vi "Main.vi"() -> ()   [LabVIEW 2018]
doc: "The myRIO Project template acquires acceleration data from the onboard accelerometer and displays the changes of acceleration values in a waveform chart."
uses:
  <vilib>/myRIO/Instrument Drivers/Utilities/Utilities.lvlib
  <vilib>/Platform/TimedLoop/XDataNode/XDataNode.xnode
  <vilib>/Platform/TimedLoop/XDataNode/nitl_modes.ctl
  <vilib>/Platform/TimedLoop/XDataNode/XDNodeRunTimeDep.lvlib
  <vilib>/Platform/TimedLoop/XDataNode/wakeup.ctl
  <vilib>/Platform/TimedLoop/XDataNode/timing_clust.ctl
  <vilib>/robotics/Steering/Steering Frame/NI_Robotics_Steering Frame.lvclass
  <vilib>/robotics/Steering/Wheel/NI_Robotics_Wheel.lvclass
  <vilib>/robotics/Steering/Wheel/Rotation Direction.ctl
  <vilib>/robotics/Steering/Wheel/Wheel Parameters.ctl
  <vilib>/addons/control/pid/NI_PID_pid.lvlib
  C:/Work/WRO/LidarCar/LidarCar/Operator Loop/Operator Loop Mode.ctl
  Operator Loop/Operator Loop Mode.ctl
  <vilib>/myRIO/Express VI/Onboard Devices/LED/LED Express VI.xnode
  <vilib>/myRIO/Instrument Drivers/Onboard IO/DIO/vis/Write.vi
  <vilib>/myRIO/Instrument Drivers/Onboard IO/DIO/DIO.lvlib
  <vilib>/myRIO/Common/Instrument Driver Framework/myRIO v1.0/DIO/typedefs/DIO Channels Enum.ctl
  <vilib>/myRIO/Common/Instrument Driver Framework/myRIO v1.0/DIO/typedefs/DIO Channels List.ctl
  <vilib>/myRIO/Common/Instrument Driver Framework/Utilities/typedefs/Generic FPGA Reference.ctl
  <vilib>/myRIO/Common/Instrument Driver Framework/Utilities/typedefs/myRIO v1.0 Reference.ctl
  <vilib>/myRIO/Common/Instrument Driver Framework/Utilities/typedefs/Hardware Version Enum.ctl
  <vilib>/myRIO/Common/Instrument Driver Framework/Utilities/typedefs/myRIO Generic Hardware Reference.ctl
  <vilib>/myRIO/Instrument Drivers/Onboard IO/DIO/typedefs/DIO Reference.ctl
  <vilib>/myRIO/Instrument Drivers/Onboard IO/DIO/vis/myRIO DIO Open.xnode
  <vilib>/myRIO/Common/Instrument Driver Framework/Utilities/vis/Is FPGA Ref Available.vi
  <vilib>/myRIO/Common/Instrument Driver Framework/myRIO v1.0/DIO/vis/myRIO v1.1 Open DIO.vi
  <vilib>/userdefined/High Color/nirio_resource_hc.ctl
  <vilib>/addons/control/pid/pid.llb/PID (DBL).vi
  <vilib>/Analysis/NI_AALPro.lvlib
  <vilib>/Analysis/coordinate.llb/2D Cartesian Coordinate Rotation (Scalar).vi
  <vilib>/myRIO/Express VI/Onboard Devices/Button/Button Express VI.xnode
  <vilib>/myRIO/Instrument Drivers/Onboard IO/DIO/vis/Read.vi
  <vilib>/myRIO/Instrument Drivers/Onboard IO/PWM/typedefs/PWM Configuration.ctl
  <vilib>/myRIO/Instrument Drivers/Onboard IO/PWM/PWM.lvlib
  <vilib>/myRIO/Common/Instrument Driver Framework/myRIO v1.0/PWM/typedefs/PWM Channels Enum.ctl
  <vilib>/myRIO/Instrument Drivers/Onboard IO/PWM/typedefs/PWM Reference.ctl
  <vilib>/myRIO/Instrument Drivers/Onboard IO/PWM/vis/Set Duty Cycle and Frequency.vi
  <vilib>/myRIO/Common/Instrument Driver Framework/myRIO v1.0/PWM/vis/myRIO v1.1 Open PWM.vi
  <vilib>/myRIO/Instrument Drivers/Onboard IO/PWM/vis/myRIO PWM Open.xnode
  <vilib>/myRIO/Express VI/Onboard IO/PWM/PWM Express VI.xnode
  <vilib>/vision/driver/NI_Vision_Acquisition_Software.lvlib
  <vilib>/myRIO/Express VI/Onboard IO/DI/DI Express VI.xnode
  <vilib>/myRIO/Express VI/Onboard IO/DO/DO Express VI.xnode
  <vilib>/robotics/Steering/Steering Frame/Create User Defined Steering Frame.vi
  <vilib>/robotics/Steering/Omnidirectional Wheel/Create Omnidirectional Wheel.vi
  <vilib>/robotics/Steering/Omnidirectional Wheel/NI_Robotics_Omnidirectional Wheel.lvclass
  <vilib>/robotics/Steering/Steering Frame/Apply Steering Frame Velocity to Motors.vi
  C:/Program Files (x86)/National Instruments/LabVIEW 2018/vi.lib/robotics/Steering/Wheel/NI_Robotics_Wheel.lvclass
  Type Definitions/Measurement Type.ctl
  Type Definitions/Acquisition Parameters.ctl
  <vilib>/userdefined/High Color/IMAQdx.ctl
panel:
  out "nowpos":dbl=-11.367150887839898
  out "OffsetZero":i32=-11
  in  "get over":bool
  out "B/DIO0 (Pin 11)":bool
  out "Lidar mid":i32=90
  in  "Light ON":bool
  in  "Load Image":bool
  in  "Select Image":string(combo)="A1"
  out "GoFarSec":u64
  out "min Distance":dbl=0.17274696726012956
  out "Image Out":T1(plugin-control)
  out "nearwall":bool
  out "Proc Down Color":i32=4
  in  "no get":bool
  in  "Enable US":bool=TRUE
  out "LD Range":dbl=119.77184676592617
  out "Block Face":dbl
  out "FX":dbl=518.7986455361987
  out "FXindex":i32=4
  out "FYindex":i32=14
  out "FXArr":dbl[](array[numeric])=[0.0, 518.7986455361987, 517.3027702585492, 515.9611019967892, 519.7944156608107]
  out "FYArr":dbl[](array[numeric])=[1569.0472275400712, 1569.0472275400712, 1561.3708676606448, 1566.6278937272687, 1557.2876598848363]
  out "FY":dbl=1569.0472275400712
  in  "Light Set":dbl=0.7
  out "Offset":dbl[](array[numeric])=[0.05, -3.061616997868383e-18]
  in  "Enable ND":bool
  in  "Set Test SubGoal":bool
  out "Put Counter":i32
  in  "Session In":T2="cam1"
  in  "Light":dbl
  out "ucolor":i32=4
  out "dcolor":i32=5
  in  "Color Disable":bool
  in  "URG-30LX":bool=TRUE
  in  "UBG-04FX Parameters":T3={"Starting Step"=44, "Ending Step"=725, "Cluster Count"=9, "Scan Interval"=0, "Number of Scans"=0, "Measurement Type"=enum."MS"}
  in  "Run Catch":bool
  in  "Get off/Put on":bool=TRUE
  in  "Test Catch":i16 min=0 max=3
  out "SubGoal":dbl[](array[numeric])=[0.588553326542981, 1.5637625506524007, 0.027695235097022965]
  in  "BL Range":dbl=106.0
  out "UltraSound":dbl=99.0
  in  "Set Z Offset":bool
  out "ODM Global Lidar":cluster{dbl[], dbl[]}[](graph)=[{[721.8291590825777], [795.7789827798357]}, {[0.0, 173.38729628759307, 225.66665610466003, 267.75647202793164, 307.78375775869426, 345.4796863667954, 386.0601693720772, 425.84303948753245, 461.38885484188586, 494.6121667989658, 530.892312288831, 564.3483818227398, 598.9442921444596, 631.7209869860719, 663.8971291981472, 695.8658767767539, 727.1715466499368, 758.8645020637247, 786.3860165375595, 804.3005854950422, 822.6493543934826, 841.0683200841246, 859.4613632147373, 878.918441734572, 896.3207994504536, 915.856172199784, 935.636054026129, 956.693854559551, 978.1414574666462, 997.7919082944074, 1021.5668180947448, 1129.0848273862223, 1140.3421474627507, 1167.0238039986898, 1197.8060920596474, 1237.6798928632963, 1274.67547579493, 1313.6442770102278, 1351.7890598592828, 1601.7296724745213, 1701.59915067344, 1790.471940105315, 1890.3533021616595, 1975.681444325002, 2080.8834474418536, 2199.916399964641, 2288.3422835710217, 2269.044100856724, 2269.913362880439, 2275.262737598881, 2273.0619560851524, 2271.883597560387, 2273.867229333762, 2276.270813184838, 2283.1501466095037, 2281.7136074144396, 2280.8814360333404, 2287.701288915185, 2057.221659783369, 2055.6828792476545, 2062.1389602013965, 2058.6161638397925, 2055.0754422563373, 2156.1814882136705, 2091.396440925394, 1945.0381394296392, 1934.4975767345456, 1929.5528957285972, 1928.0192875117154, 1928.679460770824, 1934.7695441247085, 2273.4555279831993, 2244.567273948284, 1420.8784222522072, 1338.2032680954792, 1274.032736829724, 1215.8750320799377, 1165.7538524389452, 1130.9140787661042, 1116.611145793328, 1108.8419935326024, 1098.073782898878, 1090.3710419336774, 1087.2408194244206, 1072.1815861120838, 1064.3437362068323, 1052.1947093007082, 1043.6027163222507, 1034.9198885950275, 1020.989821141792, 1147.510042165152, 1185.4766822006893, 1123.9684076830076, 1063.326429163897, 1003.3034354850358, 942.6873919372472, 883.4901954196058, 823.9725320994982, 764.5128057343941, 705.1514377393997, 645.8853239946892, 585.7997376242854, 526.0621283065328, 464.34896817814956, 404.24666324255236, 342.0883282079875, 277.0716342023713, 212.69592369267963], [0.0, -1.1322564017730496, 4.966756080453739, 0.5077440499308005, -4.454468226445895, -11.021670601286585, -9.596364902480591, -6.2440935839171, -9.378372326349291, -16.613562940879945, -12.932345500497807, -15.388120696622703, -10.61269028937555, -10.276165299446717, -10.586494828388973, -9.608611783836272, -13.34567042737981, -7.855848584257861, 328.8560921706781, 331.40708435844897, 327.682033403894, 326.68504208099455, 327.41527128271883, 323.9888902290291, 331.08814597563986, 330.199640851444, 330.14966222571655, 328.1530339444062, 327.11711529750204, 331.58647253289155, 328.92067367243607, 182.64222973992665, 216.23913279752037, 224.17363585313913, 227.71482426419658, 221.92474990792795, 222.95568299997052, 224.59211265082112, 229.84383762917457, 46.1196506252172, 19.290037227608405, 10.236768574542058, 0.6806810112642081, 8.771460166297727, 11.11763649590324, 13.887670225470854, 40.869048984587245, 121.85683290565059, 190.46182338990178, 255.40765812456652, 321.33540980144414, 385.21578219972656, 446.9407541050027, 507.6435863509478, 566.9883190305765, 627.0796755525192, 686.5140152469784, 745.3526744488408, 801.9668274705773, 852.0483763075719, 902.9259095939335, 953.3797430047575, 1004.0687823188368, 1077.182165623156, 1117.7495796008423, 1130.0011651866287, 1176.7036525019564, 1225.956066917477, 1277.770631563482, 1332.2729192505776, 1391.7418162789627, 1645.3317728813229, 1706.9758198210902, 1225.5086611026113, 1201.9471543380675, 1185.1985794784985, 1167.3981152418305, 1151.1958156005373, 1145.277200975239, 1158.7274049891116, 1180.048820376938, 1198.942700206554, 1223.2944316784685, 1256.8697159243388, 1274.5279241498613, 1306.6412141486715, 1334.377137334104, 1373.7982904308146, 1419.8389496097002, 1460.39373731479, 1958.9040004476574, 2284.203937575801, 2288.1943216415884, 2292.6275978401427, 2297.5929521065086, 2294.2073833976106, 2300.379784341795, 2301.2264246197224, 2302.7349037113363, 2298.9104379767673, 2294.7558697296113, 2296.21136858921, 2291.316732701449, 2293.83689238431, 2285.0809925529366, 2281.5956696474964, 2283.099714055563, 2278.034076178987]}, {[0.0, 0.0, 2300.0, 2300.0, 0.0], [0.0, 2300.0, 2300.0, 0.0, 0.0]}, {[115.0, 115.0, 2185.0, 2185.0, 115.0], [115.0, 2185.0, 2185.0, 115.0, 115.0]}, {[1.2743751839684945], [1.349012436815834]}, {[1.1606747746939823], [1.7455328863903905]}, {[903.9764173161522, 1240.4369436227526, 2170.0754422563373, -115.0, 2043.0192875117154, -115.0, -115.0], [216.58647253289155, 114.84383762917457, 903.0178048947071, 0.0, 1260.8714907327958, 0.0, 0.0]}, {[436.58676528880187, 903.9378283810288, 1240.4213885973015, 2167.4413707572576, 2041.974666138485], [796.903102586175, 217.61848380592934, 113.82095487507502, 902.8249826773058, 1259.8777188454835]}]
  out "Odometry Data":dbl[](array[numeric])=[0.5140081874058262, 1.5687256004107921, 0.036230187244589505]
  in  "Reset Start POS":bool
  in  "Set Start POS":bool
  out "X Find":dbl=519.7944156608107
  out "XL Dots":dbl=36.0
  out "XR Dots":dbl=2.0
  out "XR Find":dbl=513.9748126879588
  out "SEC":u64
  out "MIN":u64
  out "Angle Find":dbl=0.017453292519943295
  out "Y Find":dbl=1551.5711689987047
  out "XL Find":dbl=525.6140186336626
  out "Down Color":i32
  out "Up Color":i32
  out "Right Block":bool
  out "Left Block":bool
  out "Proc Time":i16=173
  out "Proc Index":i16=25
  in  "Proc  VAL B":i32
  in  "Proc  VAL A":i32
  in  "Proc CMD":i16=99
  out "Block Array":dbl[][](array[numeric])
  out "Proc Finish":bool=TRUE
  out "Proc Catch Index":i16
  out "Proc Block Index":i16
  out "Block Color":i16[][](array[numeric])
  out "Catch Color":i16[](array[numeric])
  in  "Timer Run":bool
  out "Z offset":dbl
  in  "-X":bool
  in  "+X":bool
  in  "-Y":bool
  in  "+Y":bool
  out "Sensor z":dbl=-0.7583617520109639
  in  "Z Sensor resource":refnum<visa-resource-name>="ASRL2::INSTR"
  in  "QR_CAM":bool=TRUE
  in  "Set SubGoal":bool
  in  "RC servo resource":refnum<visa-resource-name>="ASRL1::INSTR"
  out "Start Out Point":dbl[](array[numeric])=[0.5218091856466301, 1.3965735001255937]
  out "Block Fix array":dbl[](array[numeric])
  out "Target Distance":dbl=0.17274696726012956
  in  "PLAY":bool
  out "Start POS":dbl[](array[numeric])=[0.5259977631915781, 1.1566100532880597, -3.12413936106985]
  out "Start Front":dbl[](array[numeric])=[0.5187986455361987, 1.569047227540071, -3.12413936106985]
  in  "Block Find":bool
  in  "Show Lidar":bool
  in  "Robot Mode:":T5(ring)
  in  "max speed":dbl=0.67
  in  "inner threshold":dbl=0.2
  in  "outer threshold":dbl=0.5
  out "LIDAR data":cluster{dbl[], dbl[]}[](graph)
  out "VY History 2":dbl(graph)
  out "Heading History 2":dbl(graph)
  in  "Show VFH":bool
  out "Distance":i32[](array[numeric])
  out "Lidar Data":cluster{"angles (deg)":dbl[], "distances":dbl[]}(graph)={"angles (deg)"=[0.0, 433.8787272960038, 477.8933242300426, 527.1098060603185, 577.9196711836571, 638.569011724086, 712.0914573803195, 804.449757554414, 947.9078296932058, 1156.1704640673584, 1436.9407341066774, 1782.6178607501113, 443.13319277072446, 436.4011066877488, 428.963246529249, 428.85299241451406, 428.0814780693609, 436.59511206667196, 432.4776560401959, 429.6823946054481, 435.9780172673052, 437.56439930894794, 429.758975005734, 431.7298029202177, 428.18120387395703, 232.04054624122062, 174.89018459887424, 171.36933696908324, 152.11493483575714, 138.38064371099495, 125.76279949489856, 118.20964770339404, 109.94438198650472, 103.29713074135779, 95.98446041890367, 88.79774026449425, 82.41822688750861, 75.5184469259805, 68.80732906562578, 64.0039047725061, 58.16398223480165, 54.49999999999999, 47.492681073161364, 43.051109680829505, 39.86912949481099, 36.55353085362063, 31.179628134406673, 27.54948843628049, 23.138409544725345, 19.127875555233857, 16.257552369506364, 11.74735729980464, 8.235145679706214, 4.814907974350832, 1.2042427925636885, -2.460633140940076, -6.344103535323877, -10.034732473694731, -13.201321223188495, -17.130139396261864, -20.3041640219781, -25.10544737494451, -28.764532772630385, -34.71591336031218, -45.94912225121969, -110.22563027354184, -185.31896120176154, -239.53369765032343, -265.3611116739901, -461.85390169274285, -472.10476545045714, -477.8777217718457, -480.8581294893997, -485.1196896101722, -484.266579130126, -487.4515773202573, -484.93667582394033, -486.49337187206373, -483.95730286540066, -492.0033346073434, -489.67640876660056, -492.76845475334557, -489.3981635170621, -492.8115652550238, -492.4720886398095, -491.9968847640253, -488.61594681947446, -490.91570425251484, -493.338533040738, -492.98639076983807, -490.8069174109227, -490.76520638003615, -495.91085393218157, -488.3298424949866, -490.95793483883745, -490.8317465629986, -494.93802592634734, -491.29381631192706, -489.8774364757368, -488.67768905928546, -490.5971872157819, -487.7925422759795, -492.7902913399083, -493.0014998412093, -488.55382481063214, -486.91972892350634, -469.9613165631287, -436.7721049929968, 0.0], "distances"=[0.0, -250.4999999999999, -251.43184097556016, -251.41848053604448, -248.29388566570398, -245.12367748898538, -241.72247790797735, -238.2888742065911, -240.7379205823552, -245.7516185465913, -246.91157661187788, -234.68609361165238, -40.71822030521407, -22.870812878166458, -5.615436500106674, 11.229910824077672, 28.057942439731367, 45.887995374499866, 62.70627581014535, 79.63692464006853, 98.65175345461108, 117.2450274314419, 133.44370873900692, 152.88354152906706, 170.82697869203457, 103.31110734125329, 86.24629459270524, 93.04595825062364, 90.4988762356382, 89.86544077747949, 88.880359265734, 90.70545292229937, 91.4397772832236, 93.0091542838813, 93.50392161878514, 93.57329386058511, 93.97997593487217, 93.25751537483652, 92.14418845947198, 93.12625931428776, 92.18433256573309, 94.39676901250382, 90.26873902123027, 90.25852843498606, 92.79791222503873, 95.22520350271458, 91.85222256102526, 93.00551428221473, 91.10770551243492, 89.98957926751012, 94.61338166957546, 89.23003752364293, 89.62244348171956, 91.8739171974208, 91.99211813680864, 93.96778854770238, 96.79231555414454, 95.47410195535423, 91.04792758740966, 92.42596131101173, 89.73149348678317, 93.69480515003963, 92.6369346123471, 98.03471507358655, 115.1723845561186, 247.57081902114484, 375.7896787021964, 441.1661905563066, 446.0319275692539, 711.1926416177196, 668.0127921222534, 622.7823721286196, 578.1690577192416, 538.7799984711108, 497.11354873671013, 462.5742748662027, 425.2780507395445, 393.95456479719826, 361.38805874467806, 338.1445234441252, 308.96280471513904, 284.50000000000006, 257.4848297397867, 235.0590588573292, 211.5827070219672, 188.85990941037318, 165.86276409643145, 145.41585648840845, 125.29202615175753, 104.78749217215065, 84.33605291681421, 64.6104651489256, 45.567806094374454, 25.5922826027996, 6.426991425530077, -12.852881619165652, -32.439952098151, -51.63706085422075, -71.02884788563368, -90.57105616959733, -111.01080981581498, -130.70361777677303, -153.01545268739454, -174.58098737926213, -194.9132121301739, -216.7906307594014, -231.7592736747566, -237.1479038490254, 0.0]} caption="Global Lidar Data"
  out "Lidar Array Size":dbl=107.0
  out "Angle":dbl[](array[numeric])=[-120.0, -117.75, -115.5, -113.25, -111.0, -108.75, -106.5, -104.25, -102.0, -99.75, -97.5, -95.25, -93.0, -90.75, -88.5, -86.25, -84.0, -81.75, -79.5, -77.25, -75.0, -72.75, -70.5, -68.25, -66.0, -63.75, -61.5, -59.25, -57.0, -54.75, -52.5, -50.25, -48.0, -45.75, -43.5, -41.25, -39.0, -36.75, -34.5, -32.25, -30.0, -27.75, -25.5, -23.25, -21.0, -18.75, -16.5, -14.25, -12.0, -9.75, -7.5, -5.25, -3.0, -0.75, 1.5, 3.75, 6.0, 8.25, 10.5, 12.75, 15.0, 17.25, 19.5, 21.75, 24.0, 26.25, 28.5, 30.75, 33.0, 35.25, 37.5, 39.75, 42.0, 44.25, 46.5, 48.75, 51.0, 53.25, 55.5, 57.75, 60.0, 62.25, 64.5, 66.75, 69.0, 71.25, 73.5, 75.75, 78.0, 80.25, 82.5, 84.75, 87.0, 89.25, 91.5, 93.75, 96.0, 98.25, 100.5, 102.75, 105.0, 107.25, 109.5, 111.75, 114.0, 116.25, 118.5]
  in  "URG-04LX Resource":refnum<visa-resource-name>="ASRL3::INSTR"
  in  "URG-30LX Parameters":T3={"Starting Step"=60, "Ending Step"=1020, "Cluster Count"=9, "Scan Interval"=0, "Number of Scans"=0, "Measurement Type"=enum."MS"}
  out "Now POS":cluster{"X":dbl, "Y":dbl, "Angle":dbl}={"X"=514.0081874058262, "Y"=1568.7256004107921, "Angle"=2.075836820083688}
  in  "Enable":bool=TRUE caption="Enable Motor"
  in  "X Velocity (m/s)":dbl(slide) min=-1.0 max=1.0 scale=-0.5..0.5
  in  "Y Velocity (m/s)":dbl(slide) min=-1.0 max=1.0 scale=-0.5..0.5
  in  "Heading(rad)":dbl(slide) min=-10.0 max=10.0 scale=10.0..-10.0
  out "X Velocity Feedback":dbl(slide) scale=-0.5..0.5
  out "Y Velocity Feedback":dbl(slide)=-0.0 scale=-0.5..0.5
  out "Angular Velocity Feedback":dbl(slide) scale=10.0..-10.0
  in  "stop":bool=TRUE
  in  "PID gains":T6={"proportional gain (Kc)"=0.11, "integral time (Ti, min)"=0.001, "derivative time (Td, min)"=0.0} {"derivative time (Td, min)" format="%.5f"; "integral time (Ti, min)" format="%.3f"; "proportional gain (Kc)" format="%.3f"}
  out "ENC Val. mm":T7={"Numeric Control"=-13.769011552061516, "Numeric Control"=3.3657583793928145, "Numeric Control"=-3.059780344902559}
  in  "Reset Counter":bool
  in  "Encoder PPR":dbl=24.0
  in  "Gear Ratio":i32=64
  in  "R(mm)":dbl=37.4
  out "error out":errorcluster={"status"=FALSE, "code"=1073676294, "source"="VISA Read in URG-04LX-UG01 Read Measurement Data.vi->Main.vi"}
  # "0:x\n1:Green \n2:Red \n3:Yellow\n4:Blue\n5:Orange"
  # "2    0          1     3\n\\     /           \\     /"
  # "下      上        不處理"
  # "讀取QR CODE"
  # "執行程式"
  # "不看顏色,使用預設"
  # "不取方塊"
  # "設定Z軸偏移"
  # "地圖BX,地圖BY,座標Xmm,座標Ymm,下顏色,上顏色,FXm,FYm,FZrag,看到的次數(最多100)"
  # "顯示行走圖"
  # "按下使用遠距光達"
  # "用來修正世界座標\n及偏移值"
  # "測試取放方塊\n1.Block Correction -> Idle\n2.Set SubGoal\n3.選擇爪子\n4.選擇拿起(Get)或放下(Put,按下)\n5.按下Run Catch"
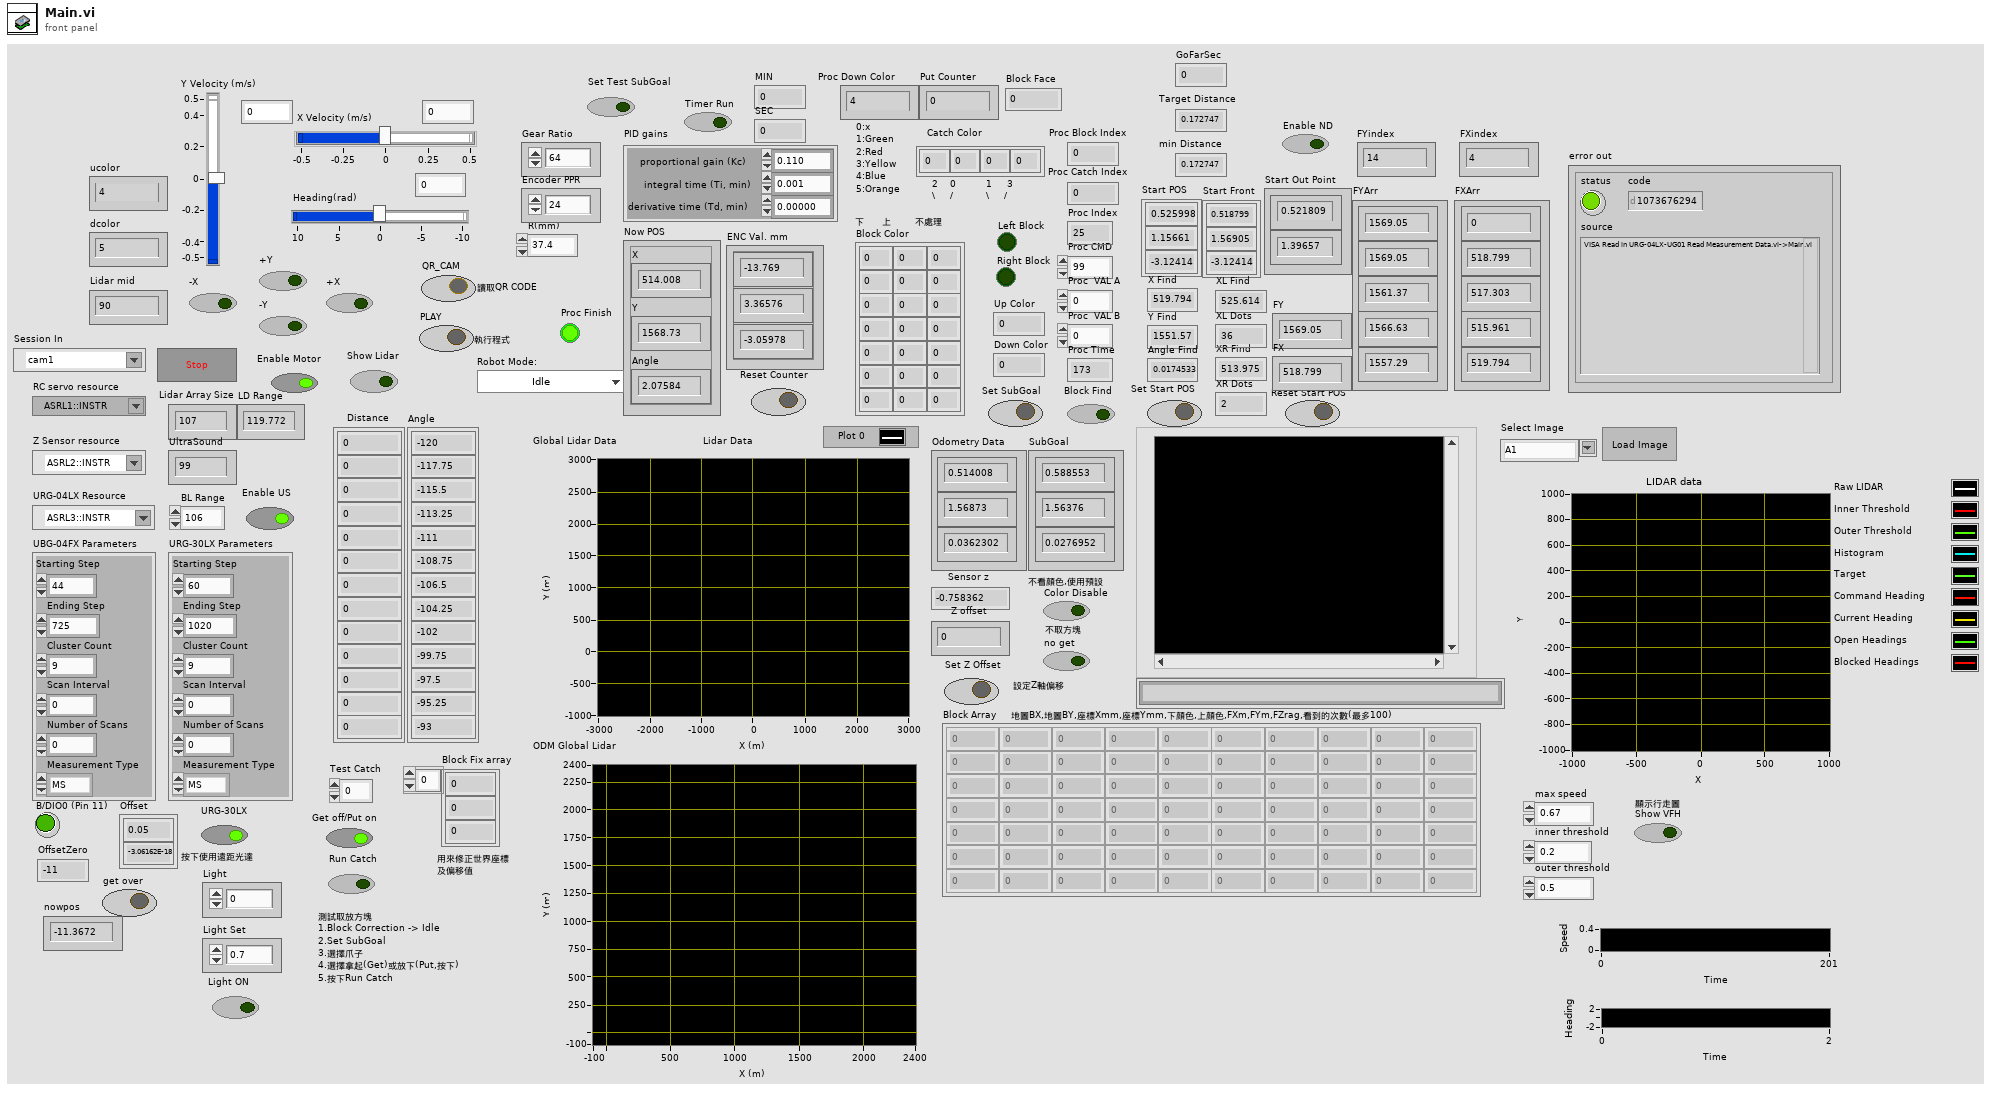
[diagram p1: front panel]
types:
  T1 = typedef "IMAQ Image.ctl" = refnum<image>
  T2 = typedef "IMAQdx.ctl" = refnum<k21>
  T3 = typedef "Acquisition Parameters.ctl" = cluster{"Starting Step":i32, "Ending Step":i32, "Cluster Count":i32, "Scan Interval":i32, "Number of Scans":i32, "Measurement Type":T4}
  T4 = typedef "Measurement Type.ctl" = enum16{"MD", "MS"}
  T5 = enum16{"Idle", "Tele-Op", "Path Following", "Go Target", "Wall Correction", "Positioning", "Block Correction", "Get Color", "WhereGo", "Home Correction", "RC Control", "MoveTarget", "moveblock", "hands up", "hands down", "readQR"}
  T6 = cluster{"proportional gain (Kc)":dbl, "integral time (Ti, min)":dbl, "derivative time (Td, min)":dbl}
  T7 = cluster{"Numeric Control":dbl, "Numeric Control":dbl, "Numeric Control":dbl}
  T8 = typedef "PWM.lvlib/PWM Reference.ctl" = cluster{"myRIO Reference":T9, "PWM Channels Enum":T13, "PWM Configuration":T14}
  T9 = typedef "myRIO Generic Hardware Reference.ctl" = cluster{"myRIO Model":T10, "myRIO Hardware Reference":T11}
  T10 = typedef "Hardware Version Enum.ctl" = enum16{"Unknown", "myRIO-1900", "myRIO-1950", "roboRIO", "NI ELVIS RIO CM", "ELVIS III"}
  T11 = typedef "myRIO v1.0 Reference.ctl" = cluster{"Generic FPGA Reference":T12, "Allow multiple opens":bool}
  T12 = typedef "Generic FPGA Reference.ctl" = refnum<k20>
  T13 = typedef "PWM Channels Enum.ctl" = enum16{"Not Connected", "C/PWM0", "C/PWM1", "A/PWM0", "A/PWM1", "A/PWM2", "A/PWM3", "A/PWM4", "A/PWM5", "A/PWM6", "A/PWM7", "A/PWM8", "A/PWM9", "A/PWM10", "A/PWM11", "A/PWM12", "A/PWM13", "A/PWM14", "A/PWM15", "A/PWM16", "A/PWM17", "A/PWM18", "A/PWM19", "B/PWM0", "B/PWM1", "B/PWM2", "B/PWM3", "B/PWM4", "B/PWM5", "B/PWM6", "B/PWM7", "B/PWM8", "B/PWM9", "B/PWM10", "B/PWM11", "B/PWM12", "B/PWM13", "B/PWM14", "B/PWM15", "B/PWM16", "B/PWM17", "B/PWM18", "B/PWM19", "PWM/PWM0", "PWM/PWM1", "PWM/PWM2", "PWM/PWM3", "PWM/PWM4", "PWM/PWM5", "PWM/PWM6", "PWM/PWM7", "PWM/PWM8", "PWM/PWM9"}
  T14 = typedef "PWM.lvlib/PWM Configuration.ctl" = cluster{"Frequency":dbl, "Duty Cycle":dbl}
  T15 = typedef "nirio_resource_hc.ctl" = tag
  T16 = typedef "DIO.lvlib/DIO Reference.ctl" = cluster{"myRIO Reference":T9, "DIO Channels List":T17}
  T17 = typedef "DIO Channels List.ctl" = T18[]
  T18 = typedef "DIO Channels Enum.ctl" = enum16{"Not Connected", "C/DIO0", "C/DIO1", "C/DIO2", "C/DIO3", "C/DIO4", "C/DIO5", "C/DIO6", "C/DIO7", "A/DIO0", "A/DIO1", "A/DIO2", "A/DIO3", "A/DIO4", "A/DIO5", "A/DIO6", "A/DIO7", "A/DIO8", "A/DIO9", "A/DIO10", "A/DIO11", "A/DIO12", "A/DIO13", "A/DIO14", "A/DIO15", "A/DIO16", "A/DIO17", "A/DIO18", "A/DIO19", "B/DIO0", "B/DIO1", "B/DIO2", "B/DIO3", "B/DIO4", "B/DIO5", "B/DIO6", "B/DIO7", "B/DIO8", "B/DIO9", "B/DIO10", "B/DIO11", "B/DIO12", "B/DIO13", "B/DIO14", "B/DIO15", "B/DIO16", "B/DIO17", "B/DIO18", "B/DIO19", "LED0", "LED1", "LED2", "LED3", "Button0", "DIO/DIO0", "DIO/DIO1", "DIO/DIO2", "DIO/DIO3", "DIO/DIO4", "DIO/DIO5", "DIO/DIO6", "DIO/DIO7", "DIO/DIO8", "DIO/DIO9", "SPI/CS0", "SPI/CS1", "SPI/CS2", "SPI/CS3", "LED RADIO (Green)", "LED RADIO (Red)", "LED COMM (Green)", "LED COMM (Red)", "LED MODE (Green)", "LED MODE (Red)"}
  T19 = typedef "Operator Loop Mode.ctl" = enum16{"Idle", "Tele-Op", "Path Following", "Go Target", "Wall Correction", "Positioning", "Block Correction", "Get Color", "WhereGo", "Home Correction", "RC Control", "MoveTarget", "moveblock", "hands up", "hands down", "readQR"}
  T20 = typedef "XDNodeRunTimeDep.lvlib/timing_clust.ctl" = cluster{"Expected End [f-1]":u64, "Actual End [f-1]":u64, "Finished Late? [f-1]":bool, "Expected End [i-1]":u64, "Actual End [i-1]":u64, "Finished Late? [i-1]":bool, "Expected Start [i]":u64, "Actual Start [i]":u64, "Expected Start [f]":u64, "Actual Start [f]":u64, "Source Name":string, "Structure Name":string, "Period":i64, "Deadline":i64, "Offset":i64, "Start":i64, "Priority":i32, "Timeout":i32, "Mode":T21, "Wakeup Reason":T22, "Error":errorcluster, "Source Type":string, "Secondary Source Type":string, "Global End Time":u64, "Global Start Time":u64, "Frame Duration":u64, "Iteration Duration":u64, "Assigned CPU":i32, "I/O Scan Engine Mode":u32}
  T21 = typedef "XDNodeRunTimeDep.lvlib/nitl_modes.ctl" = enum32{"No Change", "Process missed periods, maintain original phase", "Discard missed periods, maintain original phase", "Process missed periods, ignore original phase", "Discard missed periods, ignore original phase"}
  T22 = typedef "XDNodeRunTimeDep.lvlib/wakeup.ctl" = enum32{"Normal", "Aborted", "Asynchronous wakeup", "Timing source error", "Timed loop error", "Timeout"}
  T23 = cluster{"Speed A(mm/s)":dbl, "Speed B(mm/s)":dbl, "Speed C(mm/s)":dbl}
  T24 = typedef "NI_Robotics_Wheel.lvclass/Rotation Direction.ctl" = u16
  T25 = typedef "NI_Robotics_Wheel.lvclass/Wheel Parameters.ctl" = cluster{"wheel radius":dbl, "gear ratio":dbl, "forward rotation direction":T24}
  T26 = cluster{"StartUp Cnt. A":dbl, "StartUp Cnt. B":dbl, "StartUp Cnt. C":dbl}
  T27 = cluster{"Numeric":dbl, "Numeric":dbl, "Numeric":dbl}
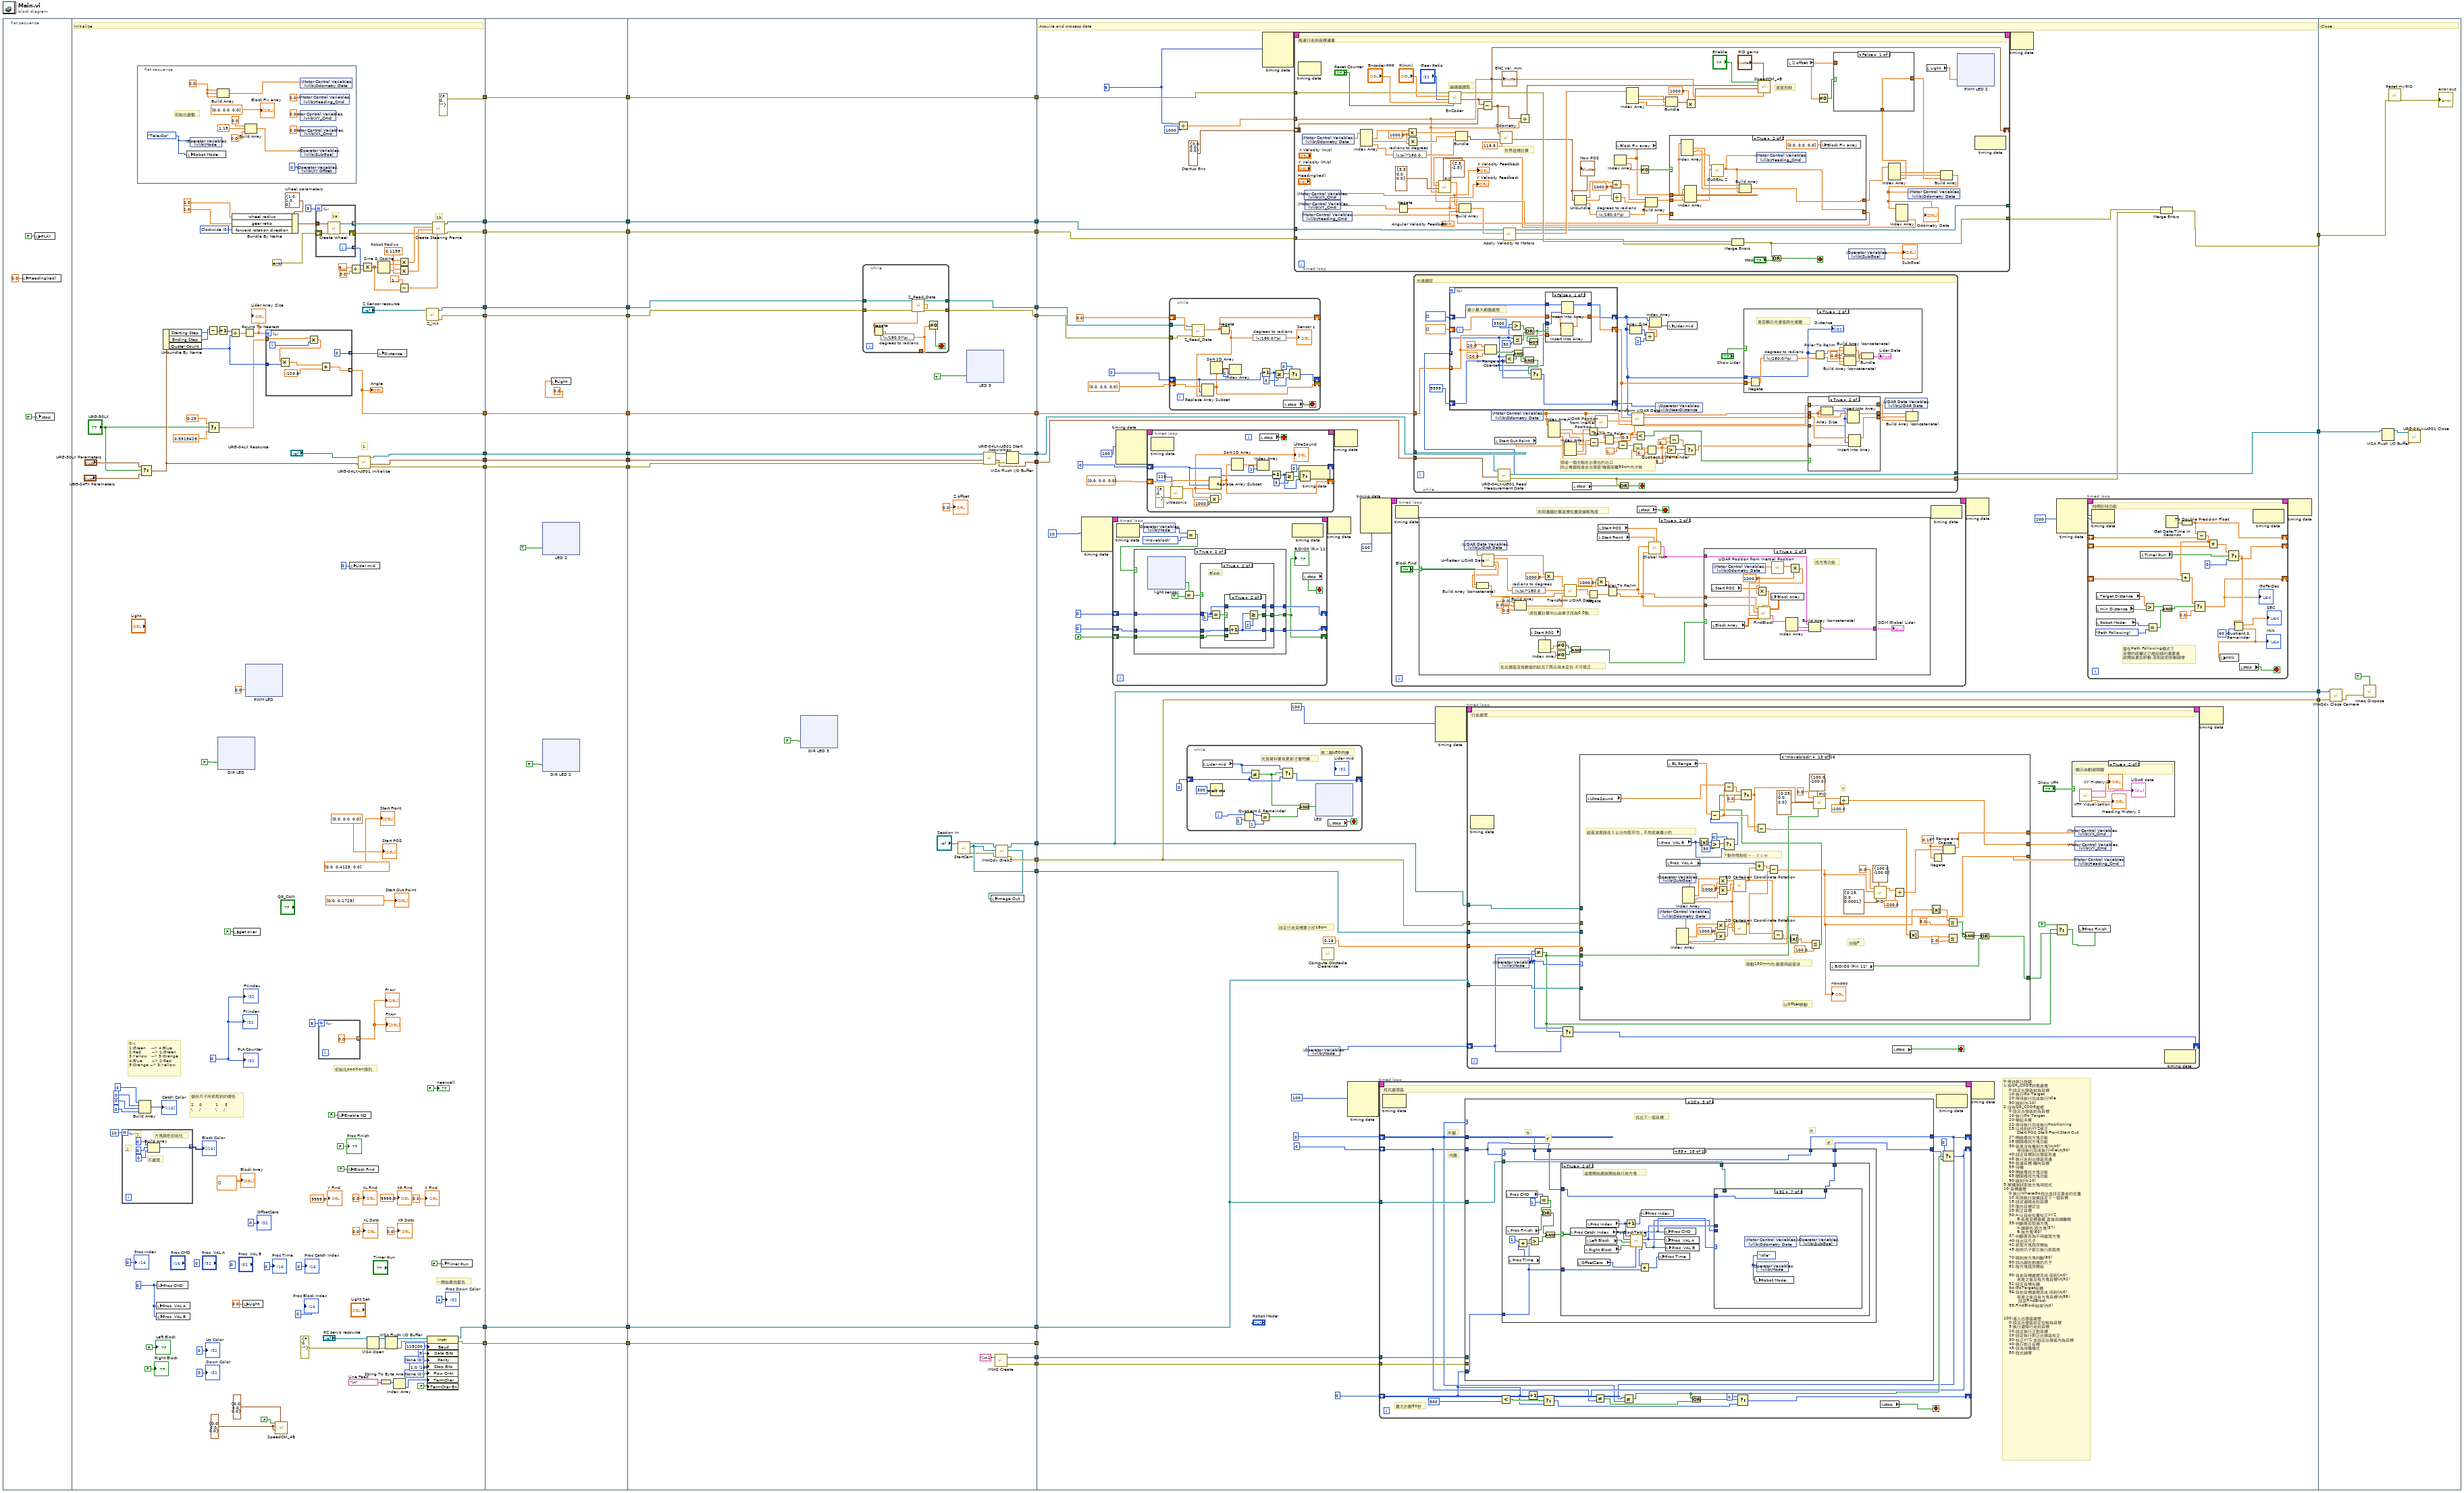
[diagram p0: block diagram]
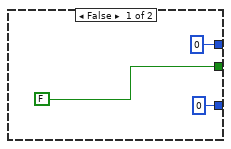
[diagram p2: hidden frame]
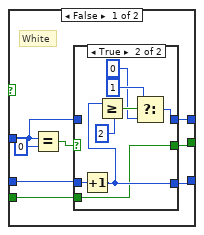
[diagram p3: hidden frame]
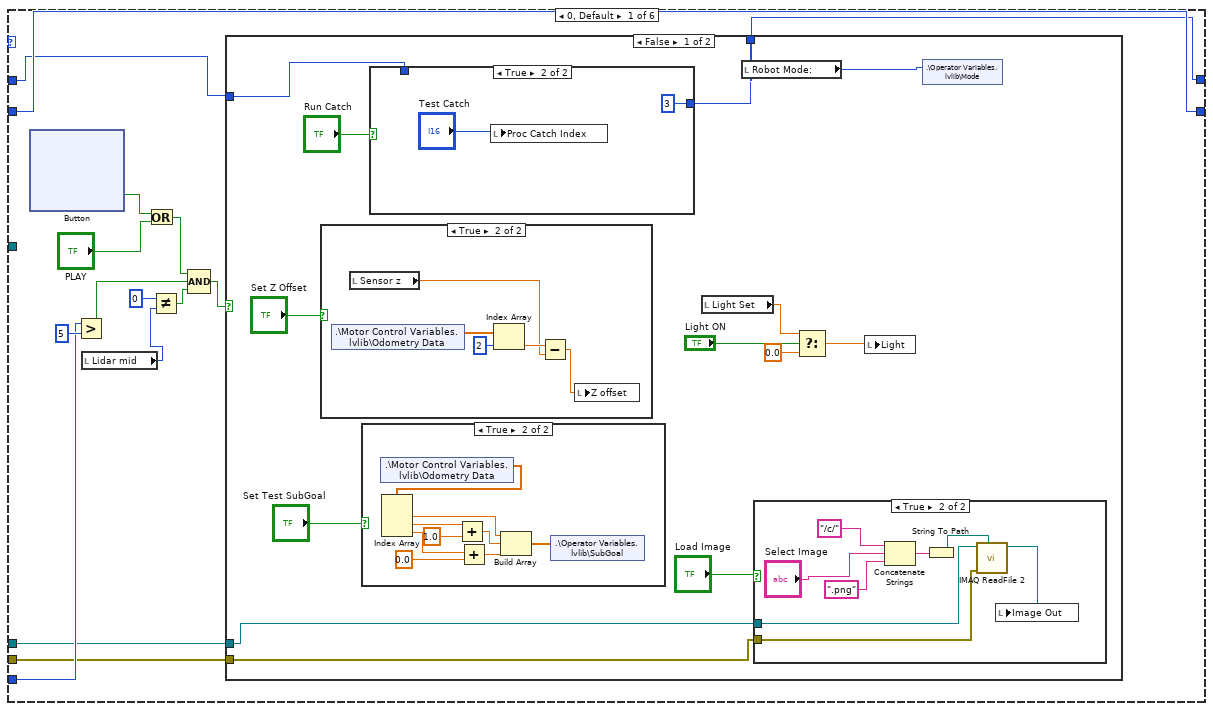
[diagram p6: hidden frame]
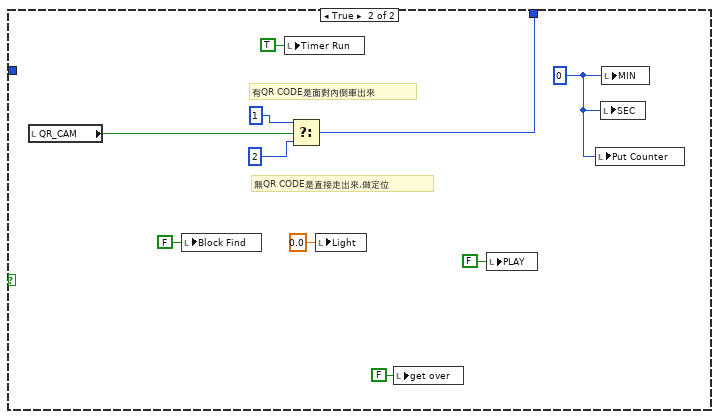
[diagram p11: hidden frame]
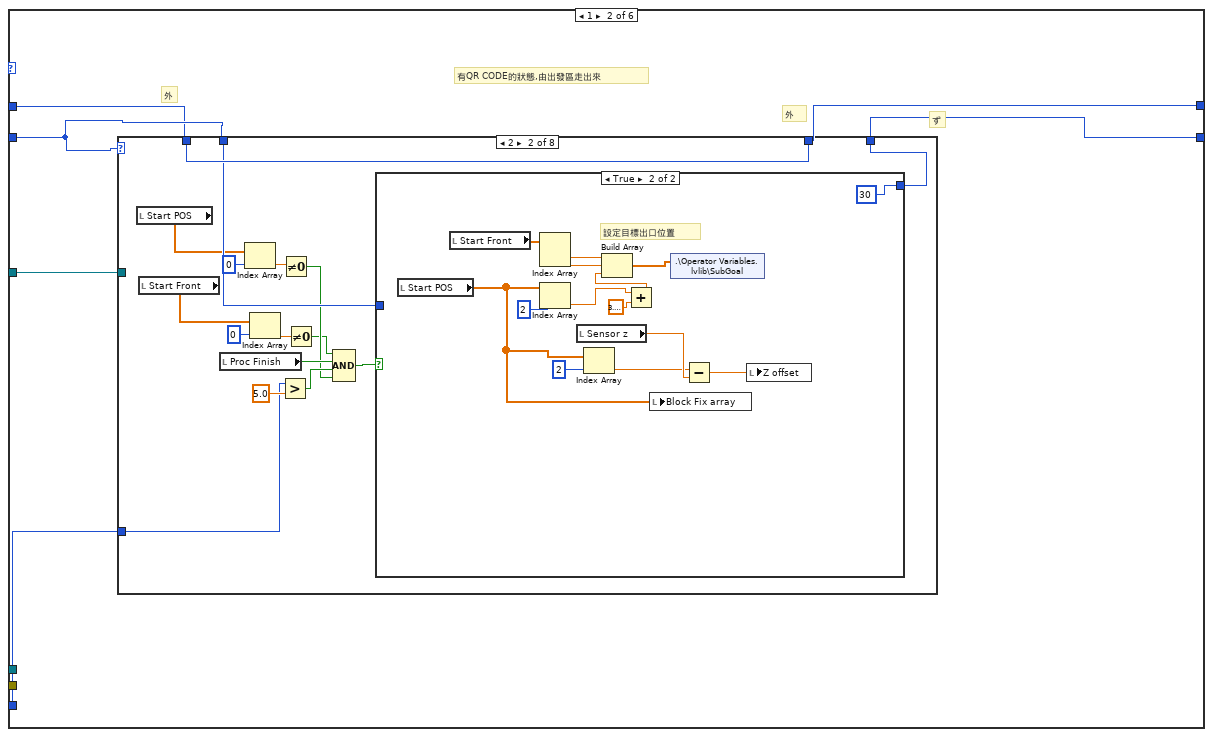
[diagram p12: hidden frame]
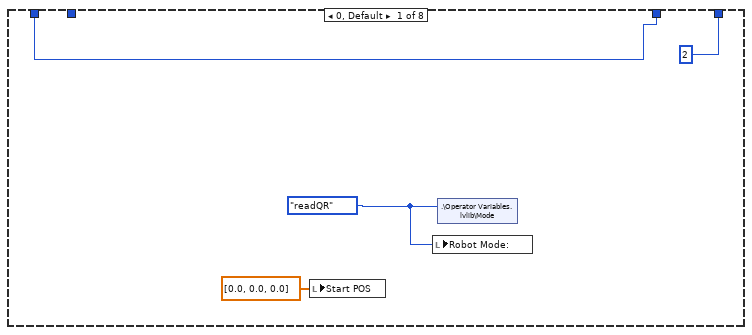
[diagram p13: hidden frame]
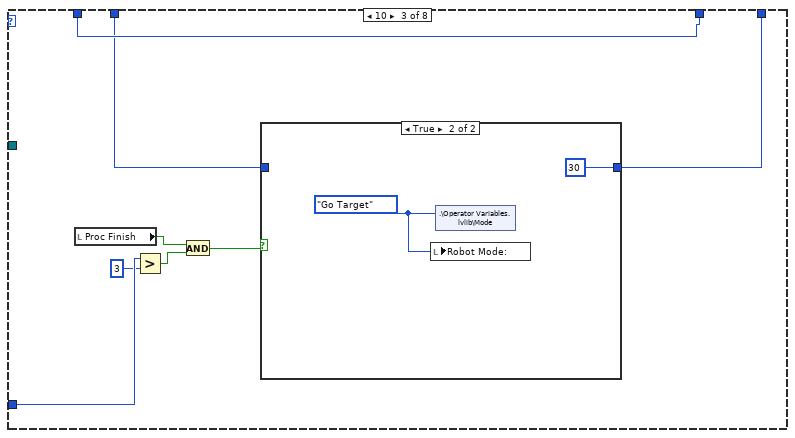
[diagram p15: hidden frame]
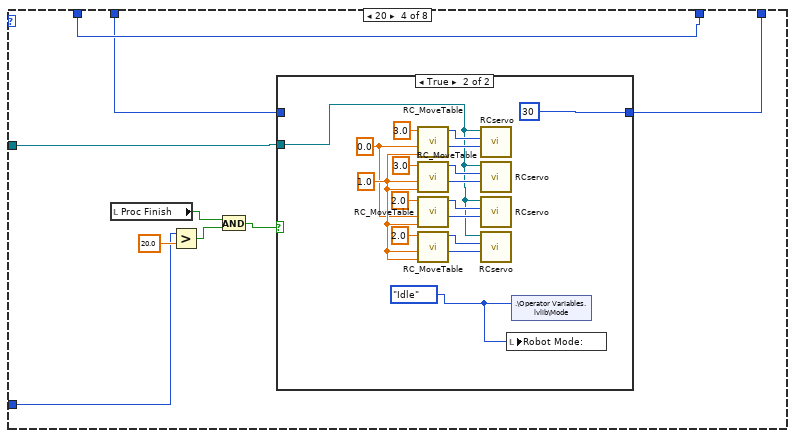
[diagram p17: hidden frame]
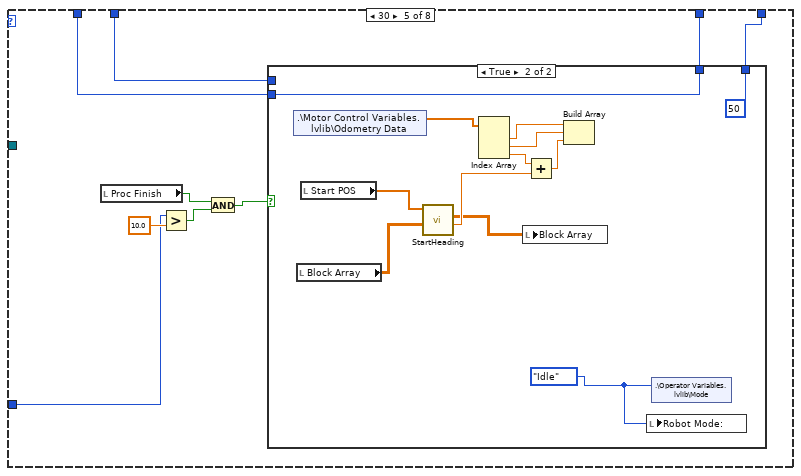
[diagram p19: hidden frame]
diagram:
  n1 = flat-sequence {
    tunnel: [errorcluster {"status"=FALSE, "code"=0, "source"=""} ("error in (no error)")] -> w25
    tunnel: [w130] -> w23
    tunnel: [w129] -> w21
    tunnel: [w120] -> w19
    tunnel: [w119] -> w17
    tunnel: [w118] -> w15
    tunnel: [w117] -> w13
    tunnel: [w101] -> w11
    tunnel: [w100] -> w9
    tunnel: [w98] -> w7
    tunnel: [w97] -> w5
    tunnel: w25 -> [w266]
    tunnel: [w266] -> w24
    tunnel: w23 -> [w265]
    tunnel: [w265] -> w22
    tunnel: w21 -> [w264]
    tunnel: [w264] -> w20
    tunnel: w19 -> [w263]
    tunnel: [w263] -> w18
    tunnel: w17 -> [w262]
    tunnel: [w262] -> w16
    tunnel: w15 -> [w261]
    tunnel: [w261] -> w14
    tunnel: w13 -> [w260]
    tunnel: [w260] -> w12
    tunnel: w11 -> [w259]
    tunnel: [w259] -> w10
    tunnel: w9 -> [w258]
    tunnel: [w258] -> w8
    tunnel: w7 -> [w257]
    tunnel: [w257] -> w6
    tunnel: w5 -> [w256]
    tunnel: [w256] -> w4
    tunnel: w24 -> [w366]
    tunnel: [w366] -> w39
    tunnel: w22 -> [w365]
    tunnel: [w365] -> w38
    tunnel: w20 -> [w364]
    tunnel: [w364] -> w37
    tunnel: w18 -> [w363]
    tunnel: [w363] -> w36
    tunnel: w16 -> [w358]
    tunnel: [w362] -> w35
    tunnel: w14 -> [w357]
    tunnel: w12 -> [w356]
    tunnel: [w359] -> w34
    tunnel: w10 -> [w354]
    tunnel: [w354] -> w33
    tunnel: w8 -> [w353]
    tunnel: [w353] -> w32
    tunnel: w6 -> [w350]
    tunnel: w4 -> [w352]
    tunnel: [w349] -> w31
    tunnel: [w351] -> w30
    tunnel: [w343] -> w29
    tunnel: [w342] -> w28
    tunnel: [w345] -> w3
    tunnel: [w339] -> w2
    tunnel: [w338] -> w1
    tunnel: w39 -> [w498]
    tunnel: w38 -> [w494]
    tunnel: w37 -> [w479]
    tunnel: w36 -> [w487]
    tunnel: w35 -> [w452]
    tunnel: [w470] -> w41
    tunnel: w34 -> [w451]
    tunnel: [w483] -> w40
    tunnel: w33 -> [_]
    tunnel: w32 -> [w463]
    tunnel: w31 -> [w472]
    tunnel: w30 -> [w473]
    tunnel: w29 -> [w459]
    tunnel: w28 -> [w460]
    tunnel: [w460] -> w27
    tunnel: [w459] -> w26
    tunnel: w3 -> [w456]
    tunnel: w2 -> [w454]
    tunnel: w1 -> [w453]
    tunnel: w41 -> [w2689]
    tunnel: w40 -> [w2690]
    tunnel: w27 -> [w2685]
    tunnel: w26 -> [w2684]
    frame #0 {
      n2 = local write "Heading(rad)"(0.0 ("Heading(rad)")) -> ()
      n3 = local write "PLAY"(FALSE ("PLAY")) -> ()
      n4 = local write "stop"(FALSE ("stop")) -> ()
    }
    frame #1 {
      w52 = T23 {"Speed A(mm/s)"=0.0, "Speed B(mm/s)"=0.0, "Speed C(mm/s)"=0.0} ("Speed Now")
      w61 = 0 ("Proc  VAL B")
      (unwired) 0 ("Proc  VAL B")
      (unwired) 0 ("Proc  VAL A")
      w74 = i16 0 ("Proc CMD")
      w115 = "\n"  # Line Feed
      w102 = u16 0 items=["None", "XON/XOFF", "RTS/CTS", "XON/XOFF & RTS/CTS", "DTR/DSR", "XON/XOFF & DTR/DSR"] ("Serial Settings:Flow Control")
      w108 = u16 10 items=["1.0"=10, "1.5"=15, "2.0"=20] ("Serial Settings:Stop Bits")
      w109 = u16 0 items=["None", "Odd", "Even", "Mark", "Space"] ("Serial Settings:Parity")
      w132 = T24 0 items=["Clockwise", "Counterclockwise"] ("forward rotation direction")
      w138 = 0.1195  # Robot Radius
      w135 = T25 {"wheel radius"=1.0, "gear ratio"=1.0, "forward rotation direction"=0}  # wheel parameters
      # "一開始要找藍色"
      # "初始化position陣列"
      # "儲存爪子所抓取到的顏色\n\n2    0          1     3\n\\     /           \\     /"
      # "0:x\n1:Green    --> 4:Blue   \n2:Red        --> 1:Green\n3:Yellow   --> 5:Orange\n4:Blue       --> 2:Red\n5:Orange --> 3:Yellow"
      # "1."
      # "1b"
      # "Initialize"
      n5 = for {
        N: 10 -> [_]
        tunnel: [w225] -> w90 mode=indexing
        # "不處理"
        # "下"
        # "上"
        # "方塊顏色初始化"
        n6 = Build Array(i16 0 ("element"), i16 0 ("element"), i16 0 ("element")) -> (w225:i16[])
      }
      "Block Color" <- w90
      n7 = flat-sequence {
        frame #0 {
          w235 = 0.0 ("element")
          w236 = Operator_Loop_Mode."Tele-Op" ("Operator Loop Mode")
          # "初始化變數"
          n8 = local write "Robot Mode:"(w236) -> ()
          n9 = shared-variable ".\\Operator Variables.lvlib\\Mode"(w236) -> ()  [unwired: 1 in, 1 out]
          n10 = Build Array(w235, w235, w235) -> (w234:dbl[])
          n11 = Build Array(0.0 ("element"), 1.15 ("element"), 0.0 ("element")) -> (w232:dbl[])
          n12 = shared-variable ".\\Operator Variables.lvlib\\XY Offset"(i16 0 ("XY Offset")) -> ()  [unwired: 1 in, 1 out]
          n13 = shared-variable ".\\Motor Control Variables.lvlib\\Odometry Data"(w234) -> ()  [unwired: 1 in, 1 out]
          n14 = shared-variable ".\\Motor Control Variables.lvlib\\Heading_Cmd"(0.0 ("Heading_Cmd")) -> ()  [unwired: 1 in, 1 out]
          n15 = shared-variable ".\\Motor Control Variables.lvlib\\VY_Cmd"(0.0 ("VY_Cmd")) -> ()  [unwired: 1 in, 1 out]
          n16 = shared-variable ".\\Motor Control Variables.lvlib\\VX_Cmd"(0.0 ("VX_Cmd")) -> ()  [unwired: 1 in, 1 out]
          n17 = shared-variable ".\\Operator Variables.lvlib\\SubGoal"(w232) -> ()  [unwired: 1 in, 1 out]
          "Block Fix array" <- dbl[] [0.0, 0.0, 0.0] ("Block Fix array")
        }
      }
      n18 = Build Array(i16 0 ("element"), i16 0 ("element"), i16 0 ("element"), i16 0 ("element")) -> (→"Catch Color":i16[])
      n19 = Select(t="URG-30LX Parameters", s="URG-30LX", f="UBG-04FX Parameters") -> (s? t:f=w71:T3)
      n20 = local write "Proc  VAL A"(w74) -> ()
      n21 = local write "Proc  VAL B"(w74) -> ()
      n22 = local write "Proc CMD"(w74) -> ()
      n23 = Unbundle By Name(w71) -> ("Starting Step"=w121:i32, "Ending Step"=w127:i32, "Cluster Count"=w122:i32)
      n24 = Subtract(x=w127, y=w121) -> (x-y=w126:i32)
      n25 = Select(t=0.25 ("x"), s="URG-30LX", f=0.3515625 ("x")) -> (s? t:f=w67:dbl)
      n26 = Increment(x=w126) -> (x+1=w125:i32)
      n27 = xnode "DIR LED"("DIRC (C/DIO5 (DIO5))"=FALSE) -> ()  [unwired: 1 in, 1 out]
      n28 = Divide(x=w125, y=w122) -> (x/y=w124:dbl)
      n29 = Bundle By Name(cluster=w135, "wheel radius"=1.0, "gear ratio"=1.0, "forward rotation direction"=w132) -> (w151:T25)
      n30 = local write "get over"(FALSE ("get over")) -> ()
      n31 = local write "Light"(0.0 ("Light")) -> ()
      n32 = Round To Nearest(number=w124) -> (nearest integer value=w123:dbl)
      "Lidar Array Size" <- w123
      n33 = xnode "PWM LED"("Duty Cycle"=0.0) -> ()  [unwired: 1 in, 1 out]
      n34 = for {
        N: w123 -> [_]
        tunnel: [w246] -> w120 mode=indexing
        tunnel: w122 -> [w243]
        tunnel: w67 -> [w242]
        tunnel: [0] -> w50 mode=indexing
        i -> [w247]
        n35 = Multiply(x=w242, y=w247) -> (x*y=w244:dbl)
        n36 = Multiply(x=w244, y=w243) -> (x*y=w245:dbl)
        n37 = Add(x=w245, y=-120.0) -> (x+y=w246:dbl)
      }
      "Angle" <- w120
      n38 = call "SpeedCtrl_4B.vi"("PID gains"=T6 {"proportional gain (Kc)"=0.0, "integral time (Ti, min)"=0.0, "derivative time (Td, min)"=0.0}, "Target Spd. \nmm/s"=w52, "Speed Now"=w52, "Enable"=FALSE) -> ()  [unwired: 7 in, 1 out]
      n39 = for {
        N: 3 -> [_]
        shift-right: [w251] -> w143
        shift-left: errorcluster {"status"=FALSE, "code"=0, "source"=""} ("error out") -> [w252]
        tunnel: [w250] -> w149 mode=indexing
        tunnel: w151 -> [w249]
        tunnel: [w248] -> w147 mode=indexing
        i -> [w248]
        # "1a"
        n40 = call-poly <vilib>:"Create Wheel.vi"("error in (no error)"=w252, "wheel parameters"=w249) -> ("error out"=w251:errorcluster, "omni wheel out"=w250:refnum<class "NI_Robotics_Omnidirectional Wheel.lvclass">)  [unwired: 8 in]
      }
      n41 = for {
        N: 5 -> [_]
        tunnel: [0.0] -> w62 mode=indexing
      }
      "FYArr" <- w62
      "FXArr" <- w62
      n42 = local write "Enable ND"(FALSE ("Enable ND")) -> ()
      n43 = local write "Block Find"(FALSE ("Block Find")) -> ()
      n44 = Divide(x=6.283185307179586, y=3.0) -> (x/y=w148:dbl)
      n45 = local write "Lidar mid"(0 ("Lidar mid")) -> ()
      n46 = call "URG-04LX-UG01 Initialize.vi"("Acquisition Parameters"=w71, "URG-04LX-UG01 Resource Reference"="URG-04LX Resource") -> ("error out"=w117:errorcluster, "Acquisition Parameters"=w118:T3, "VISA Refnum out"=w119:refnum<visa-resource-name>)  [unwired: 7 in]
      n47 = Multiply(x=w147, y=w148) -> (x*y=w142:dbl[])
      n48 = VISA Open(error in (no error)=errorcluster {"status"=FALSE, "code"=0, "source"=""}, VISA resource name="RC servo resource") -> (VISA resource name=w106:refnum<visa-resource-name>, error out=w105:errorcluster)  [unwired: 3 in]
      n49 = Sine & Cosine(0:w142) -> (1:w141:dbl[], 2:w140:dbl[])
      n50 = local write "Distance"(w50) -> ()
      n51 = String To Byte Array(string=w115) -> (unsigned byte array=w114:u8[])
      n52 = VISA Flush I/O Buffer(VISA resource name=w106, error in (no error)=w105) -> (VISA resource name out=w103:refnum<visa-resource-name>, error out=w104:errorcluster)  [unwired: 1 in]
      n53 = Index Array(array=w114) -> (element=w116:u8)  [unwired: 1 in]
      n54 = Multiply(x=w138, y=w141) -> (x*y=w146:dbl[])
      n55 = Multiply(x=w138, y=w140) -> (x*y=w145:dbl[])
      n56 = Subtract(x=1.5707963267948966, y=w142) -> (x-y=w144:dbl[])
      n57 = call "Z_init.vi"("Resource Reference"="Z Sensor resource") -> ("error out"=w97:errorcluster, "VISA Refnum out"=w98:refnum<visa-resource-name>)  [unwired: 9 in]
      n58 = property class="Instr"(reference=w103, error in=w104, "Baud"=u32 115200 ("Serial Settings:Baud Rate"), "Data Bits"=u16 8 ("Serial Settings:Data Bits"), "Parity"=w109, "Stop Bits"=w108, "Flow Cntrl"=w102, "TermChar"=w116, "TermChar En"=FALSE ("Message Based Settings:Termination Character Enable")) -> (reference out=w100:refnum<visa-resource-name>, error out=w101:errorcluster)
      n59 = call-poly <vilib>:"Create Steering Frame.vi"("wheel frame angles (rad)"=w144, "error in (no error)"=w143, "wheel y positions"=w145, "wheel x positions"=w146, "wheels"=w149) -> ("error out"=w129:errorcluster, "steering frame out"=w130:refnum<class "NI_Robotics_Steering Frame.lvclass">)  [unwired: 5 in]
      n60 = local write "Timer Run"(FALSE ("Timer Run")) -> ()
      "Proc Index" <- i16 0 ("Proc Index")
      "Proc Time" <- i16 0 ("Proc Time")
      "Proc Catch Index" <- i16 0 ("Proc Catch Index")
      "Proc Block Index" <- i16 0 ("Proc Block Index")
      "Proc Finish" <- FALSE ("Proc Finish")
      "Left Block" <- FALSE ("Left Block")
      "Right Block" <- FALSE ("Right Block")
      "Up Color" <- 0 ("Up Color")
      "Down Color" <- 0 ("Down Color")
      "XL Find" <- 0.0 ("XL Find")
      "Y Find" <- 9999.0 ("Y Find")
      "XR Find" <- 9999.0 ("XR Find")
      "XL Dots" <- 0.0 ("XL Find")
      "XR Dots" <- 0.0 ("XR Find")
      "X Find" <- 0.0 ("XL Find")
      "Put Counter" <- w61
      "FYindex" <- w61
      "FXindex" <- w61
      "Proc Down Color" <- 4 ("Proc Down Color")
      "nearwall" <- FALSE ("nearwall")
      "Start POS" <- dbl[] [0.0, 0.0, 0.0] ("Start Front")
      "Start Front" <- dbl[] [0.0, 0.4125, 0.0] ("Start Front")
      "Start Out Point" <- dbl[] [0.0, 0.1725] ("Start Out Point")
      "Block Array" <- dbl[][] [] ("Block Array")
      "OffsetZero" <- 0 ("OffsetZero")
    }
    frame #2 {
      n61 = xnode "LED 2"("LED0"=TRUE) -> ()  [unwired: 1 in, 1 out]
      n62 = xnode "DIR LED 2"("DIRC (C/DIO5 (DIO5))"=FALSE) -> ()  [unwired: 1 in, 1 out]
      n63 = local write "Light"(0.0 ("Light")) -> ()
    }
    frame #3 {
      n64 = xnode "DIR LED 3"("DIRC (C/DIO5 (DIO5))"=FALSE) -> ()  [unwired: 1 in, 1 out]
      n65 = while {
        tunnel: w352 -> [w409]
        tunnel: [w408] -> w351
        tunnel: w350 -> [w407]
        tunnel: [w406] -> w349
        tunnel: [w402] -> _
        stop <- w405 stop-if-true
        n66 = call "Z_Read_Data.vi"("error in"=w409, "VISA Refnum in"=w407) -> ("error out"=w408:errorcluster, "OUT"=w404:dbl, "VISA Refnum out"=w406:refnum<visa-resource-name>)  [unwired: 7 in]
        n67 = Negate(x=w404) -> (-x=w403:dbl)
        n68 = expression code="(x/180.0)*pi" "degrees to radians"(w403) -> (w402:dbl)
        n69 = Not Equal To 0?(x=w402) -> (x != 0?=w405:bool)
      }
      n70 = call "StartCam.vi"("Session In"="Session In") -> ("error out"=w344:errorcluster, "New Image"=w345:T1, "Session Out"=w346:T2)  [unwired: 8 in]
      n71 = xnode "LED 3"("LED1"=TRUE ("LED0")) -> ()  [unwired: 1 in, 1 out]
      n72 = call "URG-04LX-UG01 Start Acquisition.vi"("VISA Refnum in 2"=w358, "Acquisition Parameters"=w357, "error in (no error)"=w356) -> ("VISA Refnum in"=w361:refnum<visa-resource-name>, "Acquisition Parameters"=w359:T3, "error out"=w360:errorcluster)  [unwired: 6 in]
      n73 = call "IMAQ Create"("Image Name"="im1") -> ("New Image"=w339:T1, "error out"=w338:errorcluster)  [unwired: 4 in]
      n74 = call <vilib>:"IMAQdx Grab2.vi"("error in"=w344, "Image In"=w345, "Session In"=w346) -> ("error out"=w343:errorcluster, "Image Out"=w341:T1, "Session Out"=w342:T2)  [unwired: 5 in, 1 out]
      n75 = local write "Image Out"(w341) -> ()
      n76 = VISA Flush I/O Buffer(VISA resource name=w361, error in (no error)=w360) -> (VISA resource name out=w362:refnum<visa-resource-name>)  [unwired: 1 in, 1 out]
      "Z offset" <- 0.0 ("offset value")
    }
    frame #4 {
      w493 = 5
      w496 = T26 {"StartUp Cnt. A"=0.0, "StartUp Cnt. B"=0.0, "StartUp Cnt. C"=0.0}  # StartUp Enc
      # "0:等待執行按鍵\n1:有QR_CODE狀態處裡\n    0:設定出發區前為目標\n    10:執行Go Target\n    20:等待執行完成執行Idle\n    50:跳到(外10)\n2:沒有QR_CODE處裡\n    0:設定出發區前為目標\n    10:執行Go Target\n    20:舉起手臂\n    22:等待執行完成執行Positioning\n    25:以找到的XYZ修正\n          Start POS,Start Front,Start Out\n    27:開啟尋找方塊功能\n    28:關閉尋找方塊功能\n    30:若是沒有看到方塊(內40)\n          等待執行完成執行Idle(內90)\n    40:設定目標到出發區旁邊\n    45:執行走到出發區旁邊\n    50:抵達目標,轉向目標\n    55:待機\n    60:開啟尋找方塊功能\n    65:關閉尋找方塊功能\n    90:跳到(外10)\n3:單獨測試取放方塊用程式\n10:目標處裡\n    0:執行WhereGo找出並設定要走的位置\n    10:利用執行結果設定下一個目標\n    15:設定避障走到目標\n    20:面向目標定位\n    25:對正目標\n    30:A:以目前位置校正XYZ\n          B:若是目標過寬,直接回頭離開\n    35:判斷是否取過方塊\n          A.讀顏色,取方塊(37)\n          B.放方塊(80)\n    37:判斷是否為不用處理方塊\n    40:找出空爪子\n    42:抓取方塊程序開始\n    45:按照爪子索引執行抓取表\n\n    70:跳到放方塊判斷(80)\n    80:找出顏色對應的爪子\n    82:放方塊程序開始\n\n    90:目前目標處裡完成,回到(內0)\n          若是之後沒有方塊目標(內92)\n    92:設定目標反轉\n    94:GoTarget反轉\n    96:目前目標處裡完成,回到(內0)\n          若是之後沒有方塊目標(內98)\n           設定FindBlock\n    98:FindBlock結束(內0)\n    \n\n100:進入出發區處裡\n    0:設定出發區前定位點為目標\n    5:執行避障行走到目標\n    10:設定執行正對目標\n    20:設定執行對正出發區校正\n    30:校正XYZ,並設定出發區內為目標\n    40:執行對正目標\n    45:設為待機模式\n    50:程式歸零"
      # "設定行走目標要小於18cm"
      # "Acquire and process data"
      n77 = node-c288(i64 10 ("Period")) -> (w450:T20)  [unwired: 3 in]
      n78 = timed-loop {
        timing: w450 -> [_]
        timing-out: [_] -> w449
        shift-right: [w501] -> _
        shift-left: FALSE ("y") -> [w506]
        shift-right: [w504] -> _
        shift-left: 0 -> [w505]
        shift-right: [w503] -> _
        shift-left: 0 -> [w502]
        stop <- w508 stop-if-true
        n79 = node-c288() -> ()  [unwired: 1 in, 1 out]
        n80 = shared-variable ".\\Operator Variables.lvlib\\Mode"() -> (w510:T19)  [unwired: 1 in, 1 out]
        n81 = Equal?(x=w510, y=Operator_Loop_Mode."moveblock" ("Operator Loop Mode")) -> (x = y?=w507:bool)
        n82 = case shown="True" w507 {
          tunnel: [FALSE w519] -> w501
          tunnel: w506 -> [_ w518]
          tunnel: w505 -> [_ w517]
          tunnel: [0 w516] -> w504
          tunnel: [0 w514] -> w503
          tunnel: w502 -> [_ w515]
          frame False {
          }
          frame True {
            n83 = xnode "light sensor"() -> ("B/DIO0 (Pin 11)"=w521:bool)  [unwired: 1 in, 1 out]
            n84 = Equal?(x=w521, y=TRUE) -> (x = y?=w520:bool)
            n85 = case shown="True" w520 {
              tunnel: [w526 w547] -> w519
              tunnel: w518 -> [w523 w542]
              tunnel: w517 -> [w528 w549]
              tunnel: [w525 w548] -> w516
              tunnel: w515 -> [w524 w543]
              tunnel: [w527 w544] -> w514
              frame False {
                # "White"
                n86 = Equal?(x=w524, y=0) -> (x = y?=w530:bool)
                n87 = case shown="True" w530 {
                  tunnel: w528 -> [w532 w541]
                  tunnel: [w532 w539] -> w525
                  tunnel: [w531 w534] -> w526
                  tunnel: [w533 w535] -> w527
                  tunnel: w524 -> [w533 _]
                  tunnel: w523 -> [w531 w534]
                  frame False {
                  }
                  frame True {
                    n88 = Increment(x=w541) -> (x+1=w539:i32)
                    n89 = Greater Or Equal?(x=w539, y=2) -> (x >= y?=w538:bool)
                    n90 = Select(t=i16 1, s=w538, f=i16 0) -> (s? t:f=w535:i16)
                  }
                }
              }
              frame True {
                # "Block"
                n91 = Equal?(x=w543, y=1) -> (x = y?=w546:bool)
                n92 = case shown="True" w546 {
                  tunnel: w549 -> [w551 w557]
                  tunnel: [w551 w555] -> w548
                  tunnel: [w550 w554] -> w547
                  tunnel: [w552 w553] -> w544
                  tunnel: w543 -> [w552 w553]
                  tunnel: w542 -> [w550 _]
                  frame False {
                  }
                  frame True {
                    n93 = Increment(x=w557) -> (x+1=w555:i32)
                    n94 = Greater Or Equal?(x=w555, y=2) -> (x >= y?=w554:bool)
                  }
                }
              }
            }
          }
        }
        "B/DIO0 (Pin 11)" <- w501
        n95 = node-c288() -> ()  [unwired: 1 in, 1 out]
        n96 = local read "stop"() -> (w508:bool)
      }
      n97 = node-c288(i64 100 ("Period")) -> (w466:T20)  [unwired: 3 in]
      n98 = timed-loop {
        timing: w466 -> [_]
        timing-out: [_] -> w465
        shift-right: [w606] -> _
        shift-left: dbl[] [0.0, 0.0, 0.0] -> [w612]
        shift-right: [w607] -> _
        shift-left: 0 -> [w602]
        stop <- w614 stop-if-true
        n99 = node-c288() -> ()  [unwired: 1 in, 1 out]
        n100 = call "ultrasonic.vi"("error in (no error)"=errorcluster {"status"=FALSE, "code"=0, "source"=""}, "ADDRESS"=u8 119) -> ("x/y 2"=w601:dbl)  [unwired: 8 in, 1 out]
        n101 = Multiply(x=w601, y=1000.0) -> (x*y=w599:dbl)
        "UltraSound" <- w599
        n102 = Replace Array Subset(array=w612, new element=w599, index=w602) -> (w606:dbl[])
        n103 = Sort 1D Array(array=w606) -> (sorted array=w605:dbl[])
        n104 = Index Array(array=w605, index=1) -> ()  [unwired: 1 out]
        n105 = local read "stop"() -> (w614:bool)
        n106 = Increment(x=w602) -> (x+1=w608:i32)
        n107 = Greater Or Equal?(x=w608, y=3) -> (x >= y?=w610:bool)
        n108 = Select(t=0, s=w610, f=w608) -> (s? t:f=w607:i32)
        n109 = node-c288() -> ()  [unwired: 1 in, 1 out]
      }
      n110 = while {
        shift-right: [w652] -> _
        shift-left: 0.0 -> [w667]
        tunnel: w473 -> [w664]
        tunnel: w472 -> [w663]
        shift-right: [w653] -> _
        shift-left: 0 -> [w655]
        shift-right: [w654] -> _
        shift-left: dbl[] [0.0, 0.0, 0.0] -> [w656]
        stop <- w666 stop-if-true
        n111 = call "Z_Read_Data.vi"("error in"=w664, "IN"=w667, "VISA Refnum in"=w663) -> ("OUT"=w652:dbl)  [unwired: 6 in, 2 out]
        n112 = Negate(x=w652) -> (-x=w651:dbl)
        n113 = Replace Array Subset(array=w656, new element=w651, index=w655) -> (w654:dbl[])
        n114 = Sort 1D Array(array=w654) -> (sorted array=w661:dbl[])
        n115 = Index Array(array=w661, index=1) -> ()  [unwired: 1 out]
        n116 = expression code="(x/180.0)*pi" "degrees to radians"(w651) -> (→"Sensor z":dbl)
        n117 = Increment(x=w655) -> (x+1=w660:i32)
        n118 = Greater Or Equal?(x=w660, y=3) -> (x >= y?=w658:bool)
        n119 = local read "stop"() -> (w666:bool)
        n120 = Select(t=0, s=w658, f=w660) -> (s? t:f=w653:i32)
      }
      n121 = Divide(x=w493, y=i64 1000) -> (x/y=w495:dbl)
      n122 = while {
        shift-right: [w1867] -> _
        shift-left: 0 -> [w1869]
        i -> [w1875]
        stop <- w1877 stop-if-true
        # "光答資料要有更新才會閃爍"
        # "第二顆LED閃爍"
        n123 = local read "Lidar mid"() -> (w1866:i32)
        n124 = Wait (ms)(milliseconds to wait=u32 300) -> ()  [unwired: 1 out]
        n125 = Quotient & Remainder(x=w1875, y=2) -> (x-y*floor(x/y)=w1873:i32)  [unwired: 1 out]
        n126 = Not Equal?(x=w1866, y=w1869) -> (x != y?=w1868:bool)
        n127 = Equal?(x=w1873, y=1) -> (x = y?=w1871:bool)
        n128 = Select(t=w1866, s=w1868, f=w1869) -> (s? t:f=w1867:i32)
        n129 = And(x=w1868, y=w1871) -> (x .and. y?=w1870:bool)
        n130 = xnode "LED"("LED1"=w1870) -> ()  [unwired: 1 in, 1 out]
        n131 = local read "stop"() -> (w1877:bool)
      }
      n132 = node-c288(w493) -> (w500:T20)  [unwired: 3 in]
      n133 = timed-loop {
        timing: w500 -> [_]
        timing-out: [_] -> w499
        tunnel: w498 -> [w2621]
        shift-right: [w2603] -> _
        shift-left: w496 -> [w2576]
        tunnel: w495 -> [w2565]
        tunnel: w494 -> [w2610]
        tunnel: w479 -> [w2609]
        tunnel: [w2597] -> _
        tunnel: [w2596] -> w492
        stop <- w2606 stop-if-true
        w2585 = 1000.0 ("y")
        w2589 = 1000.0 ("y")
        # "速度控制"
        # "編碼器讀取"
        # "世界座標計算"
        # "馬達行走與座標運算"
        n134 = node-c288() -> ()  [unwired: 1 in, 1 out]
        n135 = shared-variable ".\\Motor Control Variables.lvlib\\Odometry Data"() -> (w2595:dbl[])  [unwired: 1 in, 1 out]
        n136 = shared-variable ".\\Motor Control Variables.lvlib\\Heading_Cmd"() -> (w2561:dbl)  [unwired: 1 in, 1 out]
        n137 = shared-variable ".\\Motor Control Variables.lvlib\\VX_Cmd"() -> (w2566:dbl)  [unwired: 1 in, 1 out]
        "X Velocity Feedback" <- w2566
        n138 = shared-variable ".\\Motor Control Variables.lvlib\\VY_Cmd"() -> (w2570:dbl)  [unwired: 1 in, 1 out]
        n139 = Index Array(array=w2595) -> (element #1=w2590:dbl, element #2=w2588:dbl, element #3=w2577:dbl)  [unwired: 3 in]
        n140 = expression code="(x/pi)*180.0" "radians to degrees"(w2577) -> (w2594:dbl)
        n141 = Negate(x=w2570) -> (-x=w2598:dbl)
        "Y Velocity Feedback" <- w2598
        n142 = Multiply(x=w2590, y=w2589) -> (x*y=w2587:dbl)
        n143 = Multiply(x=w2589, y=w2588) -> (x*y=w2586:dbl)
        n144 = call "EnCoder.vi"("Reset Counter"="Reset Counter", "Encoder PPR"="Encoder PPR", "Gear Ratio"="Gear Ratio", "R(mm)"="R(mm)", "error in"=w2621) -> ("ENC Val. mm"=w2603:T7, "error out"=w2608:errorcluster)  [unwired: 4 in, 1 out]
        "ENC Val. mm" <- w2603
        n145 = Bundle(w2587, w2586, "Numeric"=w2594) -> (w2593:cluster{dbl, dbl, "Numeric":dbl})  [unwired: 1 in]
        n146 = Subtract(x=w2603, y=w2576) -> (x-y=w2602:cluster{dbl, dbl, dbl})
        n147 = call "Odometry.vi"("L"=119.5, "POS in"=w2593, "ENC Diff(mm)"=w2602) -> ("POS out"=w2592:cluster{"X":dbl, "Y":dbl, "Angle":dbl})  [unwired: 8 in]
        "Now POS" <- w2592
        n148 = Divide(x=w2602, y=w2565) -> (x/y=w2620:cluster{dbl, dbl, dbl})
        n149 = Unbundle(w2592) -> ("X"=w2584:dbl, "Y"=w2583:dbl, "Angle"=w2591:dbl)
        n150 = expression code="(x/180.0)*pi" "degrees to radians"(w2591) -> (w2580:dbl)
        n151 = Divide(x=w2584, y=w2585) -> (x/y=w2581:dbl)
        n152 = Divide(x=w2583, y=w2585) -> (x/y=w2582:dbl)
        n153 = local read "Block Fix array"() -> (w2568:dbl[])
        n154 = Index Array(array=w2568) -> (element=w2569:dbl)  [unwired: 1 in]
        n155 = Not Equal To 0?(x=w2569) -> (x != 0?=w2567:bool)
        n156 = Build Array(w2581, w2582, w2580) -> (w2579:dbl[])
        n157 = case shown="True" w2567 {
          tunnel: w2579 -> [w2668 w2675]
          tunnel: [w2668 w2670] -> w2575
          tunnel: w2568 -> [_ w2676]
          tunnel: w2561 -> [w2667 _]
          tunnel: [w2667 w2669] -> w2560
          frame False {
          }
          frame True {
            n158 = Index Array(array=w2676) -> (element #1=w2672:dbl, element #2=w2671:dbl, element #3=w2674:dbl)  [unwired: 3 in]
            n159 = Index Array(array=w2675) -> (element #3=w2673:dbl)  [unwired: 3 in, 2 out]
            n160 = call "GLOBAL Z.vi"("wZ"=w2673, "sZ"=w2674) -> ("TZ"=w2669:dbl)  [unwired: 9 in]
            n161 = Build Array(w2672, w2671, w2669) -> (w2670:dbl[])
            n162 = shared-variable ".\\Motor Control Variables.lvlib\\Heading_Cmd"(w2669) -> ()  [unwired: 1 in, 1 out]
            n163 = local write "Block Fix array"(dbl[] [0.0, 0.0, 0.0] ("Block Fix array")) -> ()
          }
        }
        n164 = local read "Z offset"() -> (w2564:dbl)
        n165 = Not Equal To 0?(x=w2564) -> (x != 0?=w2557:bool)
        n166 = shared-variable ".\\Operator Variables.lvlib\\SubGoal"() -> (→"SubGoal":dbl[])  [unwired: 1 in, 1 out]
        n167 = Index Array(array=w2575) -> (element #1=w2574:dbl, element #2=w2573:dbl, element #3=w2563:dbl)  [unwired: 3 in]
        n168 = case shown="False" w2557 {
          tunnel: w2564 -> [_ w2665]
          tunnel: [w2661 w2663] -> w2562
          tunnel: w2563 -> [w2661 w2662]
          frame False {
          }
          frame True {
            n169 = local read "Sensor z"() -> (w2666:dbl)
            n170 = Add(x=w2665, y=w2666) -> (x+y=w2664:dbl)
            n171 = call "GLOBAL Z.vi"("wZ"=w2662, "sZ"=w2664) -> ("TZ"=w2663:dbl)  [unwired: 9 in]
          }
        }
        n172 = local read "Light"() -> (w2558:dbl)
        n173 = Build Array(w2574, w2573, w2562) -> (w2572:dbl[])
        "Odometry Data" <- w2572
        n174 = Index Array(array=w2572) -> (element #3=w2578:dbl)  [unwired: 3 in, 2 out]
        n175 = call-poly <vilib>:"PID.vi"("output range"=cluster{"output high":dbl, "output low":dbl} {"output high"=2.5, "output low"=-2.5}, "dt (s)"=w2565, "PID gains"=T6 {"proportional gain (Kc)"=3.3, "integral time (Ti, min)"=0.0, "derivative time (Td, min)"=0.0}, "process variable"=w2578, "setpoint"=w2560) -> ("output"=w2571:dbl)  [unwired: 5 in, 1 out]
        "Angular Velocity Feedback" <- w2571
        n176 = Build Array(w2566, w2598, w2571) -> (w2612:dbl[])
        n177 = call-poly <vilib>:"Apply Velocity to Motors.vi"("error in (no error)"=w2609, "steering frame velocity"=w2612, "steering frame in"=w2610) -> ("error out"=w2607:errorcluster, "ccw motor velocity setpoints"=w2611:dbl[], "steering frame out"=w2597:refnum<class "NI_Robotics_Steering Frame.lvclass">)  [unwired: 4 in, 2 out]
        n178 = Index Array(array=w2611) -> (element #1=w2604:dbl, element #2=w2605:dbl, element #3=w2618:dbl)  [unwired: 3 in]
        n179 = Bundle("Numeric"=w2604, "Numeric"=w2605, "Numeric"=w2618) -> (w2615:T27)  [unwired: 1 in]
        n180 = Multiply(x=w2615, y=1000.0) -> (x*y=w2614:T27)
        n181 = Merge Errors(w2608, w2607) -> (w2596:errorcluster)
        n182 = call "SpeedCtrl_4B.vi"("dt (s)"=w2565, "PID gains"="PID gains", "Target Spd. \nmm/s"=w2614, "Speed Now"=w2620, "Enable"="Enable") -> ()  [unwired: 6 in, 1 out]
        n183 = Or(x=w2596, y="stop") -> (x .or. y?=w2606:bool)
        n184 = shared-variable ".\\Motor Control Variables.lvlib\\Odometry Data"(w2572) -> ()  [unwired: 1 in, 1 out]
        n185 = xnode "PWM LED 2"("Duty Cycle"=w2558) -> ()  [unwired: 1 in, 1 out]
        n186 = node-c288() -> ()  [unwired: 1 in, 1 out]
      }
      n187 = shared-variable ".\\Operator Variables.lvlib\\Mode"() -> (w488:T19)  [unwired: 1 in, 1 out]
      n188 = call "Compute Obstacle Clearance.vi"() -> ()  [unwired: 1 in, 1 out]
      n189 = node-c288(w449) -> ()  [unwired: 1 out]
      n190 = node-c288(w465) -> ()  [unwired: 1 out]
      n191 = node-c288(i64 100 ("Period")) -> (w478:T20)  [unwired: 3 in]
      n192 = node-c288(i64 100 ("Period")) -> (w486:T20)  [unwired: 3 in]
      n193 = timed-loop "Timed Loop" {
        timing: w478 -> [_]
        timing-out: [_] -> w477
        shift-right: [w680] -> _
        shift-left: 0 ("f") -> [w674]
        shift-right: [w675] -> _
        shift-left: 0 ("f") -> [w671]
        shift-right: [w677] -> _
        shift-left: 0 ("f") -> [w670]
        tunnel: w463 -> [w672]
        tunnel: w454 -> [w669]
        tunnel: w453 -> [w668]
        stop <- w673 stop-if-true
        # "內圈"
        # "外圈"
        # "最大計數50秒"
        # "程式處理區"
        n194 = node-c288() -> ()  [unwired: 1 in, 1 out]
        n195 = case shown="10" w671 {
          tunnel: w671 -> [w701 w790 w931 w1154 w1245 w1710]
          tunnel: w670 -> [w702 w791 w932 w1155 w1246 w1711]
          tunnel: [w702 w788 w929 w1152 w1243 w1708] -> w676
          tunnel: [w700 w789 w930 w1153 w1244 w1709] -> w675
          tunnel: w674 -> [w696 w787 w928 w1151 w1241 w1707]
          tunnel: w672 -> [_ w786 w927 w1150 w1242 _]
          tunnel: w669 -> [w692 _ _ _ _ _]
          tunnel: w668 -> [w691 _ _ _ _ _]
          frame 0, Default {
            n196 = xnode "Button"() -> ("Value"=w694:bool)  [unwired: 1 in, 1 out]
            n197 = Greater?(x=w696, y=5) -> (0:w698:bool)
            n198 = local read "Lidar mid"() -> (w689:i32)
            n199 = Or(x=w694, y="PLAY") -> (x .or. y?=w693:bool)
            n200 = Not Equal?(x=0, y=w689) -> (x != y?=w690:bool)
            n201 = Compound Arithmetic op=AND(w693, w698, w690) -> (w697:bool)
            n202 = case shown="False" w697 {
              tunnel: w701 -> [w745 _]
              tunnel: [w747 w783] -> w700
              tunnel: w692 -> [w744 _]
              tunnel: w691 -> [w743 _]
              frame False {
                n203 = case shown="True" "Set Z Offset" {
                  frame False {
                  }
                  frame True {
                    n204 = shared-variable ".\\Motor Control Variables.lvlib\\Odometry Data"() -> (w775:dbl[])  [unwired: 1 in, 1 out]
                    n205 = local read "Sensor z"() -> (w772:dbl)
                    n206 = Index Array(array=w775, index=2) -> (element=w773:dbl)
                    n207 = Subtract(x=w773, y=w772) -> (x-y=w771:dbl)
                    n208 = local write "Z offset"(w771) -> ()
                  }
                }
                n209 = case shown="True" "Set Test SubGoal" {
                  frame False {
                  }
                  frame True {
                    n210 = shared-variable ".\\Motor Control Variables.lvlib\\Odometry Data"() -> (w767:dbl[])  [unwired: 1 in, 1 out]
                    n211 = Index Array(array=w767) -> (element #1=w766:dbl, element #2=w765:dbl, element #3=w762:dbl)  [unwired: 3 in]
                    n212 = Add(x=w765, y=1.0) -> (x+y=w763:dbl)
                    n213 = Add(x=w762, y=0.0) -> (x+y=w760:dbl)
                    n214 = Build Array(w766, w763, w760) -> (w759:dbl[])
                    n215 = shared-variable ".\\Operator Variables.lvlib\\SubGoal"(w759) -> ()  [unwired: 1 in, 1 out]
                  }
                }
                n216 = case shown="True" "Run Catch" {
                  tunnel: w745 -> [w768 _]
                  tunnel: [w768 3] -> w747
                  frame False {
                  }
                  frame True {
                    n217 = local write "Proc Catch Index"("Test Catch") -> ()
                  }
                }
                n218 = local read "Light Set"() -> (w739:dbl)
                n219 = local read "Robot Mode:"() -> (w750:T5)
                n220 = case shown="True" "Load Image" {
                  tunnel: w744 -> [_ w753]
                  tunnel: w743 -> [_ w752]
                  frame False {
                  }
                  frame True {
                    n221 = Concatenate Strings("/c/" ("string"), "Select Image", ".png" ("string")) -> (w756:string)
                    n222 = String To Path(string=w756) -> (path=w755:path)
                    n223 = call "IMAQ ReadFile 2"("File Path"=w755, "error in (no error)"=w752, "Image"=w753) -> ("Image Out"=w751:T1)  [unwired: 4 in, 4 out]
                    n224 = local write "Image Out"(w751) -> ()
                  }
                }
                n225 = Select(t=w739, s="Light ON", f=0.0) -> (s? t:f=w741:dbl)
                n226 = local write "Light"(w741) -> ()
                n227 = shared-variable ".\\Operator Variables.lvlib\\Mode"(w750) -> ()  [unwired: 1 in, 1 out]
              }
              frame True {
                w778 = u64 0 ("MIN")
                # "無QR CODE是直接走出來,做定位"
                # "有QR CODE是面對內倒車出來"
                n228 = local read "QR_CAM"() -> (w781:bool)
                n229 = local write "Block Find"(FALSE ("Block Find")) -> ()
                n230 = local write "Timer Run"(TRUE ("Timer Run")) -> ()
                n231 = Select(t=1, s=w781, f=2) -> (s? t:f=w783:i32)
                n232 = local write "Light"(0.0 ("Light")) -> ()
                n233 = local write "get over"(FALSE ("get over")) -> ()
                n234 = local write "PLAY"(FALSE ("PLAY")) -> ()
                n235 = local write "Put Counter"(w778) -> ()
                n236 = local write "SEC"(w778) -> ()
                n237 = local write "MIN"(w778) -> ()
              }
            }
          }
          frame 1 {
            # "ず"
            # "外"
            # "外"
            # "有QR CODE的狀態,由出發區走出來"
            n238 = case shown="2" w791 {
              tunnel: w791 -> [_ w808 w827 w845 w870 w894 w904 w916]
              tunnel: w790 -> [w795 w811 w834 w846 w872 w893 w906 w913]
              tunnel: [w795 w811 w834 w846 w871 w893 w907 w914] -> w789
              tunnel: [2 ("f") w800 w828 w844 w873 w895 w905 w915] -> w788
              tunnel: w787 -> [_ w809 w830 w840 w866 w889 w900 w918]
              tunnel: w786 -> [_ _ _ w838 _ _ _ _]
              frame 0, Default {
                w794 = Operator_Loop_Mode."readQR" ("Operator Loop Mode")
                n239 = local write "Start POS"(dbl[] [0.0, 0.0, 0.0] ("Start POS")) -> ()
                n240 = local write "Robot Mode:"(w794) -> ()
                n241 = shared-variable ".\\Operator Variables.lvlib\\Mode"(w794) -> ()  [unwired: 1 in, 1 out]
              }
              frame 2 {
                n242 = local read "Start POS"() -> (w807:dbl[])
                n243 = local read "Start Front"() -> (w799:dbl[])
                n244 = local read "Proc Finish"() -> (w804:bool)
                n245 = Index Array(array=w807, index=0) -> (element=w805:dbl)
                n246 = Index Array(array=w799, index=0) -> (element=w797:dbl)
                n247 = Greater?(x=w809, y=5.0) -> (0:w803:bool)
                n248 = Not Equal To 0?(x=w805) -> (x != 0?=w802:bool)
                n249 = Not Equal To 0?(x=w797) -> (x != 0?=w796:bool)
                n250 = Compound Arithmetic op=AND(w796, w804, w803, w802) -> (w801:bool)
                n251 = case shown="True" w801 {
                  tunnel: [w812 30] -> w800
                  tunnel: w808 -> [w812 _]
                  frame False {
                  }
                  frame True {
                    # "設定目標出口位置"
                    n252 = local read "Start POS"() -> (w816:dbl[])
                    n253 = local read "Start Front"() -> (w822:dbl[])
                    n254 = Index Array(array=w822) -> (element #1=w825:dbl, element #2=w824:dbl)  [unwired: 2 in]
                    n255 = Index Array(array=w816, index=2) -> (element=w814:dbl)
                    n256 = local read "Sensor z"() -> (w819:dbl)
                    n257 = Index Array(array=w816, index=2) -> (element=w817:dbl)
                    n258 = Add(x=w814, y=3.141592653589793) -> (x+y=w813:dbl)
                    n259 = Build Array(w825, w824, w813) -> (w823:dbl[])
                    n260 = local write "Block Fix array"(w816) -> ()
                    n261 = shared-variable ".\\Operator Variables.lvlib\\SubGoal"(w823) -> ()  [unwired: 1 in, 1 out]
                    n262 = Subtract(x=w817, y=w819) -> (x-y=w818:dbl)
                    n263 = local write "Z offset"(w818) -> ()
                  }
                }
              }
              frame 10 {
                n264 = local read "Proc Finish"() -> (w833:bool)
                n265 = Greater?(x=w830, y=3) -> (0:w832:bool)
                n266 = And(x=w833, y=w832) -> (x .and. y?=w831:bool)
                n267 = case shown="True" w831 {
                  tunnel: [w835 30] -> w828
                  tunnel: w827 -> [w835 _]
                  frame False {
                  }
                  frame True {
                    w837 = Operator_Loop_Mode."Go Target" ("Operator Loop Mode")
                    n268 = local write "Robot Mode:"(w837) -> ()
                    n269 = shared-variable ".\\Operator Variables.lvlib\\Mode"(w837) -> ()  [unwired: 1 in, 1 out]
                  }
                }
              }
              frame 20 {
                n270 = local read "Proc Finish"() -> (w843:bool)
                n271 = Greater?(x=w840, y=20.0) -> (0:w839:bool)
                n272 = And(x=w843, y=w839) -> (x .and. y?=w842:bool)
                n273 = case shown="True" w842 {
                  tunnel: w845 -> [w847 _]
                  tunnel: [w847 30] -> w844
                  tunnel: w838 -> [_ w848]
                  frame False {
                  }
                  frame True {
                    w854 = 1.0 ("ID")
                    w853 = 0.0 ("ID")
                    w863 = Operator_Loop_Mode."Idle" ("Operator Loop Mode")
                    n274 = call "RC_MoveTable.vi"("Index"=w854, "ID"=w853, "CMD"=3.0) -> ("Value"=w856:i32, "RC ID"=w855:i32)  [unwired: 6 in]
                    n275 = call "RC_MoveTable.vi"("Index"=w854, "ID"=w854, "CMD"=3.0) -> ("Value"=w858:i32, "RC ID"=w857:i32)  [unwired: 6 in]
                    n276 = call "RC_MoveTable.vi"("Index"=w854, "ID"=w853, "CMD"=2.0) -> ("Value"=w860:i32, "RC ID"=w859:i32)  [unwired: 6 in]
                    n277 = call "RC_MoveTable.vi"("Index"=w854, "ID"=w854, "CMD"=2.0) -> ("Value"=w862:i32, "RC ID"=w861:i32)  [unwired: 6 in]
                    n278 = call "RCservo.vi"("Value"=w856, "ID"=w855, "VISA resource name"=w848) -> ()  [unwired: 7 in, 2 out]
                    n279 = call "RCservo.vi"("Value"=w858, "ID"=w857, "VISA resource name"=w848) -> ()  [unwired: 7 in, 2 out]
                    n280 = call "RCservo.vi"("Value"=w860, "ID"=w859, "VISA resource name"=w848) -> ()  [unwired: 7 in, 2 out]
                    n281 = call "RCservo.vi"("Value"=w862, "ID"=w861, "VISA resource name"=w848) -> ()  [unwired: 7 in, 2 out]
                    n282 = local write "Robot Mode:"(w863) -> ()
                    n283 = shared-variable ".\\Operator Variables.lvlib\\Mode"(w863) -> ()  [unwired: 1 in, 1 out]
                  }
                }
              }
              frame 30 {
                n284 = local read "Proc Finish"() -> (w869:bool)
                n285 = Greater?(x=w866, y=10.0) -> (0:w867:bool)
                n286 = And(x=w869, y=w867) -> (x .and. y?=w865:bool)
                n287 = case shown="True" w865 {
                  tunnel: [w875 50] -> w873
                  tunnel: w872 -> [w874 w880]
                  tunnel: [w874 w880] -> w871
                  tunnel: w870 -> [w875 _]
                  frame False {
                  }
                  frame True {
                    w882 = Operator_Loop_Mode."Idle" ("Operator Loop Mode")
                    n288 = shared-variable ".\\Motor Control Variables.lvlib\\Odometry Data"() -> (w887:dbl[])  [unwired: 1 in, 1 out]
                    n289 = local read "Block Array"() -> (w877:dbl[][])
                    n290 = local read "Start POS"() -> (w879:dbl[])
                    n291 = call "StartHeading.vi"("Block Array"=w877, "Start POS"=w879) -> ("Heading rad back"=w878:dbl, "block array out"=w876:dbl[][])  [unwired: 8 in]
                    n292 = Index Array(array=w887) -> (element #1=w886:dbl, element #2=w885:dbl, element #3=w884:dbl)  [unwired: 3 in]
                    n293 = local write "Block Array"(w876) -> ()
                    n294 = Add(x=w884, y=w878) -> (x+y=w883:dbl)
                    n295 = Build Array(w886, w885, w883) -> ()  [unwired: 1 out]
                    n296 = local write "Robot Mode:"(w882) -> ()
                    n297 = shared-variable ".\\Operator Variables.lvlib\\Mode"(w882) -> ()  [unwired: 1 in, 1 out]
                  }
                }
              }
              frame 50 {
                n298 = local read "Proc Finish"() -> (w892:bool)
                n299 = Greater?(x=w889, y=5.0) -> (0:w890:bool)
                n300 = And(x=w892, y=w890) -> (x .and. y?=w888:bool)
                n301 = case shown="True" w888 {
                  tunnel: w894 -> [w896 _]
                  tunnel: [w896 60 ("f")] -> w895
                  frame False {
                  }
                  frame True {
                    w898 = Operator_Loop_Mode."Go Target" ("Operator Loop Mode")
                    n302 = local write "Robot Mode:"(w898) -> ()
                    n303 = shared-variable ".\\Operator Variables.lvlib\\Mode"(w898) -> ()  [unwired: 1 in, 1 out]
                  }
                }
              }
              frame 60 {
                n304 = local read "Proc Finish"() -> (w903:bool)
                n305 = Greater?(x=w900, y=2.0) -> (0:w901:bool)
                n306 = And(x=w903, y=w901) -> (x .and. y?=w899:bool)
                n307 = case shown="True" w899 {
                  tunnel: [w909 w910] -> w907
                  tunnel: w906 -> [w909 w910]
                  tunnel: [w908 61] -> w905
                  tunnel: w904 -> [w908 _]
                  frame False {
                  }
                  frame True {
                    w912 = Operator_Loop_Mode."Idle" ("Operator Loop Mode")
                    n308 = local write "Robot Mode:"(w912) -> ()
                    n309 = shared-variable ".\\Operator Variables.lvlib\\Mode"(w912) -> ()  [unwired: 1 in, 1 out]
                  }
                }
              }
              frame 61 {
                n310 = local read "Proc Finish"() -> (w921:bool)
                n311 = Greater?(x=w918, y=2.0) -> (0:w919:bool)
                n312 = And(x=w921, y=w919) -> (x .and. y?=w917:bool)
                n313 = case shown="True" w917 {
                  tunnel: w916 -> [w923 _]
                  tunnel: [w923 0] -> w915
                  tunnel: [w922 10] -> w914
                  tunnel: w913 -> [w922 _]
                  frame False {
                  }
                  frame True {
                    w926 = Operator_Loop_Mode."Idle" ("Operator Loop Mode")
                    n314 = local write "Robot Mode:"(w926) -> ()
                    n315 = shared-variable ".\\Operator Variables.lvlib\\Mode"(w926) -> ()  [unwired: 1 in, 1 out]
                  }
                }
              }
            }
          }
          frame 2 {
            # "ず"
            # "外"
            # "ず"
            # "外"
            # "沒有QR CODE的狀態,由出發區走出來,\n並做定位動作"
            n316 = case shown="0, Default" w932 {
              tunnel: w932 -> [_ _ w954 w980 w985 w1033 w1044 w1061 _ w1099 w1110 w1121 w1132 w1143 w1149]
              tunnel: w931 -> [w943 w946 w955 w981 w992 w1040 w1051 w1062 w1092 w1100 w1111 w1122 w1133 w1144 _]
              tunnel: [w943 w946 w955 w981 w992 w1040 w1051 w1062 w1092 w1100 w1111 w1122 w1133 w1144 10] -> w930
              tunnel: [10 22 w953 w979 w991 w1039 w1050 w1060 45 w1098 w1109 w1120 w1131 w1142 w1149] -> w929
              tunnel: w928 -> [_ _ w948 w974 w986 w1034 w1045 w1059 _ w1097 w1108 w1119 w1130 w1141 _]
              tunnel: w927 -> [_ _ w947 _ _ _ _ _ _ _ _ _ _ _ _]
              frame 0, Default {
                w934 = 9999.0 ("XR Find")
                # "設定目標出口位置"
                n317 = local read "Start Front"() -> (w935:dbl[])
                n318 = local read "Start POS"() -> (w941:dbl[])
                n319 = Index Array(array=w935) -> (element #1=w939:dbl, element #2=w938:dbl)  [unwired: 2 in]
                n320 = Index Array(array=w941, index=2) -> (element=w937:dbl)
                n321 = Build Array(w939, w938, w937) -> (w936:dbl[])
                n322 = local write "XR Find"(w934) -> ()
                n323 = local write "XL Find"(0.0 ("XL Find")) -> ()
                n324 = local write "Y Find"(w934) -> ()
                n325 = shared-variable ".\\Operator Variables.lvlib\\SubGoal"(w936) -> ()  [unwired: 1 in, 1 out]
              }
              frame 10 {
                w944 = Operator_Loop_Mode."Go Target" ("Operator Loop Mode")
                n326 = local write "Robot Mode:"(w944) -> ()
                n327 = shared-variable ".\\Operator Variables.lvlib\\Mode"(w944) -> ()  [unwired: 1 in, 1 out]
              }
              frame 20 {
                n328 = local read "Proc Finish"() -> (w952:bool)
                n329 = Greater?(x=w948, y=10.0) -> (0:w949:bool)
                n330 = And(x=w952, y=w949) -> (x .and. y?=w951:bool)
                n331 = case shown="True" w951 {
                  tunnel: w954 -> [w956 _]
                  tunnel: [w956 22] -> w953
                  tunnel: w947 -> [_ w957]
                  frame False {
                  }
                  frame True {
                    w971 = 1.0 ("ID")
                    w970 = 0.0 ("ID")
                    w972 = Operator_Loop_Mode."Idle" ("Operator Loop Mode")
                    # "手臂舉起"
                    n332 = call "RC_MoveTable.vi"("Index"=w971, "ID"=w970, "CMD"=3.0) -> ("Value"=w964:i32, "RC ID"=w965:i32)  [unwired: 6 in]
                    n333 = call "RC_MoveTable.vi"("Index"=w971, "ID"=w971, "CMD"=3.0) -> ("Value"=w962:i32, "RC ID"=w963:i32)  [unwired: 6 in]
                    n334 = call "RC_MoveTable.vi"("Index"=w971, "ID"=w970, "CMD"=2.0) -> ("Value"=w960:i32, "RC ID"=w961:i32)  [unwired: 6 in]
                    n335 = call "RC_MoveTable.vi"("Index"=w971, "ID"=w971, "CMD"=2.0) -> ("Value"=w958:i32, "RC ID"=w959:i32)  [unwired: 6 in]
                    n336 = call "RCservo.vi"("Value"=w964, "ID"=w965, "VISA resource name"=w957) -> ()  [unwired: 7 in, 2 out]
                    n337 = call "RCservo.vi"("Value"=w962, "ID"=w963, "VISA resource name"=w957) -> ()  [unwired: 7 in, 2 out]
                    n338 = call "RCservo.vi"("Value"=w960, "ID"=w961, "VISA resource name"=w957) -> ()  [unwired: 7 in, 2 out]
                    n339 = call "RCservo.vi"("Value"=w958, "ID"=w959, "VISA resource name"=w957) -> ()  [unwired: 7 in, 2 out]
                    n340 = local write "Robot Mode:"(w972) -> ()
                    n341 = shared-variable ".\\Operator Variables.lvlib\\Mode"(w972) -> ()  [unwired: 1 in, 1 out]
                  }
                }
              }
              frame 22 {
                n342 = local read "Proc Finish"() -> (w978:bool)
                n343 = Greater?(x=w974, y=15.0) -> (0:w975:bool)
                n344 = And(x=w978, y=w975) -> (x .and. y?=w977:bool)
                n345 = case shown="True" w977 {
                  tunnel: w980 -> [w982 _]
                  tunnel: [w982 25] -> w979
                  frame False {
                  }
                  frame True {
                    w983 = Operator_Loop_Mode."Positioning" ("Operator Loop Mode")
                    # "定位動作"
                    n346 = local write "Robot Mode:"(w983) -> ()
                    n347 = shared-variable ".\\Operator Variables.lvlib\\Mode"(w983) -> ()  [unwired: 1 in, 1 out]
                  }
                }
              }
              frame 25 {
                n348 = local read "Proc Finish"() -> (w990:bool)
                n349 = Greater?(x=w986, y=30.0) -> (0:w987:bool)
                n350 = And(x=w990, y=w987) -> (x .and. y?=w989:bool)
                n351 = case shown="True" w989 {
                  tunnel: [w993 27] -> w991
                  tunnel: w985 -> [w993 _]
                  frame False {
                  }
                  frame True {
                    w1003 = Operator_Loop_Mode."Idle" ("Operator Loop Mode")
                    w1006 = 1000
                    # "計算出發區的X,Y"
                    # "進出發區的角度剛好是相反的"
                    n352 = local write "Robot Mode:"(w1003) -> ()
                    n353 = shared-variable ".\\Operator Variables.lvlib\\Mode"(w1003) -> ()  [unwired: 1 in, 1 out]
                    n354 = local read "Angle Find"() -> (w995:dbl)
                    n355 = local read "FY"() -> (w1004:dbl)
                    n356 = local read "FX"() -> (w1005:dbl)
                    n357 = local read "Start Front"() -> (w1016:dbl[])
                    n358 = local read "Start Out Point"() -> (w1012:dbl[])
                    n359 = local read "Sensor z"() -> (w999:dbl)
                    n360 = Add(x=w995, y=3.141592653589793) -> (x+y=w1019:dbl)
                    n361 = Negate(x=w995) -> (-x=w994:dbl)
                    n362 = Quotient & Remainder(x=w1019, y=6.283185307179586) -> (x-y*floor(x/y)=w1020:dbl)  [unwired: 1 out]
                    n363 = Negate(x=w995) -> (-x=w996:dbl)
                    n364 = Subtract(x=w995, y=w999) -> (x-y=w998:dbl)
                    n365 = Index Array(array=w1016) -> (element #1=w1031:dbl, element #2=w1030:dbl)  [unwired: 2 in]
                    n366 = Greater Or Equal?(x=w1020, y=3.141592653589793) -> (x >= y?=w1022:bool)
                    n367 = Index Array(array=w1012) -> (element #1=w1013:dbl, element #2=w1014:dbl)  [unwired: 2 in]
                    n368 = local write "Z offset"(w998) -> ()
                    n369 = Divide(x=w1005, y=w1006) -> (x/y=w1001:dbl)
                    n370 = Divide(x=w1004, y=w1006) -> (x/y=w1000:dbl)
                    n371 = Subtract(x=w1020, y=6.283185307179586) -> (x-y=w1024:dbl)
                    n372 = call-poly <vilib>:"2D Cartesian Coordinate Rotation.vi"("theta"=w994, "y"=w1030, "x"=w1031) -> ("y out"=w1028:dbl, "x out"=w1029:dbl)  [unwired: 6 in, 1 out]
                    n373 = call-poly <vilib>:"2D Cartesian Coordinate Rotation.vi"("theta"=w996, "y"=w1014, "x"=w1013) -> ("y out"=w1010:dbl, "x out"=w1011:dbl)  [unwired: 6 in, 1 out]
                    n374 = Select(t=w1024, s=w1022, f=w1020) -> (s? t:f=w997:dbl)
                    n375 = Subtract(x=w1000, y=w1028) -> (x-y=w1026:dbl)
                    n376 = Subtract(x=w1001, y=w1029) -> (x-y=w1027:dbl)
                    n377 = Subtract(x=w1000, y=w1010) -> (x-y=w1008:dbl)
                    n378 = Subtract(x=w1001, y=w1011) -> (x-y=w1009:dbl)
                    n379 = Build Array(w1001, w1000, w995) -> (w1002:dbl[])
                    n380 = Build Array(w1001, w1000, w995) -> (w1015:dbl[])
                    n381 = Build Array(w1009, w1008) -> (w1007:dbl[])
                    n382 = Build Array(w1027, w1026, w997) -> (w1017:dbl[])
                    n383 = local write "Block Fix array"(w1002) -> ()
                    n384 = local write "Start Out Point"(w1007) -> ()
                    n385 = local write "Start Front"(w1015) -> ()
                    n386 = local write "Start POS"(w1017) -> ()
                  }
                }
              }
              frame 27 {
                n387 = local read "Proc Finish"() -> (w1038:bool)
                n388 = Greater?(x=w1034, y=5.0) -> (0:w1035:bool)
                n389 = And(x=w1038, y=w1035) -> (x .and. y?=w1037:bool)
                n390 = case shown="True" w1037 {
                  tunnel: [w1041 28 ("f")] -> w1039
                  tunnel: w1033 -> [w1041 _]
                  frame False {
                  }
                  frame True {
                    # "開始找尋方塊"
                    n391 = local write "Block Find"(TRUE ("Block Find")) -> ()
                  }
                }
              }
              frame 28 {
                n392 = local read "Proc Finish"() -> (w1049:bool)
                n393 = Greater?(x=w1045, y=20.0) -> (0:w1046:bool)
                n394 = And(x=w1049, y=w1046) -> (x .and. y?=w1048:bool)
                n395 = case shown="True" w1048 {
                  tunnel: [w1052 30 ("f")] -> w1050
                  tunnel: w1044 -> [w1052 _]
                  frame False {
                  }
                  frame True {
                    # "開始找尋方塊"
                    n396 = local write "Block Find"(FALSE ("Block Find")) -> ()
                  }
                }
              }
              frame 30 {
                n397 = local read "Proc Finish"() -> (w1055:bool)
                n398 = Greater Or Equal?(x=w1059, y=3) -> (x >= y?=w1057:bool)
                n399 = And(x=w1055, y=w1057) -> (x .and. y?=w1056:bool)
                n400 = case shown="True" w1056 {
                  tunnel: w1061 -> [w1063 _]
                  tunnel: [w1063 w1064] -> w1060
                  frame False {
                  }
                  frame True {
                    w1066 = Operator_Loop_Mode."Idle" ("Operator Loop Mode")
                    n401 = local read "Block Array"() -> (w1069:dbl[][])
                    n402 = Array Size(array=w1069) -> (size(s)=w1068:i32[])
                    n403 = Index Array(array=w1068) -> (element=w1067:i32)  [unwired: 1 in]
                    n404 = Equal To 0?(x=w1067) -> (x = 0?=w1065:bool)
                    n405 = local write "Robot Mode:"(w1066) -> ()
                    n406 = shared-variable ".\\Operator Variables.lvlib\\Mode"(w1066) -> ()  [unwired: 1 in, 1 out]
                    n407 = case shown="True" w1065 {
                      tunnel: [90 40] -> w1064
                      frame False {
                        # "有發現方塊就離開"
                      }
                      frame True {
                        # "若沒有發現方塊\n就走到較寬的側邊"
                      }
                    }
                  }
                }
              }
              frame 40 {
                # "在左邊?"
                # "判斷靠地圖左邊或右邊,決定走到較寬的那一面"
                n408 = local read "Start POS"() -> (w1087:dbl[])
                n409 = Index Array(array=w1087) -> (element #1=w1074:dbl, element #2=w1072:dbl, element #3=w1076:dbl)  [unwired: 3 in]
                n410 = Less Or Equal?(x=w1074, y=1.15) -> (x <= y?=w1085:bool)
                n411 = Add(x=w1076, y=6.283185307179586) -> (x+y=w1089:dbl)
                n412 = Negate(x=w1089) -> (-x=w1088:dbl)
                n413 = Select(t=-0.4, s=w1085, f=0.4) -> (s? t:f=w1090:dbl)
                n414 = call-poly <vilib>:"2D Cartesian Coordinate Rotation.vi"("theta"=w1088, "y"=0.0, "x"=w1090) -> ("y out"=w1079:dbl, "x out"=w1078:dbl)  [unwired: 6 in, 1 out]
                n415 = Add(x=w1074, y=w1078) -> (x+y=w1080:dbl)
                n416 = Add(x=w1072, y=w1079) -> (x+y=w1077:dbl)
                n417 = Build Array(w1080, w1077) -> (w1073:dbl[])
                n418 = Build Array (concatenate)(w1073, w1076) -> (w1075:dbl[])
                n419 = shared-variable ".\\Operator Variables.lvlib\\SubGoal"(w1075) -> ()  [unwired: 1 in, 1 out]
              }
              frame 45 {
                n420 = local read "Proc Finish"() -> (w1093:bool)
                n421 = Greater Or Equal?(x=w1097, y=3) -> (x >= y?=w1095:bool)
                n422 = And(x=w1093, y=w1095) -> (x .and. y?=w1094:bool)
                n423 = case shown="True" w1094 {
                  tunnel: w1099 -> [w1101 _]
                  tunnel: [w1101 50] -> w1098
                  frame False {
                  }
                  frame True {
                    w1103 = Operator_Loop_Mode."Path Following" ("Operator Loop Mode")
                    n424 = local write "Robot Mode:"(w1103) -> ()
                    n425 = shared-variable ".\\Operator Variables.lvlib\\Mode"(w1103) -> ()  [unwired: 1 in, 1 out]
                  }
                }
              }
              frame 50 {
                n426 = local read "Proc Finish"() -> (w1104:bool)
                n427 = Greater Or Equal?(x=w1108, y=10) -> (x >= y?=w1106:bool)
                n428 = And(x=w1104, y=w1106) -> (x .and. y?=w1105:bool)
                n429 = case shown="True" w1105 {
                  tunnel: w1110 -> [w1112 _]
                  tunnel: [w1112 55] -> w1109
                  frame False {
                  }
                  frame True {
                    w1113 = Operator_Loop_Mode."Go Target" ("Operator Loop Mode")
                    n430 = local write "Robot Mode:"(w1113) -> ()
                    n431 = shared-variable ".\\Operator Variables.lvlib\\Mode"(w1113) -> ()  [unwired: 1 in, 1 out]
                  }
                }
              }
              frame 55 {
                n432 = local read "Proc Finish"() -> (w1115:bool)
                n433 = Greater Or Equal?(x=w1119, y=20) -> (x >= y?=w1117:bool)
                n434 = And(x=w1115, y=w1117) -> (x .and. y?=w1116:bool)
                n435 = case shown="True" w1116 {
                  tunnel: w1121 -> [w1123 _]
                  tunnel: [w1123 60] -> w1120
                  frame False {
                  }
                  frame True {
                    w1124 = Operator_Loop_Mode."Idle" ("Operator Loop Mode")
                    n436 = local write "Robot Mode:"(w1124) -> ()
                    n437 = shared-variable ".\\Operator Variables.lvlib\\Mode"(w1124) -> ()  [unwired: 1 in, 1 out]
                  }
                }
              }
              frame 60 {
                n438 = local read "Proc Finish"() -> (w1126:bool)
                n439 = Greater Or Equal?(x=w1130, y=5) -> (x >= y?=w1128:bool)
                n440 = And(x=w1126, y=w1128) -> (x .and. y?=w1127:bool)
                n441 = case shown="True" w1127 {
                  tunnel: w1132 -> [w1134 _]
                  tunnel: [w1134 65] -> w1131
                  frame False {
                  }
                  frame True {
                    # "開始找尋方塊"
                    n442 = local write "Block Find"(TRUE ("Block Find")) -> ()
                  }
                }
              }
              frame 65 {
                n443 = local read "Proc Finish"() -> (w1137:bool)
                n444 = Greater Or Equal?(x=w1141, y=10) -> (x >= y?=w1139:bool)
                n445 = And(x=w1137, y=w1139) -> (x .and. y?=w1138:bool)
                n446 = case shown="True" w1138 {
                  tunnel: w1143 -> [w1145 _]
                  tunnel: [w1145 90] -> w1142
                  frame False {
                  }
                  frame True {
                    # "結束找尋方塊"
                    n447 = local write "Block Find"(FALSE ("Block Find")) -> ()
                  }
                }
              }
              frame 90 {
              }
            }
          }
          frame 3 {
            # "ず"
            # "外"
            # "ず"
            # "外"
            # "沒有QR CODE的狀態,由出發區走出來,\n並做定位動作"
            n448 = case shown="10" w1155 {
              tunnel: w1155 -> [_ w1173 w1240]
              tunnel: w1154 -> [w1159 w1174 _]
              tunnel: [w1159 w1174 0] -> w1153
              tunnel: [10 w1172 w1240] -> w1152
              tunnel: w1151 -> [_ w1161 _]
              tunnel: w1150 -> [_ w1160 _]
              frame 0, Default {
                w1157 = 0.0 ("Proc Time")
                # "歸零抓取表"
                n449 = shared-variable ".\\Motor Control Variables.lvlib\\Odometry Data"() -> (w1156:dbl[])  [unwired: 1 in, 1 out]
                n450 = local write "Proc Index"(w1157) -> ()
                n451 = local write "Proc Time"(w1157) -> ()
                n452 = local write "Proc CMD"(w1157) -> ()
                n453 = shared-variable ".\\Operator Variables.lvlib\\SubGoal"(w1156) -> ()  [unwired: 1 in, 1 out]
              }
              frame 10 {
                n454 = local read "Proc Time"() -> (w1168:i16)
                n455 = local read "Proc Finish"() -> (w1163:bool)
                n456 = local read "Proc CMD"() -> (w1166:i16)
                n457 = Add(x=1.0 ("y"), y=w1168) -> (x+y=w1167:dbl)
                n458 = Greater?(x=w1161, y=w1167) -> (0:w1170:bool)
                n459 = Equal?(x=w1166, y=i16 1) -> (x = y?=w1164:bool)
                n460 = Or(x=w1164, y=w1163) -> (x .or. y?=w1162:bool)
                n461 = And(x=w1162, y=w1170) -> (x .and. y?=w1171:bool)
                n462 = case shown="True" w1171 {
                  tunnel: w1173 -> [w1175 w1183]
                  tunnel: [w1175 w1184] -> w1172
                  tunnel: w1161 -> [_ w1179]
                  tunnel: w1160 -> [_ w1178]
                  frame False {
                  }
                  frame True {
                    n463 = local read "Proc Catch Index"() -> (w1188:i16)
                    n464 = local read "Right Block"() -> (w1189:bool)
                    n465 = local read "Left Block"() -> (w1190:bool)
                    n466 = local read "Proc Index"() -> (w1187:i16)
                    n467 = Increment(x=w1187) -> (x+1=w1186:i16)
                    n468 = case shown="True" "Get off/Put on" {
                      tunnel: [w1191 w1206] -> w1180
                      tunnel: w1190 -> [w1196 w1205]
                      tunnel: w1189 -> [w1195 w1204]
                      tunnel: w1188 -> [w1197 w1203]
                      tunnel: w1187 -> [w1198 w1202]
                      tunnel: [w1193 w1201] -> w1177
                      tunnel: [w1192 w1200] -> w1176
                      tunnel: [w1194 w1199] -> w1185
                      frame True {
                        n469 = call "PutBlockTable.vi"("Right Block"=w1195, "Left Block"=w1196, "Catch Index"=w1197, "Proc Index"=w1198) -> ("Time"=w1191:i32, "B"=w1192:i32, "A"=w1193:i32, "CMD"=w1194:i32)  [unwired: 4 in]
                      }
                      frame False {
                        n470 = call "GetBlockTable.vi"("Right Block"=w1204, "Left Block"=w1205, "Catch Index"=w1203, "Proc Index"=w1202) -> ("Time"=w1206:i32, "B"=w1200:i32, "A"=w1201:i32, "CMD"=w1199:i32)  [unwired: 4 in]
                      }
                    }
                    n471 = local write "Proc Index"(w1186) -> ()
                    n472 = Add(x=w1180, y=w1179) -> (x+y=w1181:i32)
                    n473 = local write "Proc CMD"(w1185) -> ()
                    n474 = local write "Proc  VAL A"(w1177) -> ()
                    n475 = local write "Proc  VAL B"(w1176) -> ()
                    n476 = local write "Proc Time"(w1181) -> ()
                    n477 = case shown="92" w1185 {
                      tunnel: [w1207 w1209 w1211 w1223 w1229 w1233 w1235 90] -> w1184
                      tunnel: w1183 -> [w1207 w1209 w1211 w1223 w1229 w1233 w1235 _]
                      tunnel: w1178 -> [_ _ _ w1222 _ _ _ _]
                      tunnel: w1177 -> [_ _ _ w1220 _ _ _ _]
                      tunnel: w1176 -> [_ _ _ w1217 _ _ _ _]
                      frame 0, Default {
                        w1208 = Operator_Loop_Mode."Idle" ("Operator Loop Mode")
                        # "不做事"
                        n478 = local write "Robot Mode:"(w1208) -> ()
                        n479 = shared-variable ".\\Operator Variables.lvlib\\Mode"(w1208) -> ()  [unwired: 1 in, 1 out]
                      }
                      frame 1 {
                        w1210 = Operator_Loop_Mode."MoveTarget" ("Operator Loop Mode")
                        # "移動\n預計建立MoveTarget"
                        n480 = local write "Robot Mode:"(w1210) -> ()
                        n481 = shared-variable ".\\Operator Variables.lvlib\\Mode"(w1210) -> ()  [unwired: 1 in, 1 out]
                      }
                      frame 10 {
                        w1212 = Operator_Loop_Mode."moveblock" ("Operator Loop Mode")
                        # "移動\n用光感看黑在看白"
                        n482 = local write "Robot Mode:"(w1212) -> ()
                        n483 = shared-variable ".\\Operator Variables.lvlib\\Mode"(w1212) -> ()  [unwired: 1 in, 1 out]
                      }
                      frame 2..5 {
                        w1224 = Operator_Loop_Mode."Idle" ("Operator Loop Mode")
                        # "RC動作"
                        n484 = Equal?(x=w1220, y=90) -> (x = y?=w1218:bool)
                        n485 = call "RCservo.vi"("Value"=w1217, "ID"=w1220, "VISA resource name"=w1222) -> ("error out"=w1214:errorcluster, "VISA resource name out"=w1221:refnum<visa-resource-name>)  [unwired: 7 in]
                        n486 = local write "Robot Mode:"(w1224) -> ()
                        n487 = shared-variable ".\\Operator Variables.lvlib\\Mode"(w1224) -> ()  [unwired: 1 in, 1 out]
                        n488 = Subtract(x=3000, y=w1217) -> (x-y=w1215:i32)
                        n489 = local read "nowpos"() -> (w1213:dbl)
                        n490 = case shown="True" w1218 {
                          tunnel: w1221 -> [_ w1228]
                          tunnel: w1215 -> [_ w1227]
                          tunnel: w1214 -> [_ w1225]
                          frame False {
                          }
                          frame True {
                            n491 = call "RCservo.vi"("error in (no error)"=w1225, "Value"=w1227, "ID"=70, "VISA resource name"=w1228) -> ()  [unwired: 6 in, 2 out]
                          }
                        }
                        n492 = local write "OffsetZero"(w1213) -> ()
                      }
                      frame 90 {
                        w1230 = Operator_Loop_Mode."Block Correction" ("Operator Loop Mode")
                        n493 = local write "Robot Mode:"(w1230) -> ()
                        n494 = shared-variable ".\\Operator Variables.lvlib\\Mode"(w1230) -> ()  [unwired: 1 in, 1 out]
                      }
                      frame 91 {
                        w1231 = Operator_Loop_Mode."Idle" ("Operator Loop Mode")
                        n495 = shared-variable ".\\Operator Variables.lvlib\\SubGoal"() -> (w1232:dbl[])  [unwired: 1 in, 1 out]
                        n496 = local write "Block Fix array"(w1232) -> ()
                        n497 = local write "Robot Mode:"(w1231) -> ()
                        n498 = shared-variable ".\\Operator Variables.lvlib\\Mode"(w1231) -> ()  [unwired: 1 in, 1 out]
                      }
                      frame 92 {
                        w1236 = Operator_Loop_Mode."Idle" ("Operator Loop Mode")
                        n499 = shared-variable ".\\Motor Control Variables.lvlib\\Odometry Data"() -> (w1234:dbl[])  [unwired: 1 in, 1 out]
                        n500 = local write "Robot Mode:"(w1236) -> ()
                        n501 = shared-variable ".\\Operator Variables.lvlib\\Mode"(w1236) -> ()  [unwired: 1 in, 1 out]
                        n502 = shared-variable ".\\Operator Variables.lvlib\\SubGoal"(w1234) -> ()  [unwired: 1 in, 1 out]
                      }
                      frame 99 {
                        w1238 = Operator_Loop_Mode."Idle" ("Operator Loop Mode")
                        # "結束"
                        n503 = local write "Robot Mode:"(w1238) -> ()
                        n504 = shared-variable ".\\Operator Variables.lvlib\\Mode"(w1238) -> ()  [unwired: 1 in, 1 out]
                      }
                    }
                  }
                }
              }
              frame 90 {
              }
            }
          }
          frame 10 {
            # "ず"
            # "外"
            # "ず"
            # "外"
            # "找出下一個目標"
            n505 = case shown="85" w1246 {
              tunnel: w1246 -> [_ w1260 w1293 w1308 w1328 w1345 _ w1386 w1407 w1440 w1466 _ w1519 w1544 w1570 w1628 w1646 w1660 w1687 w1695]
              tunnel: w1245 -> [w1251 w1258 w1294 w1309 w1329 w1346 w1372 w1384 w1405 w1438 w1464 w1513 w1521 w1546 w1568 w1630 w1648 w1662 w1689 w1697]
              tunnel: [w1251 w1257 w1294 w1309 w1329 w1346 w1372 w1383 w1404 w1438 w1464 w1513 w1521 w1546 w1568 w1630 w1648 w1662 w1689 w1696] -> w1244
              tunnel: [10 w1259 w1292 w1307 w1327 w1344 w1367 w1385 w1406 w1439 w1465 80 w1520 w1545 w1569 w1629 w1647 w1661 w1688 w1694] -> w1243
              tunnel: w1241 -> [_ w1252 w1287 w1303 w1322 w1340 _ w1378 w1399 w1433 w1453 _ w1514 w1539 w1557 w1623 w1641 w1656 w1682 w1699]
              tunnel: w1242 -> [_ _ _ _ _ _ _ _ _ _ w1452 _ _ _ w1556 _ _ _ _ _]
              frame 0, Default {
                w1249 = Operator_Loop_Mode."WhereGo" ("Operator Loop Mode")
                # "執行尋找目標程式"
                n506 = local write "Enable ND"(TRUE ("Enable ND")) -> ()
                n507 = local write "Light"(0.0 ("Light")) -> ()
                n508 = local write "Robot Mode:"(w1249) -> ()
                n509 = shared-variable ".\\Operator Variables.lvlib\\Mode"(w1249) -> ()  [unwired: 1 in, 1 out]
              }
              frame 10 {
                n510 = local read "Proc Finish"() -> (w1256:bool)
                n511 = Greater?(x=w1252, y=2.0) -> (0:w1253:bool)
                n512 = And(x=w1256, y=w1253) -> (x .and. y?=w1255:bool)
                n513 = case shown="True" w1255 {
                  tunnel: w1260 -> [w1262 _]
                  tunnel: [w1262 15] -> w1259
                  tunnel: w1258 -> [w1261 w1267]
                  tunnel: [w1261 w1265] -> w1257
                  frame False {
                  }
                  frame True {
                    # "回家編號"
                    n514 = local read "Start Front"() -> (w1263:dbl[])
                    n515 = local read "Proc Block Index"() -> (w1278:i16)
                    n516 = local read "Block Array"() -> (w1286:dbl[][])
                    n517 = local read "Start POS"() -> (w1275:dbl[])
                    n518 = Not Equal?(x=w1278, y=i16 99) -> (x != y?=w1264:bool)
                    n519 = Index Array(array=w1286, index (row)=w1278) -> (element=w1285:dbl[])  [unwired: 1 in]
                    n520 = Index Array(array=w1285, index #1=6 ("index"), index #2=7 ("index"), index #3=8 ("index")) -> (element #1=w1279:dbl, element #2=w1280:dbl, element #3=w1281:dbl)
                    n521 = Build Array(w1279, w1280, w1281) -> (w1276:dbl[])
                    n522 = Index Array(array=w1263) -> (element #1=w1273:dbl, element #2=w1272:dbl)  [unwired: 2 in]
                    n523 = Index Array(array=w1275, index=2) -> (element=w1271:dbl)
                    n524 = Build Array(w1273, w1272, w1271) -> (w1270:dbl[])
                    n525 = Select(t=w1276, s=w1264, f=w1270) -> (s? t:f=w1269:dbl[])
                    n526 = shared-variable ".\\Operator Variables.lvlib\\SubGoal"(w1269) -> ()  [unwired: 1 in, 1 out]
                    n527 = Select(t=w1267, s=w1264, f=100) -> (s? t:f=w1265:i32)
                  }
                }
              }
              frame 15 {
                n528 = local read "Proc Finish"() -> (w1291:bool)
                n529 = Greater?(x=w1287, y=2.0) -> (0:w1288:bool)
                n530 = And(x=w1291, y=w1288) -> (x .and. y?=w1290:bool)
                n531 = case shown="True" w1290 {
                  tunnel: w1293 -> [w1295 _]
                  tunnel: [w1295 20] -> w1292
                  frame False {
                  }
                  frame True {
                    w1296 = Operator_Loop_Mode."Path Following" ("Operator Loop Mode")
                    # "避障行走到目標"
                    n532 = local write "Robot Mode:"(w1296) -> ()
                    n533 = shared-variable ".\\Operator Variables.lvlib\\Mode"(w1296) -> ()  [unwired: 1 in, 1 out]
                  }
                }
              }
              frame 20 {
                # "無法接近目標超過n秒,就結束等待"
                n534 = local read "GoFarSec"() -> (w1302:u64)
                n535 = local read "Proc Finish"() -> (w1306:bool)
                n536 = Greater?(x=w1302, y=u64 15) -> (0:w1298:bool)
                n537 = Greater?(x=w1303, y=10.0) -> (0:w1304:bool)
                n538 = And(x=w1306, y=w1304) -> (x .and. y?=w1300:bool)
                n539 = Or(x=w1298, y=w1300) -> (x .or. y?=w1299:bool)
                n540 = case shown="True" w1299 {
                  tunnel: w1308 -> [w1310 _]
                  tunnel: [w1310 w1312] -> w1307
                  tunnel: w1298 -> [_ w1311]
                  frame False {
                  }
                  frame True {
                    n541 = case shown="True" w1311 {
                      tunnel: [25 15] -> w1312
                      frame False {
                        w1314 = Operator_Loop_Mode."Go Target" ("Operator Loop Mode")
                        # "面向目標定位"
                        n542 = local write "Robot Mode:"(w1314) -> ()
                        n543 = shared-variable ".\\Operator Variables.lvlib\\Mode"(w1314) -> ()  [unwired: 1 in, 1 out]
                      }
                      frame True {
                        w1320 = Operator_Loop_Mode."Idle" ("Operator Loop Mode")
                        # "跳回去執行Path Following"
                        # "超過時間,例外處裡"
                        n544 = local read "Proc Block Index"() -> (w1318:i16)
                        n545 = local read "Block Array"() -> (w1319:dbl[][])
                        n546 = local read "Block Color"() -> (w1316:i16[][])
                        n547 = call "WhereExit.vi"("Block Array"=w1319, "Block Color"=w1316, "Proc Block Index"=w1318) -> ("Target Index"=w1315:i32, "Target POS"=w1317:dbl[])  [unwired: 6 in]
                        n548 = local write "Proc Block Index"(w1315) -> ()
                        n549 = shared-variable ".\\Operator Variables.lvlib\\SubGoal"(w1317) -> ()  [unwired: 1 in, 1 out]
                        n550 = local write "Robot Mode:"(w1320) -> ()
                        n551 = shared-variable ".\\Operator Variables.lvlib\\Mode"(w1320) -> ()  [unwired: 1 in, 1 out]
                      }
                    }
                  }
                }
              }
              frame 25 {
                n552 = local read "Proc Finish"() -> (w1326:bool)
                n553 = Greater?(x=w1322, y=10.0) -> (0:w1323:bool)
                n554 = And(x=w1326, y=w1323) -> (x .and. y?=w1325:bool)
                n555 = case shown="True" w1325 {
                  tunnel: w1328 -> [w1330 _]
                  tunnel: [w1330 30] -> w1327
                  frame False {
                  }
                  frame True {
                    w1333 = Operator_Loop_Mode."Block Correction" ("Operator Loop Mode")
                    # "對正目標"
                    n556 = local read "Light Set"() -> (w1332:dbl)
                    n557 = local write "Block Face"(0.0 ("Block Face")) -> ()
                    n558 = local write "Light"(w1332) -> ()
                    n559 = local write "Robot Mode:"(w1333) -> ()
                    n560 = shared-variable ".\\Operator Variables.lvlib\\Mode"(w1333) -> ()  [unwired: 1 in, 1 out]
                  }
                }
              }
              frame 30 {
                # "若是面對的寬度大於240mm,\n表示可能面對牆壁,要例外處裡"
                n561 = local read "Proc Finish"() -> (w1336:bool)
                n562 = local read "Block Face"() -> (w1339:dbl)
                n563 = Greater?(x=w1339, y=240.0) -> (0:w1337:bool)
                n564 = Greater?(x=w1340, y=10.0) -> (0:w1341:bool)
                n565 = Or(x=w1337, y=w1336) -> (x .or. y?=w1335:bool)
                n566 = And(x=w1335, y=w1341) -> (x .and. y?=w1343:bool)
                n567 = case shown="True" w1343 {
                  tunnel: w1345 -> [w1347 _]
                  tunnel: [w1347 w1348] -> w1344
                  frame False {
                  }
                  frame True {
                    n568 = local read "Block Face"() -> (w1350:dbl)
                    n569 = Less Or Equal?(x=w1350, y=240.0) -> (x <= y?=w1349:bool)
                    n570 = case shown="True" w1349 {
                      tunnel: [90 35] -> w1348
                      frame False {
                        w1357 = Operator_Loop_Mode."Idle" ("Operator Loop Mode")
                        # "把這個位置由陣列拿掉,直接回頭離開"
                        n571 = local read "Block Array"() -> (w1356:dbl[][])
                        n572 = local read "Proc Block Index"() -> (w1354:i16)
                        n573 = Delete From Array(array=w1356, length=1, index (row)=w1354) -> (array with subset deleted=w1353:dbl[][])  [unwired: 1 in, 1 out]
                        n574 = local write "Robot Mode:"(w1357) -> ()
                        n575 = shared-variable ".\\Operator Variables.lvlib\\Mode"(w1357) -> ()  [unwired: 1 in, 1 out]
                        n576 = local write "Block Array"(w1353) -> ()
                      }
                      frame True {
                        w1363 = Operator_Loop_Mode."Idle" ("Operator Loop Mode")
                        # "校正X,Y,Z"
                        n577 = shared-variable ".\\Operator Variables.lvlib\\SubGoal"() -> (w1358:dbl[])  [unwired: 1 in, 1 out]
                        n578 = call "POS_Back.vi"("BackDistance"=-0.05, "POS"=w1358) -> ("Offset"=→"Offset":dbl[], "POS N"=w1361:dbl[])  [unwired: 8 in]
                        n579 = local write "Robot Mode:"(w1363) -> ()
                        n580 = shared-variable ".\\Operator Variables.lvlib\\Mode"(w1363) -> ()  [unwired: 1 in, 1 out]
                        n581 = local write "Block Fix array"(w1361) -> ()
                      }
                    }
                  }
                }
              }
              frame 35 {
                # "還沒來過,不知道顏色"
                n582 = local read "Proc Block Index"() -> (w1370:i16)
                n583 = local read "Block Color"() -> (w1371:i16[][])
                n584 = Index Array(array=w1371, index (row)=w1370) -> (element=w1366:i16[])  [unwired: 1 in]
                n585 = Index Array(array=w1366) -> (element #1=w1364:i16, element #2=w1365:i16)  [unwired: 2 in]
                n586 = local write "Up Color"(w1365) -> ()
                n587 = local write "Down Color"(w1364) -> ()
                n588 = Equal To 0?(x=w1364) -> (x = 0?=w1368:bool)
                n589 = case shown="False" w1368 {
                  tunnel: [Operator_Loop_Mode."Idle" ("Operator Loop Mode") Operator_Loop_Mode."Get Color" ("Operator Loop Mode")] -> w1369
                  tunnel: [40 37] -> w1367
                  frame False {
                    # "直接判斷是否取方塊"
                    n590 = local write "Light"(0.0 ("Light")) -> ()
                  }
                  frame True {
                    # "考慮是否點燈"
                    # "取方塊程序"
                  }
                }
                n591 = local write "Robot Mode:"(w1369) -> ()
                n592 = shared-variable ".\\Operator Variables.lvlib\\Mode"(w1369) -> ()  [unwired: 1 in, 1 out]
              }
              frame 37 {
                n593 = local read "Proc Finish"() -> (w1382:bool)
                n594 = Greater?(x=w1378, y=5.0) -> (0:w1379:bool)
                n595 = And(x=w1382, y=w1379) -> (x .and. y?=w1381:bool)
                n596 = case shown="True" w1381 {
                  tunnel: w1386 -> [w1388 _]
                  tunnel: [w1388 40] -> w1385
                  tunnel: w1384 -> [w1387 w1392]
                  tunnel: [w1387 w1392] -> w1383
                  frame False {
                  }
                  frame True {
                    # "存入方塊上下顏色"
                    n597 = local write "Light"(0.0 ("Light")) -> ()
                    n598 = local read "Block Color"() -> (w1389:i16[][])
                    n599 = local read "Proc Block Index"() -> (w1397:i16)
                    n600 = local read "Down Color"() -> (w1396:i32)
                    n601 = local read "Up Color"() -> (w1395:i32)
                    n602 = Build Array(w1396, w1395, 0 ("element")) -> (w1394:i32[])
                    n603 = Replace Array Subset(array=w1389, new element=w1394, index (row)=w1397) -> (w1393:i16[][])  [unwired: 1 in]
                    n604 = local write "Block Color"(w1393) -> ()
                  }
                }
              }
              frame 40 {
                n605 = local read "Proc Finish"() -> (w1403:bool)
                n606 = Greater?(x=w1399, y=3.0) -> (0:w1400:bool)
                n607 = And(x=w1403, y=w1400) -> (x .and. y?=w1402:bool)
                n608 = case shown="True" w1402 {
                  tunnel: w1407 -> [w1409 _]
                  tunnel: [w1409 w1421] -> w1406
                  tunnel: w1405 -> [w1408 w1420]
                  tunnel: [w1408 w1422] -> w1404
                  frame False {
                  }
                  frame True {
                    # "當下方顏色不是我們要處裡的"
                    # "當設定為不處裡方塊"
                    # "找不到空爪子"
                    n609 = local read "Proc Down Color"() -> (w1413:i32)
                    n610 = local read "Right Block"() -> (w1417:bool)
                    n611 = local read "Down Color"() -> (w1412:i32)
                    n612 = local read "Up Color"() -> (w1418:i32)
                    n613 = local read "Catch Color"() -> (w1428:i16[])
                    n614 = local read "Left Block"() -> (w1416:bool)
                    n615 = local write "Block Find"(FALSE ("Block Find")) -> ()
                    n616 = Not Equal?(x=w1412, y=w1413) -> (x != y?=w1411:bool)
                    n617 = call "GetEmptyCatchIndex.vi"("Right Block"=w1417, "Left Block"=w1416, "Up Color"=w1418, "Down Color"=w1412, "Catch Color"=w1428) -> ("Empty Catch Index"=w1427:i16)  [unwired: 5 in, 1 out]
                    n618 = local write "Proc Catch Index"(w1427) -> ()
                    n619 = Compound Arithmetic op=OR(w1411, FALSE ("value"), "no get") -> (w1419:bool)
                    n620 = Not Equal?(x=w1427, y=i16 99) -> (x != y?=w1424:bool)
                    n621 = Select(t=w1420, s=w1424, f=100) -> (s? t:f=w1423:i32)
                    n622 = case shown="False" w1419 {
                      tunnel: w1423 -> [w1430 _]
                      tunnel: [w1430 w1432] -> w1422
                      tunnel: [42 90] -> w1421
                      tunnel: w1420 -> [_ w1432]
                      frame False {
                        # "執行拿方塊"
                      }
                      frame True {
                        # "這個方塊不處裡"
                      }
                    }
                  }
                }
              }
              frame 42 {
                n623 = local read "Proc Finish"() -> (w1437:bool)
                n624 = Greater?(x=w1433, y=5.0) -> (0:w1434:bool)
                n625 = And(x=w1437, y=w1434) -> (x .and. y?=w1436:bool)
                n626 = case shown="True" w1436 {
                  tunnel: w1440 -> [w1441 _]
                  tunnel: [w1441 w1449] -> w1439
                  frame False {
                  }
                  frame True {
                    w1445 = 0.0 ("Proc Time")
                    w1448 = Operator_Loop_Mode."Idle" ("Operator Loop Mode")
                    # "設定下一個要找的大方塊顏色"
                    # "歸零抓取表"
                    # "將方塊顏色放入相對應爪子位置"
                    n627 = local read "Proc Catch Index"() -> (w1446:i16)
                    n628 = local read "Catch Color"() -> (w1447:i16[])
                    n629 = local read "Up Color"() -> (w1443:i32)
                    n630 = local write "Proc Index"(w1445) -> ()
                    n631 = local write "Proc Time"(w1445) -> ()
                    n632 = local write "Proc CMD"(w1445) -> ()
                    n633 = Replace Array Subset(array=w1447, new element=w1443, index=w1446) -> (w1444:i16[])
                    n634 = local write "Proc Down Color"(w1443) -> ()
                    n635 = local write "Catch Color"(w1444) -> ()
                    n636 = local write "Robot Mode:"(w1448) -> ()
                    n637 = shared-variable ".\\Operator Variables.lvlib\\Mode"(w1448) -> ()  [unwired: 1 in, 1 out]
                    n638 = case shown="False" "get over" {
                      tunnel: [45 70] -> w1449
                      frame False {
                      }
                      frame True {
                      }
                    }
                  }
                }
              }
              frame 45 {
                n639 = local read "Proc Finish"() -> (w1455:bool)
                n640 = local read "Proc CMD"() -> (w1458:i16)
                n641 = local read "Proc Time"() -> (w1459:i16)
                n642 = Add(x=1.0 ("y"), y=w1459) -> (x+y=w1460:dbl)
                n643 = Greater?(x=w1453, y=w1460) -> (0:w1462:bool)
                n644 = Equal?(x=w1458, y=i16 1) -> (x = y?=w1456:bool)
                n645 = Or(x=w1456, y=w1455) -> (x .or. y?=w1454:bool)
                n646 = And(x=w1454, y=w1462) -> (x .and. y?=w1463:bool)
                n647 = case shown="True" w1463 {
                  tunnel: w1466 -> [w1467 w1474]
                  tunnel: [w1467 w1475] -> w1465
                  tunnel: w1453 -> [_ w1471]
                  tunnel: w1452 -> [_ w1470]
                  frame False {
                  }
                  frame True {
                    # "RC動作"
                    # "這裡開始應該開始執行取方塊"
                    n648 = local read "Proc Catch Index"() -> (w1479:i16)
                    n649 = local read "Right Block"() -> (w1480:bool)
                    n650 = local read "Left Block"() -> (w1481:bool)
                    n651 = local read "Proc Index"() -> (w1478:i16)
                    n652 = Increment(x=w1478) -> (x+1=w1477:i16)
                    n653 = call "GetBlockTable.vi"("Right Block"=w1480, "Left Block"=w1481, "Catch Index"=w1479, "Proc Index"=w1478) -> ("Time"=w1473:i32, "B"=w1468:i32, "A"=w1469:i32, "CMD"=w1476:i32)  [unwired: 4 in]
                    n654 = local write "Proc Index"(w1477) -> ()
                    n655 = Add(x=w1473, y=w1471) -> (x+y=w1472:i32)
                    n656 = local write "Proc Time"(w1472) -> ()
                    n657 = local write "Proc CMD"(w1476) -> ()
                    n658 = local write "Proc  VAL A"(w1469) -> ()
                    n659 = local write "Proc  VAL B"(w1468) -> ()
                    n660 = case shown="91" w1476 {
                      tunnel: [w1482 w1484 w1496 w1501 w1508 70] -> w1475
                      tunnel: w1474 -> [w1482 w1484 w1496 w1501 w1508 _]
                      tunnel: w1470 -> [_ _ w1488 _ _ _]
                      tunnel: w1469 -> [_ _ w1487 _ _ _]
                      tunnel: w1468 -> [_ _ w1486 _ _ _]
                      frame 0, Default {
                        w1483 = Operator_Loop_Mode."Idle" ("Operator Loop Mode")
                        # "不做事"
                        n661 = local write "Robot Mode:"(w1483) -> ()
                        n662 = shared-variable ".\\Operator Variables.lvlib\\Mode"(w1483) -> ()  [unwired: 1 in, 1 out]
                      }
                      frame 1 {
                        w1485 = Operator_Loop_Mode."MoveTarget" ("Operator Loop Mode")
                        # "移動\n預計建立MoveTarget"
                        n663 = local write "Robot Mode:"(w1485) -> ()
                        n664 = shared-variable ".\\Operator Variables.lvlib\\Mode"(w1485) -> ()  [unwired: 1 in, 1 out]
                      }
                      frame 2..6 {
                        w1489 = Operator_Loop_Mode."Idle" ("Operator Loop Mode")
                        n665 = Equal?(x=w1487, y=90) -> (x = y?=w1492:bool)
                        n666 = call "RCservo.vi"("Value"=w1486, "ID"=w1487, "VISA resource name"=w1488) -> ("error out"=w1495:errorcluster, "VISA resource name out"=w1490:refnum<visa-resource-name>)  [unwired: 7 in]
                        n667 = local write "Robot Mode:"(w1489) -> ()
                        n668 = shared-variable ".\\Operator Variables.lvlib\\Mode"(w1489) -> ()  [unwired: 1 in, 1 out]
                        n669 = Subtract(x=3000, y=w1486) -> (x-y=w1494:i32)
                        n670 = case shown="True" w1492 {
                          tunnel: w1490 -> [_ w1500]
                          tunnel: w1494 -> [_ w1499]
                          tunnel: w1495 -> [_ w1497]
                          frame False {
                          }
                          frame True {
                            n671 = call "RCservo.vi"("error in (no error)"=w1497, "Value"=w1499, "ID"=70, "VISA resource name"=w1500) -> ()  [unwired: 6 in, 2 out]
                          }
                        }
                      }
                      frame 90 {
                        w1502 = Operator_Loop_Mode."Block Correction" ("Operator Loop Mode")
                        n672 = local write "Robot Mode:"(w1502) -> ()
                        n673 = shared-variable ".\\Operator Variables.lvlib\\Mode"(w1502) -> ()  [unwired: 1 in, 1 out]
                      }
                      frame 91 {
                        w1507 = Operator_Loop_Mode."Idle" ("Operator Loop Mode")
                        n674 = shared-variable ".\\Operator Variables.lvlib\\SubGoal"() -> (w1506:dbl[])  [unwired: 1 in, 1 out]
                        n675 = call "POS_Back.vi"("BackDistance"=-0.05, "POS"=w1506) -> ("Offset"=w1503:dbl[], "POS N"=w1505:dbl[])  [unwired: 8 in]
                        n676 = local write "Robot Mode:"(w1507) -> ()
                        n677 = shared-variable ".\\Operator Variables.lvlib\\Mode"(w1507) -> ()  [unwired: 1 in, 1 out]
                        n678 = local write "Block Fix array"(w1505) -> ()
                        n679 = local write "Offset"(w1503) -> ()
                      }
                      frame 99 {
                        w1511 = Operator_Loop_Mode."Idle" ("Operator Loop Mode")
                        # "結束"
                        n680 = local write "Robot Mode:"(w1511) -> ()
                        n681 = shared-variable ".\\Operator Variables.lvlib\\Mode"(w1511) -> ()  [unwired: 1 in, 1 out]
                        n682 = local write "get over"(TRUE ("get over")) -> ()
                      }
                    }
                  }
                }
              }
              frame 70 {
              }
              frame 80 {
                n683 = local read "Proc Finish"() -> (w1518:bool)
                n684 = Greater?(x=w1514, y=5.0) -> (0:w1515:bool)
                n685 = And(x=w1518, y=w1515) -> (x .and. y?=w1517:bool)
                n686 = case shown="True" w1517 {
                  tunnel: w1519 -> [w1522 _]
                  tunnel: [w1522 w1534] -> w1520
                  frame False {
                  }
                  frame True {
                    w1538 = Operator_Loop_Mode."Idle" ("Operator Loop Mode")
                    # "放置次數小於兩次時,可以再放"
                    # "找手上出是否有方塊可以放"
                    n687 = local read "Proc Block Index"() -> (w1531:i16)
                    n688 = local read "Block Color"() -> (w1530:i16[][])
                    n689 = local read "Put Counter"() -> (w1526:i32)
                    n690 = Index Array(array=w1530, index (row)=w1531) -> (element=w1529:i16[])  [unwired: 1 in]
                    n691 = local read "Catch Color"() -> (w1537:i16[])
                    n692 = Less?(x=w1526, y=2) -> (x < y?=w1524:bool)
                    n693 = Index Array(array=w1529) -> (element #1=w1523:i16)  [unwired: 3 in, 2 out]
                    n694 = call "GetColorCatchIndex.vi"("Catch Color"=w1537, "Color"=w1523) -> ("Catch Color Index"=w1533:i16)  [unwired: 9 in]
                    n695 = local write "Proc Catch Index"(w1533) -> ()
                    n696 = Not Equal?(x=w1533, y=i16 99) -> (x != y?=w1528:bool)
                    n697 = And(x=w1528, y=w1524) -> (x .and. y?=w1527:bool)
                    n698 = local write "Robot Mode:"(w1538) -> ()
                    n699 = shared-variable ".\\Operator Variables.lvlib\\Mode"(w1538) -> ()  [unwired: 1 in, 1 out]
                    n700 = Select(t=82, s=w1527, f=90) -> (s? t:f=w1534:i32)
                  }
                }
              }
              frame 82 {
                n701 = local read "Proc Finish"() -> (w1543:bool)
                n702 = Greater?(x=w1539, y=i16 5) -> (0:w1540:bool)
                n703 = And(x=w1543, y=w1540) -> (x .and. y?=w1542:bool)
                n704 = case shown="True" w1542 {
                  tunnel: w1544 -> [w1547 _]
                  tunnel: [w1547 85] -> w1545
                  frame False {
                  }
                  frame True {
                    w1550 = i16 0 ("Proc Time")
                    # "抓取計數加一"
                    # "歸零抓取表"
                    # "將相對應爪子位置,清成空(0)"
                    n705 = local read "Proc Catch Index"() -> (w1553:i16)
                    n706 = local read "Catch Color"() -> (w1554:i16[])
                    n707 = local read "Put Counter"() -> (w1549:i32)
                    n708 = Replace Array Subset(array=w1554, new element=i16 0 ("new element/subarray"), index=w1553) -> (w1552:i16[])
                    n709 = Increment(x=w1549) -> (x+1=w1548:i32)
                    n710 = local write "Put Counter"(w1548) -> ()
                    n711 = local write "Proc Index"(w1550) -> ()
                    n712 = local write "Proc Time"(w1550) -> ()
                    n713 = local write "Catch Color"(w1552) -> ()
                  }
                }
              }
              frame 85 {
                n714 = local read "Proc CMD"() -> (w1562:i16)
                n715 = local read "Proc Finish"() -> (w1559:bool)
                n716 = local read "Proc Time"() -> (w1564:i16)
                n717 = Add(x=i16 1 ("y"), y=w1564) -> (x+y=w1563:i16)
                n718 = Greater?(x=w1557, y=w1563) -> (0:w1566:bool)
                n719 = Equal?(x=w1562, y=i16 1) -> (x = y?=w1560:bool)
                n720 = Or(x=w1560, y=w1559) -> (x .or. y?=w1558:bool)
                n721 = And(x=w1558, y=w1566) -> (x .and. y?=w1567:bool)
                n722 = case shown="True" w1567 {
                  tunnel: w1570 -> [w1571 w1584]
                  tunnel: [w1571 w1585] -> w1569
                  tunnel: w1557 -> [_ w1576]
                  tunnel: w1556 -> [_ w1575]
                  frame False {
                  }
                  frame True {
                    # "這裡開始應該開始執行放方塊"
                    n723 = local read "Proc Catch Index"() -> (w1581:i16)
                    n724 = local read "OffsetZero"() -> (w1572:i32)
                    n725 = local read "Right Block"() -> (w1583:bool)
                    n726 = local read "Left Block"() -> (w1580:bool)
                    n727 = local read "Proc Index"() -> (w1582:i16)
                    n728 = Increment(x=w1582) -> (x+1=w1586:i16)
                    n729 = call "PutBlockTable.vi"("Numeric"=w1572, "Right Block"=w1583, "Left Block"=w1580, "Catch Index"=w1581, "Proc Index"=w1582) -> ("Time"=w1578:i32, "B"=w1573:i32, "A"=w1574:i32, "CMD"=w1579:i32)  [unwired: 3 in]
                    n730 = Add(x=w1578, y=w1576) -> (x+y=w1577:i32)
                    n731 = local write "Proc Index"(w1586) -> ()
                    n732 = local write "Proc Time"(w1577) -> ()
                    n733 = local write "Proc CMD"(w1579) -> ()
                    n734 = local write "Proc  VAL A"(w1574) -> ()
                    n735 = local write "Proc  VAL B"(w1573) -> ()
                    n736 = case shown="92" w1579 {
                      tunnel: [w1588 w1590 w1603 w1608 w1610 w1613 w1620 90] -> w1585
                      tunnel: w1584 -> [w1588 w1590 w1603 w1608 w1610 w1613 w1620 _]
                      tunnel: w1575 -> [_ _ w1593 _ _ _ _ _]
                      tunnel: w1574 -> [_ _ w1595 _ _ _ _ _]
                      tunnel: w1573 -> [_ _ w1594 _ _ _ _ _]
                      frame 0, Default {
                        w1589 = Operator_Loop_Mode."Idle" ("Operator Loop Mode")
                        # "不做事"
                        n737 = local write "Robot Mode:"(w1589) -> ()
                        n738 = shared-variable ".\\Operator Variables.lvlib\\Mode"(w1589) -> ()  [unwired: 1 in, 1 out]
                        n739 = local write "OffsetZero"(0 ("OffsetZero")) -> ()
                      }
                      frame 1 {
                        w1591 = Operator_Loop_Mode."MoveTarget" ("Operator Loop Mode")
                        # "移動\n預計建立MoveTarget"
                        n740 = local write "Robot Mode:"(w1591) -> ()
                        n741 = shared-variable ".\\Operator Variables.lvlib\\Mode"(w1591) -> ()  [unwired: 1 in, 1 out]
                      }
                      frame 2..4 {
                        w1596 = Operator_Loop_Mode."Idle" ("Operator Loop Mode")
                        # "RC動作"
                        n742 = Equal?(x=w1595, y=90) -> (x = y?=w1599:bool)
                        n743 = call "RCservo.vi"("Value"=w1594, "ID"=w1595, "VISA resource name"=w1593) -> ("error out"=w1602:errorcluster, "VISA resource name out"=w1597:refnum<visa-resource-name>)  [unwired: 7 in]
                        n744 = local write "Robot Mode:"(w1596) -> ()
                        n745 = shared-variable ".\\Operator Variables.lvlib\\Mode"(w1596) -> ()  [unwired: 1 in, 1 out]
                        n746 = Subtract(x=3000, y=w1594) -> (x-y=w1601:i32)
                        n747 = case shown="True" w1599 {
                          tunnel: w1597 -> [_ w1607]
                          tunnel: w1601 -> [_ w1606]
                          tunnel: w1602 -> [_ w1604]
                          frame False {
                          }
                          frame True {
                            n748 = call "RCservo.vi"("error in (no error)"=w1604, "Value"=w1606, "ID"=70, "VISA resource name"=w1607) -> ()  [unwired: 6 in, 2 out]
                          }
                        }
                        n749 = local read "nowpos"() -> (w1592:dbl)
                        n750 = local write "OffsetZero"(w1592) -> ()
                      }
                      frame 10 {
                        w1609 = Operator_Loop_Mode."moveblock" ("Operator Loop Mode")
                        # "移動\n預計建立MoveTarget"
                        n751 = local write "Robot Mode:"(w1609) -> ()
                        n752 = shared-variable ".\\Operator Variables.lvlib\\Mode"(w1609) -> ()  [unwired: 1 in, 1 out]
                      }
                      frame 90 {
                        w1611 = Operator_Loop_Mode."Block Correction" ("Operator Loop Mode")
                        n753 = local write "Robot Mode:"(w1611) -> ()
                        n754 = shared-variable ".\\Operator Variables.lvlib\\Mode"(w1611) -> ()  [unwired: 1 in, 1 out]
                      }
                      frame 91 {
                        w1612 = Operator_Loop_Mode."Idle" ("Operator Loop Mode")
                        # "校正X,Y,Z"
                        n755 = shared-variable ".\\Operator Variables.lvlib\\SubGoal"() -> (w1614:dbl[])  [unwired: 1 in, 1 out]
                        n756 = local write "Robot Mode:"(w1612) -> ()
                        n757 = shared-variable ".\\Operator Variables.lvlib\\Mode"(w1612) -> ()  [unwired: 1 in, 1 out]
                        n758 = call "POS_Back.vi"("BackDistance"=-0.05, "POS"=w1614) -> ("Offset"=w1617:dbl[], "POS N"=w1615:dbl[])  [unwired: 8 in]
                        n759 = local write "Block Fix array"(w1615) -> ()
                        n760 = local write "Offset"(w1617) -> ()
                      }
                      frame 92 {
                        w1619 = Operator_Loop_Mode."Idle" ("Operator Loop Mode")
                        n761 = shared-variable ".\\Motor Control Variables.lvlib\\Odometry Data"() -> (w1618:dbl[])  [unwired: 1 in, 1 out]
                        n762 = local write "Robot Mode:"(w1619) -> ()
                        n763 = shared-variable ".\\Operator Variables.lvlib\\Mode"(w1619) -> ()  [unwired: 1 in, 1 out]
                        n764 = shared-variable ".\\Operator Variables.lvlib\\SubGoal"(w1618) -> ()  [unwired: 1 in, 1 out]
                      }
                      frame 99 {
                        w1622 = Operator_Loop_Mode."Idle" ("Operator Loop Mode")
                        # "結束"
                        n765 = local write "Robot Mode:"(w1622) -> ()
                        n766 = shared-variable ".\\Operator Variables.lvlib\\Mode"(w1622) -> ()  [unwired: 1 in, 1 out]
                      }
                    }
                  }
                }
              }
              frame 90 {
                n767 = local read "Proc Finish"() -> (w1627:bool)
                n768 = Greater?(x=w1623, y=2.0) -> (0:w1624:bool)
                n769 = And(x=w1627, y=w1624) -> (x .and. y?=w1626:bool)
                n770 = case shown="True" w1626 {
                  tunnel: w1628 -> [w1631 _]
                  tunnel: [w1631 94] -> w1629
                  frame False {
                  }
                  frame True {
                    w1640 = Operator_Loop_Mode."Idle" ("Operator Loop Mode")
                    # "準備轉身"
                    n771 = shared-variable ".\\Motor Control Variables.lvlib\\Odometry Data"() -> (w1639:dbl[])  [unwired: 1 in, 1 out]
                    n772 = Index Array(array=w1639) -> (element #1=w1638:dbl, element #2=w1637:dbl, element #3=w1636:dbl)  [unwired: 3 in]
                    n773 = Add(x=w1636, y=3.141592653589793) -> (x+y=w1634:dbl)
                    n774 = Build Array(w1638, w1637, w1634) -> (w1633:dbl[])
                    n775 = shared-variable ".\\Operator Variables.lvlib\\SubGoal"(w1633) -> ()  [unwired: 1 in, 1 out]
                    n776 = local write "Robot Mode:"(w1640) -> ()
                    n777 = shared-variable ".\\Operator Variables.lvlib\\Mode"(w1640) -> ()  [unwired: 1 in, 1 out]
                  }
                }
              }
              frame 94 {
                n778 = local read "Proc Finish"() -> (w1645:bool)
                n779 = Greater?(x=w1641, y=2.0) -> (0:w1642:bool)
                n780 = And(x=w1645, y=w1642) -> (x .and. y?=w1644:bool)
                n781 = case shown="True" w1644 {
                  tunnel: w1646 -> [w1649 _]
                  tunnel: [w1649 96] -> w1647
                  frame False {
                  }
                  frame True {
                    w1651 = Operator_Loop_Mode."Go Target" ("Operator Loop Mode")
                    # "執行轉身"
                    n782 = local write "Robot Mode:"(w1651) -> ()
                    n783 = shared-variable ".\\Operator Variables.lvlib\\Mode"(w1651) -> ()  [unwired: 1 in, 1 out]
                  }
                }
              }
              frame 96 {
                n784 = local read "QR_CAM"() -> (w1655:bool)
                n785 = local read "Proc Finish"() -> (w1659:bool)
                n786 = Select(t=5.0, s=w1655, f=5.0 ("y")) -> (s? t:f=w1652:dbl)
                n787 = Greater?(x=w1656, y=w1652) -> (0:w1657:bool)
                n788 = And(x=w1659, y=w1657) -> (x .and. y?=w1658:bool)
                n789 = case shown="True" w1658 {
                  tunnel: w1660 -> [w1663 _]
                  tunnel: [w1663 w1672] -> w1661
                  frame False {
                  }
                  frame True {
                    w1681 = Operator_Loop_Mode."Idle" ("Operator Loop Mode")
                    # "若是沒有接下來的方塊可以處裡,準備再找一次方塊"
                    # "做一次Find Block"
                    # "回到找下一個目標"
                    n790 = local read "Block Array"() -> (w1667:dbl[][])
                    n791 = local read "Proc Block Index"() -> (w1678:i16)
                    n792 = Array Size(array=w1667) -> (size(s)=w1680:i32[])
                    n793 = local read "QR_CAM"() -> (w1675:bool)
                    n794 = Index Array(array=w1680) -> (element=w1677:i32)  [unwired: 1 in]
                    n795 = Increment(x=w1678) -> (x+1=w1676:i16)
                    n796 = Less Or Equal?(x=w1677, y=4) -> (x <= y?=w1665:bool)
                    n797 = Less?(x=w1676, y=i16 5) -> ()  [unwired: 1 out]
                    n798 = Not(x=w1675) -> (.not. x?=w1668:bool)
                    n799 = local write "Robot Mode:"(w1681) -> ()
                    n800 = shared-variable ".\\Operator Variables.lvlib\\Mode"(w1681) -> ()  [unwired: 1 in, 1 out]
                    n801 = And(x=w1665, y=w1668) -> (x .and. y?=w1664:bool)
                    n802 = Select(t=TRUE, s=w1664, f=FALSE) -> (s? t:f=w1671:bool)
                    n803 = local write "Block Find"(w1671) -> ()
                    n804 = Select(t=98, s=w1664, f=0) -> (s? t:f=w1672:i32)
                  }
                }
              }
              frame 98 {
                # "20"
                n805 = local read "Proc Finish"() -> (w1686:bool)
                n806 = Greater?(x=w1682, y=5.0) -> (0:w1683:bool)
                n807 = And(x=w1686, y=w1683) -> (x .and. y?=w1685:bool)
                n808 = case shown="True" w1685 {
                  tunnel: w1687 -> [w1690 _]
                  tunnel: [w1690 100] -> w1688
                  frame False {
                  }
                  frame True {
                    w1693 = Operator_Loop_Mode."Idle" ("Operator Loop Mode")
                    n809 = local write "Block Find"(FALSE ("Block Find")) -> ()
                    n810 = local write "Robot Mode:"(w1693) -> ()
                    n811 = shared-variable ".\\Operator Variables.lvlib\\Mode"(w1693) -> ()  [unwired: 1 in, 1 out]
                  }
                }
              }
              frame 100 {
                n812 = local read "Proc Finish"() -> (w1702:bool)
                n813 = Greater?(x=w1699, y=10.0) -> (0:w1700:bool)
                n814 = And(x=w1702, y=w1700) -> (x .and. y?=w1698:bool)
                n815 = case shown="True" w1698 {
                  tunnel: w1697 -> [w1704 w1706]
                  tunnel: [w1704 w1706] -> w1696
                  tunnel: w1695 -> [w1703 _]
                  tunnel: [w1703 0 ("f")] -> w1694
                  frame False {
                  }
                  frame True {
                  }
                }
              }
            }
          }
          frame 100 {
            # "ず"
            # "外"
            # "ず"
            # "外"
            # "進出發區處裡"
            n816 = case shown="20" w1711 {
              tunnel: w1711 -> [_ _ w1731 w1742 w1753 w1766 w1777 w1789 w1800 w1805]
              tunnel: w1710 -> [w1719 w1721 w1729 w1740 w1751 w1764 w1775 w1787 w1798 _]
              tunnel: [w1719 w1721 w1729 w1740 w1751 w1764 w1775 w1787 w1798 0] -> w1709
              tunnel: [5 10 w1730 w1741 w1752 w1765 w1776 w1788 w1799 w1805] -> w1708
              tunnel: w1707 -> [_ _ w1726 w1735 w1746 w1759 w1770 w1782 w1793 _]
              frame 0, Default {
                # "設定出發區前方為目標"
                n817 = local read "Start Front"() -> (w1712:dbl[])
                n818 = local read "Start POS"() -> (w1718:dbl[])
                n819 = Index Array(array=w1712) -> (element #1=w1716:dbl, element #2=w1715:dbl)  [unwired: 2 in]
                n820 = Index Array(array=w1718, index=2) -> (element=w1714:dbl)
                n821 = Build Array(w1716, w1715, w1714) -> (w1713:dbl[])
                n822 = shared-variable ".\\Operator Variables.lvlib\\SubGoal"(w1713) -> ()  [unwired: 1 in, 1 out]
              }
              frame 5 {
                w1722 = Operator_Loop_Mode."Path Following" ("Operator Loop Mode")
                # "避障行走"
                n823 = local write "Robot Mode:"(w1722) -> ()
                n824 = shared-variable ".\\Operator Variables.lvlib\\Mode"(w1722) -> ()  [unwired: 1 in, 1 out]
              }
              frame 10 {
                n825 = local read "Proc Finish"() -> (w1725:bool)
                n826 = Greater?(x=w1726, y=5) -> (0:w1727:bool)
                n827 = And(x=w1725, y=w1727) -> (x .and. y?=w1724:bool)
                n828 = case shown="True" w1724 {
                  tunnel: w1731 -> [w1732 _]
                  tunnel: [w1732 20] -> w1730
                  frame False {
                  }
                  frame True {
                    w1733 = Operator_Loop_Mode."Go Target" ("Operator Loop Mode")
                    # "設定執行Go Target"
                    n829 = local write "Robot Mode:"(w1733) -> ()
                    n830 = shared-variable ".\\Operator Variables.lvlib\\Mode"(w1733) -> ()  [unwired: 1 in, 1 out]
                  }
                }
              }
              frame 20 {
                n831 = local read "Proc Finish"() -> (w1737:bool)
                n832 = Greater?(x=w1735, y=5) -> (0:w1738:bool)
                n833 = And(x=w1737, y=w1738) -> (x .and. y?=w1736:bool)
                n834 = case shown="True" w1736 {
                  tunnel: w1742 -> [w1743 _]
                  tunnel: [w1743 25] -> w1741
                  frame False {
                  }
                  frame True {
                    w1744 = Operator_Loop_Mode."Home Correction" ("Operator Loop Mode")
                    # "正式程式要執行Home Correction"
                    n835 = local write "Robot Mode:"(w1744) -> ()
                    n836 = shared-variable ".\\Operator Variables.lvlib\\Mode"(w1744) -> ()  [unwired: 1 in, 1 out]
                  }
                }
              }
              frame 25 {
                n837 = local read "Proc Finish"() -> (w1748:bool)
                n838 = Greater?(x=w1746, y=5) -> (0:w1749:bool)
                n839 = And(x=w1748, y=w1749) -> (x .and. y?=w1747:bool)
                n840 = case shown="True" w1747 {
                  tunnel: w1753 -> [w1754 _]
                  tunnel: [w1754 30] -> w1752
                  frame False {
                  }
                  frame True {
                    w1757 = Operator_Loop_Mode."Idle" ("Operator Loop Mode")
                    n841 = shared-variable ".\\Operator Variables.lvlib\\SubGoal"() -> (w1756:dbl[])  [unwired: 1 in, 1 out]
                    n842 = local write "Block Fix array"(w1756) -> ()
                    n843 = local write "Robot Mode:"(w1757) -> ()
                    n844 = shared-variable ".\\Operator Variables.lvlib\\Mode"(w1757) -> ()  [unwired: 1 in, 1 out]
                    n845 = local write "Enable ND"(FALSE ("Enable ND")) -> ()
                  }
                }
              }
              frame 27 {
                n846 = local read "Proc Finish"() -> (w1761:bool)
                n847 = Greater?(x=w1759, y=3) -> (0:w1762:bool)
                n848 = And(x=w1761, y=w1762) -> (x .and. y?=w1760:bool)
                n849 = case shown="True" w1760 {
                  tunnel: w1766 -> [w1767 _]
                  tunnel: [w1767 30] -> w1765
                  frame False {
                  }
                  frame True {
                    w1768 = Operator_Loop_Mode."hands down" ("Operator Loop Mode")
                    n850 = local write "Robot Mode:"(w1768) -> ()
                    n851 = shared-variable ".\\Operator Variables.lvlib\\Mode"(w1768) -> ()  [unwired: 1 in, 1 out]
                  }
                }
              }
              frame 30 {
                n852 = local read "Proc Finish"() -> (w1772:bool)
                n853 = Greater?(x=w1770, y=5) -> (0:w1773:bool)
                n854 = And(x=w1772, y=w1773) -> (x .and. y?=w1771:bool)
                n855 = case shown="True" w1771 {
                  tunnel: w1777 -> [w1778 _]
                  tunnel: [w1778 40] -> w1776
                  frame False {
                  }
                  frame True {
                    w1779 = Operator_Loop_Mode."Idle" ("Operator Loop Mode")
                    # "校正XYZ,並設定出發區為目標"
                    n856 = local read "Start POS"() -> (w1780:dbl[])
                    n857 = local write "Robot Mode:"(w1779) -> ()
                    n858 = shared-variable ".\\Operator Variables.lvlib\\Mode"(w1779) -> ()  [unwired: 1 in, 1 out]
                    n859 = shared-variable ".\\Operator Variables.lvlib\\SubGoal"(w1780) -> ()  [unwired: 1 in, 1 out]
                  }
                }
              }
              frame 40 {
                n860 = local read "Proc Finish"() -> (w1784:bool)
                n861 = Greater?(x=w1782, y=3) -> (0:w1785:bool)
                n862 = And(x=w1784, y=w1785) -> (x .and. y?=w1783:bool)
                n863 = case shown="True" w1783 {
                  tunnel: w1789 -> [w1790 _]
                  tunnel: [w1790 45] -> w1788
                  frame False {
                  }
                  frame True {
                    w1791 = Operator_Loop_Mode."Go Target" ("Operator Loop Mode")
                    # "正式程式要執行回到出發區"
                    n864 = local write "Robot Mode:"(w1791) -> ()
                    n865 = shared-variable ".\\Operator Variables.lvlib\\Mode"(w1791) -> ()  [unwired: 1 in, 1 out]
                  }
                }
              }
              frame 45 {
                n866 = local read "Proc Finish"() -> (w1795:bool)
                n867 = Greater?(x=w1793, y=5) -> (0:w1796:bool)
                n868 = And(x=w1795, y=w1796) -> (x .and. y?=w1794:bool)
                n869 = case shown="True" w1794 {
                  tunnel: w1800 -> [w1801 _]
                  tunnel: [w1801 50] -> w1799
                  frame False {
                  }
                  frame True {
                    w1802 = Operator_Loop_Mode."Idle" ("Operator Loop Mode")
                    # "完成"
                    n870 = local write "Robot Mode:"(w1802) -> ()
                    n871 = shared-variable ".\\Operator Variables.lvlib\\Mode"(w1802) -> ()  [unwired: 1 in, 1 out]
                  }
                }
              }
              frame 50 {
              }
            }
          }
        }
        n872 = Less?(x=w674, y=500) -> (x < y?=w686:bool)
        n873 = Increment(x=w674) -> (x+1=w685:i32)
        n874 = Select(t=w685, s=w686, f=w674) -> (s? t:f=w687:i32)
        n875 = Not Equal?(x=w675, y=w671) -> (x != y?=w678:bool)
        n876 = local read "stop"() -> (w673:bool)
        n877 = node-c288() -> ()  [unwired: 1 in, 1 out]
        n878 = Select(t=0, s=w678, f=w676) -> (s? t:f=w677:i32)
        n879 = Not Equal?(x=w677, y=w670) -> (x != y?=w683:bool)
        n880 = Or(x=w678, y=w683) -> (x .or. y?=w682:bool)
        n881 = Select(t=0, s=w682, f=w687) -> (s? t:f=w680:i32)
      }
      n882 = timed-loop {
        timing: w486 -> [_]
        timing-out: [_] -> w485
        stop <- w1813 stop-if-true
        # "利用邊牆計算座標位置與偏移角度"
        n883 = node-c288() -> ()  [unwired: 1 in, 1 out]
        n884 = case shown="True" "Block Find" {
          frame False {
          }
          frame True {
            # "在出發區沒有數值的狀況下表示尚未定位,不可修正"
            # "將位置計算中心由車子改為0,0點"
            n885 = shared-variable ".\\LIDAR Data Variables.lvlib\\LIDAR Data"() -> (w1843:dbl[])  [unwired: 1 in, 1 out]
            n886 = call "Unflatten LIDAR Data.vi"("Flat LIDAR Data"=w1843) -> ("Robot Pose x,y (m)"=w1834:dbl[], "Robot Pose Theta (rad)"=w1833:dbl, "Bearing (rad)"=w1829:dbl[], "Range (m)"=w1835:dbl[])  [unwired: 7 in]
            n887 = Build Array (concatenate)(w1834, w1833) -> (w1832:dbl[])
            n888 = expression code="(x/pi)*180.0" "radians to degrees"(w1829) -> (w1838:dbl[])
            n889 = Build Array(0.0 ("element"), 0.0 ("element"), 0.0 ("element")) -> (w1837:dbl[])
            n890 = local read "Start POS"() -> (w1826:dbl[])
            n891 = Index Array(array=w1826) -> (element #1=w1825:dbl, element #2=w1824:dbl)  [unwired: 2 in]
            n892 = Multiply(x=w1835, y=1000.0) -> (x*y=w1830:dbl[])
            n893 = Not Equal To 0?(x=w1825) -> (x != 0?=w1827:bool)
            n894 = Not Equal To 0?(x=w1824) -> (x != 0?=w1828:bool)
            n895 = call "Transform LIDAR Data.vi"("New Orientation (X m, Y m, T rad)"=w1837, "Orientation (X m, Y m, T rad)"=w1832, "Direction (deg)"=w1838, "Magnitude (mm)"=w1830) -> ("Direction out (rad)"=w1815:dbl[], "Magnitude out (m)"=w1831:dbl[])  [unwired: 5 in, 1 out]
            n896 = And(x=w1827, y=w1828) -> (x .and. y?=w1814:bool)
            n897 = Negate(x=w1815) -> (-x=w1816:dbl[])
            n898 = Multiply(x=w1831, y=1000.0) -> (x*y=w1839:dbl[])
            n899 = local read "Start Front"() -> (w1822:dbl[])
            n900 = local read "Start POS"() -> (w1823:dbl[])
            n901 = Polar To Re/Im(2:w1816, 3:w1839) -> (0:w1818:dbl[], 1:w1819:dbl[])
            n902 = call "Global MAP.vi"("Start point"=w1823, "Start Front point"=w1822, "Y point"=w1818, "X point"=w1819) -> ("ODM Global Lidar"=w1821:cluster{dbl[], dbl[]}[])  [unwired: 7 in]
            n903 = case shown="True" w1814 {
              tunnel: w1819 -> [_ w1856]
              tunnel: w1818 -> [_ w1855]
              tunnel: w1821 -> [w1844 w1846]
              tunnel: [w1844 w1845] -> w1820
              frame False {
              }
              frame True {
                w1848 = 1000.0 ("y")
                # "找方塊功能"
                n904 = local read "Start POS"() -> (w1849:dbl[])
                n905 = local read "Block Array"() -> (w1853:dbl[][])
                n906 = shared-variable ".\\Motor Control Variables.lvlib\\Odometry Data"() -> (w1859:dbl[])  [unwired: 1 in, 1 out]
                n907 = Multiply(x=w1849, y=w1848) -> (x*y=w1847:dbl[])
                n908 = call "LIDAR Position from Inertial Position.vi"("CM X, Y, Theta"=w1859) -> ("LIDAR X, Y, Theta"=w1858:dbl[])  [unwired: 10 in]
                n909 = Multiply(x=w1858, y=w1848) -> (x*y=w1857:dbl[])
                n910 = call "FindBlock.vi"("Start pos"=w1847, "Block Array in"=w1853, "Robot pos"=w1857, "World Y array"=w1855, "World X array"=w1856) -> ("ODM Global Lidar Fix Map"=w1852:cluster{dbl[], dbl[]}[], "Block Array out"=w1854:dbl[][])  [unwired: 4 in, 1 out]
                n911 = local write "Block Array"(w1854) -> ()
                n912 = Index Array(array=w1852) -> (element #1=w1851:cluster{dbl[], dbl[]}, element #2=w1850:cluster{dbl[], dbl[]})  [unwired: 2 in]
                n913 = Build Array (concatenate)(w1846, w1851, w1850) -> (w1845:cluster{dbl[], dbl[]}[])
              }
            }
            "ODM Global Lidar" <- w1820
          }
        }
        n914 = local read "stop"() -> (w1813:bool)
        n915 = node-c288() -> ()  [unwired: 1 in, 1 out]
      }
      n916 = while {
        tunnel: w451 -> [w2505]
        tunnel: w452 -> [w2507]
        tunnel: [w2506] -> w470
        tunnel: w487 -> [w2497]
        tunnel: [w2498] -> w482
        stop <- w2500 stop-if-true
        # "假造一個光點在出發出的出口\n防止機器跑進去出發區(機器距離50cm內才做"
        # "光達讀取"
        n917 = shared-variable ".\\Motor Control Variables.lvlib\\Odometry Data"() -> (w2493:dbl[])  [unwired: 1 in, 1 out]
        n918 = local read "Start Out Point"() -> (w2492:dbl[])
        n919 = call "URG-04LX-UG01 Read Measurement Data.vi"("Acquisition Parameters"=w2505, "VISA Refnum in"=w2507) -> ("error out"=w2498:errorcluster, "Distance Measurements"=w2504:i32[], "VISA Refnum out"=w2506:refnum<visa-resource-name>)  [unwired: 6 in, 1 out]
        n920 = for {
          tunnel: w2504 -> [w2530] mode=indexing
          tunnel: w2497 -> [w2531] mode=indexing
          shift-right: [w2542] -> w2462
          shift-left: i32[] [] -> [w2544]
          shift-right: [w2541] -> w2494
          shift-left: dbl[] [] -> [w2543]
          shift-right: [w2537] -> w2464
          shift-left: 9999 -> [w2538]
          # "最小最大範圍處理"
          n921 = In Range and Coerce(upper limit=20.0, x=w2531, lower limit=-20.0 ("upper limit")) -> (In Range?=w2536:bool)  [unwired: 1 out]
          n922 = Less?(x=w2530, y=w2538) -> (x < y?=w2532:bool)
          n923 = Greater?(x=w2530, y=3300) -> (0:w2546:bool)
          n924 = Less Or Equal?(x=w2530, y=50) -> (x <= y?=w2545:bool)
          n925 = And(x=w2536, y=w2532) -> (x .and. y?=w2535:bool)
          n926 = Or(x=w2546, y=w2545) -> (x .or. y?=w2533:bool)
          n927 = Not(x=w2533) -> (.not. x?=w2529:bool)
          n928 = And(x=w2529, y=w2535) -> (x .and. y?=w2534:bool)
          n929 = Select(t=w2530, s=w2534, f=w2538) -> (s? t:f=w2537:i32)
          n930 = case shown="False" w2533 {
            tunnel: w2544 -> [w2554 w2556]
            tunnel: w2543 -> [w2553 w2555]
            tunnel: [w2552 w2556] -> w2542
            tunnel: [w2551 w2555] -> w2541
            tunnel: w2530 -> [w2550 _]
            tunnel: w2531 -> [w2549 _]
            frame False {
              n931 = Insert Into Array(array=w2553, new element=w2549) -> (w2551:dbl[])  [unwired: 1 in]
              n932 = Insert Into Array(array=w2554, new element=w2550) -> (w2552:i32[])  [unwired: 1 in]
            }
            frame True {
            }
          }
        }
        n933 = Index Array(array=w2493) -> (element #1=w2490:dbl, element #2=w2488:dbl, element #3=w2482:dbl)  [unwired: 3 in]
        n934 = Index Array(array=w2492) -> (element #1=w2491:dbl, element #2=w2489:dbl)  [unwired: 2 in]
        n935 = local read "stop"() -> (w2499:bool)
        n936 = Subtract(x=w2491, y=w2490) -> (x-y=w2487:dbl)
        n937 = Subtract(x=w2489, y=w2488) -> (x-y=w2486:dbl)
        n938 = call "LIDAR Position from Inertial Position.vi"("CM X, Y, Theta"=w2493) -> ("LIDAR X, Y, Theta"=w2503:dbl[])  [unwired: 10 in]
        n939 = Re/Im To Polar(2:w2486, 3:w2487) -> (0:w2485:dbl, 1:w2466:dbl)
        n940 = Subtract(x=w2485, y=1.5707963267948966) -> (x-y=w2483:dbl)
        n941 = Or(x=w2498, y=w2499) -> (x .or. y?=w2500:bool)
        n942 = Array Size(array=w2462) -> (size(s)=w2460:i32)
        n943 = call "Transform LIDAR Data.vi"("New Orientation (X m, Y m, T rad)"=w2493, "Orientation (X m, Y m, T rad)"=w2503, "Direction (deg)"=w2494, "Magnitude (mm)"=w2462) -> ("New Orientation (X m, Y m, T rad) out"=w2468:dbl[], "Direction out (rad)"=w2470:dbl[], "Magnitude out (m)"=w2472:dbl[])  [unwired: 5 in]
        n944 = Subtract(x=w2483, y=w2482) -> (x-y=w2481:dbl)
        n945 = Less?(x=w2466, y=0.5) -> (x < y?=w2473:bool)
        n946 = Divide(x=w2460, y=2) -> (x/y=w2458:dbl)
        n947 = Quotient & Remainder(x=w2481, y=6.283185307179586) -> (x-y*floor(x/y)=w2474:dbl)  [unwired: 1 out]
        n948 = Index Array(array=w2462, index=w2458) -> (element=w2461:i32)
        n949 = shared-variable ".\\Operator Variables.lvlib\\NearDistance"(w2464) -> ()  [unwired: 1 in, 1 out]
        n950 = Greater?(x=w2474, y=3.141592653589793) -> (0:w2477:bool)
        n951 = local write "Lidar mid"(w2461) -> ()
        n952 = Subtract(x=w2474, y=6.283185307179586) -> (x-y=w2475:dbl)
        n953 = Select(t=w2475, s=w2477, f=w2474) -> (s? t:f=w2465:dbl)
        n954 = case shown="True" "Show Lidar" {
          tunnel: w2494 -> [_ w2520]
          tunnel: w2462 -> [_ w2519]
          frame False {
          }
          frame True {
            w2526 = 0.0 ("element")
            # "是否顯示光達值與光達圖"
            n955 = Negate(x=w2520) -> (-x=w2521:dbl[])
            n956 = expression code="(x/180.0)*pi" "degrees to radians"(w2521) -> (w2522:dbl[])
            n957 = Polar To Re/Im(2:w2522, 3:w2519) -> (0:w2527:dbl[], 1:w2528:dbl[])
            n958 = Build Array (concatenate)(w2526, w2528, w2526) -> (w2523:dbl[])
            n959 = Build Array (concatenate)(w2526, w2527, w2526) -> (w2524:dbl[])
            n960 = Bundle(w2524, w2523) -> (→"Lidar Data":cluster{dbl[], dbl[]})  [unwired: 1 in]
            "Distance" <- w2519
          }
        }
        n961 = case shown="True" w2473 {
          tunnel: w2472 -> [w2510 w2517]
          tunnel: [w2510 w2516] -> w2471
          tunnel: w2470 -> [w2509 w2515]
          tunnel: [w2509 w2511] -> w2469
          tunnel: w2468 -> [w2508 w2518]
          tunnel: [w2508 w2518] -> w2467
          tunnel: w2466 -> [_ w2513]
          tunnel: w2465 -> [_ w2512]
          frame False {
          }
          frame True {
            n962 = Array Size(array=w2517) -> (size(s)=w2514:i32)
            n963 = Insert Into Array(array=w2517, index=w2514, new element=w2513) -> (w2516:dbl[])
            n964 = Insert Into Array(array=w2515, index=w2514, new element=w2512) -> (w2511:dbl[])
          }
        }
        n965 = Build Array (concatenate)(w2471, w2469, w2467) -> (w2502:dbl[])
        n966 = shared-variable ".\\LIDAR Data Variables.lvlib\\LIDAR Data"(w2502) -> ()  [unwired: 1 in, 1 out]
      }
      n967 = node-c288(i64 100 ("Period")) -> (w491:T20)  [unwired: 3 in]
      n968 = timed-loop {
        timing: w491 -> [_]
        timing-out: [_] -> w490
        tunnel: 0.16 ("obstacle clearance (m)") -> [w1929]
        shift-right: [w1922] -> _
        shift-left: w488 -> [w1924]
        tunnel: w463 -> [w1926]
        tunnel: w460 -> [w1917]
        tunnel: w459 -> [w1916]
        tunnel: w456 -> [w1915]
        stop <- w1928 stop-if-true
        # "行走處理"
        n969 = node-c288() -> ()  [unwired: 1 in, 1 out]
        n970 = shared-variable ".\\Operator Variables.lvlib\\Mode"() -> (w1923:T19)  [unwired: 1 in, 1 out]
        n971 = Not Equal?(x=w1923, y=w1924) -> (x != y?=w1914:bool)
        n972 = Select(t=w1923, s=w1914, f=w1924) -> (s? t:f=w1922:T19)
        n973 = case shown="\"moveblock\"" w1923 {
          tunnel: w1914 -> [_ _ w2005 _ _ _ _ _ _ _ _ w2310 w2373 _ _ _]
          tunnel: w1929 -> [_ _ w2008 _ _ _ _ _ _ _ _ _ _ _ _ _]
          tunnel: [0.0 ("command vx") w1992 w2015 w2050 0.0 ("command vx") w2070 w2109 0.0 ("command vx") 0.0 ("command vx") 0.0 ("command vx") 0.0 ("command vx") w2291 w2349 _ _ 0.0 ("command vx")] -> w1919
          tunnel: [0.0 ("command vy") w1990 w2009 w2049 0.0 ("command vy") w2059 w2108 0.0 ("command vy") 0.0 ("command vy") 0.0 ("command vy") 0.0 ("command vy") w2331 w2392 _ _ 0.0 ("command vy")] -> w1920
          tunnel: [w1933 w1991 w2013 w2043 w2053 w2073 w2102 w2196 w2227 w2274 w2287 w2295 w2358 _ _ w2439] -> w1921
          tunnel: w1926 -> [_ _ _ _ _ _ _ _ _ _ w2284 _ _ w2408 w2425 _]
          tunnel: [TRUE TRUE w2010 w2035 TRUE w2067 w2107 w2141 w2224 TRUE TRUE w2320 w2355 TRUE TRUE FALSE] -> w1918
          tunnel: w1917 -> [_ _ _ _ _ _ _ _ w2223 _ _ _ _ _ _ w2438]
          tunnel: w1916 -> [_ _ _ _ _ _ _ _ w2222 _ _ _ _ _ _ w2436]
          tunnel: w1915 -> [_ _ _ _ _ _ _ _ w2221 _ _ _ _ _ _ w2437]
          frame "Idle", Default {
            (unwired) 0
            # "甚麼都不做"
            n974 = case shown="True" "Set Start POS" {
              frame False {
              }
              frame True {
                w1981 = 1000
                # "計算出發區的X,Y"
                # "進出發區的角度剛好是相反的"
                n975 = local read "Angle Find"() -> (w1950:dbl)
                n976 = local read "FY"() -> (w1983:dbl)
                n977 = local read "FX"() -> (w1982:dbl)
                n978 = local read "Start Front"() -> (w1970:dbl[])
                n979 = local read "Start Out Point"() -> (w1975:dbl[])
                n980 = Add(x=w1950, y=3.141592653589793) -> (x+y=w1967:dbl)
                n981 = Quotient & Remainder(x=w1967, y=6.283185307179586) -> (x-y*floor(x/y)=w1966:dbl)  [unwired: 1 out]
                n982 = Negate(x=w1950) -> (-x=w1949:dbl)
                n983 = Negate(x=w1950) -> (-x=w1951:dbl)
                n984 = Index Array(array=w1970) -> (element #1=w1955:dbl, element #2=w1956:dbl)  [unwired: 2 in]
                n985 = Greater Or Equal?(x=w1966, y=3.141592653589793) -> (x >= y?=w1964:bool)
                n986 = Index Array(array=w1975) -> (element #1=w1974:dbl, element #2=w1973:dbl)  [unwired: 2 in]
                n987 = Divide(x=w1982, y=w1981) -> (x/y=w1954:dbl)
                n988 = Divide(x=w1983, y=w1981) -> (x/y=w1953:dbl)
                n989 = Subtract(x=w1966, y=6.283185307179586) -> (x-y=w1962:dbl)
                n990 = call-poly <vilib>:"2D Cartesian Coordinate Rotation.vi"("theta"=w1949, "y"=w1956, "x"=w1955) -> ("y out"=w1958:dbl, "x out"=w1957:dbl)  [unwired: 6 in, 1 out]
                n991 = call-poly <vilib>:"2D Cartesian Coordinate Rotation.vi"("theta"=w1951, "y"=w1973, "x"=w1974) -> ("y out"=w1977:dbl, "x out"=w1976:dbl)  [unwired: 6 in, 1 out]
                n992 = Select(t=w1962, s=w1964, f=w1966) -> (s? t:f=w1971:dbl)
                n993 = Subtract(x=w1953, y=w1977) -> (x-y=w1979:dbl)
                n994 = Subtract(x=w1953, y=w1958) -> (x-y=w1960:dbl)
                n995 = Subtract(x=w1954, y=w1976) -> (x-y=w1978:dbl)
                n996 = Subtract(x=w1954, y=w1957) -> (x-y=w1959:dbl)
                n997 = Build Array(w1954, w1953, w1971) -> (w1972:dbl[])
                n998 = Build Array(w1954, w1953, w1950) -> (w1952:dbl[])
                n999 = Build Array(w1978, w1979) -> (w1980:dbl[])
                n1000 = Build Array(w1959, w1960, w1971) -> (w1969:dbl[])
                n1001 = local write "Start POS"(w1969) -> ()
                n1002 = local write "Start Front"(w1972) -> ()
                n1003 = local write "Start Out Point"(w1980) -> ()
                n1004 = local write "Block Fix array"(w1952) -> ()
              }
            }
            n1005 = case shown="True" "Reset Start POS" {
              frame False {
              }
              frame True {
                w1948 = 0.0
                n1006 = Build Array(w1948, 0.345 ("element"), 0.0 ("element")) -> (w1942:dbl[])
                n1007 = Build Array(w1948, w1948, w1948) -> (w1943:dbl[])
                n1008 = Build Array(0.0 ("element"), 0.1725 ("element")) -> (w1941:dbl[])
                n1009 = local write "Start POS"(w1943) -> ()
                n1010 = local write "Start Front"(w1942) -> ()
                n1011 = local write "Start Out Point"(w1941) -> ()
              }
            }
            n1012 = case shown="True" "Set SubGoal" {
              frame False {
              }
              frame True {
                n1013 = shared-variable ".\\Motor Control Variables.lvlib\\Odometry Data"() -> (w1984:dbl[])  [unwired: 1 in, 1 out]
                n1014 = shared-variable ".\\Operator Variables.lvlib\\SubGoal"(w1984) -> ()  [unwired: 1 in, 1 out]
              }
            }
            n1015 = shared-variable ".\\Motor Control Variables.lvlib\\Odometry Data"() -> (w1934:dbl[])  [unwired: 1 in, 1 out]
            n1016 = Index Array(array=w1934) -> (element #3=w1933:dbl)  [unwired: 3 in, 2 out]
          }
          frame "Tele-Op" {
            # "使用介面控制移動"
            # "使用介面控制移動"
            n1017 = local read "Heading(rad)"() -> (w1991:dbl)
            n1018 = local read "X Velocity (m/s)"() -> (w2000:dbl)
            n1019 = local read "Y Velocity (m/s)"() -> (w1999:dbl)
            n1020 = Select(t=0.2, s="+X", f=w2000) -> (s? t:f=w1996:dbl)
            n1021 = Select(t=0.2, s="+Y", f=w1999) -> (s? t:f=w1995:dbl)
            n1022 = Select(t=-0.2, s="-X", f=w1996) -> (s? t:f=w1992:dbl)
            n1023 = Select(t=-0.2, s="-Y", f=w1995) -> (s? t:f=w1990:dbl)
          }
          frame "Path Following" {
            # "以指定SubGoal為目標避障行走"
            n1024 = case shown="False" w2005 {
              tunnel: [w2029 9999.0 ("min Distance")] -> w2002
              frame False {
                n1025 = local read "min Distance"() -> (w2029:dbl)
              }
              frame True {
                # "剛切到此模式時\n將距離設到很大"
              }
            }
            n1026 = shared-variable ".\\LIDAR Data Variables.lvlib\\LIDAR Data"() -> (w2028:dbl[])  [unwired: 1 in, 1 out]
            n1027 = shared-variable ".\\Operator Variables.lvlib\\SubGoal"() -> (w2027:dbl[])  [unwired: 1 in, 1 out]
            n1028 = call "Unflatten LIDAR Data.vi"("Flat LIDAR Data"=w2028) -> ("Robot Pose x,y (m)"=w2026:dbl[], "Robot Pose Theta (rad)"=w2019:dbl, "Bearing (rad)"=w2020:dbl[], "Range (m)"=w2021:dbl[])  [unwired: 7 in]
            n1029 = call "Find Relative Goal Location.vi"("Goal Position"=w2027, "Current Position"=w2026) -> ("Target Distance"=w2003:dbl, "Target Heading"=w2018:dbl)  [unwired: 8 in]
            "Target Distance" <- w2003
            n1030 = Multiply(x=w2008, y="inner threshold") -> (x*y=w2023:dbl)
            n1031 = Multiply(x=w2008, y="outer threshold") -> (x*y=w2022:dbl)
            n1032 = Bundle(w2023, w2022) -> (w2017:cluster{dbl, dbl})  [unwired: 1 in]
            n1033 = call "Call Vector Field Histogram.vi"("LIDAR magn. (m)"=w2021, "max speed"="max speed", "Initialize?"=w2005, "LIDAR angle (rad)"=w2020, "current heading (rad)"=w2019, "target heading (rad)"=w2018, "target distance"=w2003, "obstacle clearance (m)"=w2008, "thresholds"=w2017) -> ("command vx"=w2015:dbl, "command vy"=w2009:dbl, "command heading (rad)"=w2013:dbl, "histogram out"=w2014:dbl[], "mask out"=w2012:bool[])  [unwired: 2 in]
            n1034 = shared-variable ".\\Operator Variables.lvlib\\Outer Threshold"(w2022) -> ()  [unwired: 1 in, 1 out]
            n1035 = shared-variable ".\\Operator Variables.lvlib\\Inner Threshold"(w2023) -> ()  [unwired: 1 in, 1 out]
            n1036 = shared-variable ".\\Operator Variables.lvlib\\Histogram"(w2014) -> ()  [unwired: 1 in, 1 out]
            n1037 = shared-variable ".\\Operator Variables.lvlib\\Mask"(w2012) -> ()  [unwired: 1 in, 1 out]
            n1038 = Add(x=w2008, y=0.02) -> (x+y=w2006:dbl)
            n1039 = Subtract(x=w2008, y=0.03) -> ()  [unwired: 1 out]
            n1040 = Less?(x=w2003, y=w2002) -> (x < y?=w2004:bool)
            n1041 = Less Or Equal?(x=w2003, y=w2006) -> (x <= y?=w2010:bool)
            n1042 = Select(t=w2003, s=w2004, f=w2002) -> (s? t:f=→"min Distance":dbl)
          }
          frame "Go Target" {
            w2046 = FALSE
            # "座標對準並,面對指定的方向"
            n1043 = shared-variable ".\\Motor Control Variables.lvlib\\Odometry Data"() -> (w2042:dbl[])  [unwired: 1 in, 1 out]
            n1044 = local write "Left Block"(w2046) -> ()
            n1045 = local write "Right Block"(w2046) -> ()
            n1046 = shared-variable ".\\Operator Variables.lvlib\\SubGoal"() -> (w2033:dbl[])  [unwired: 1 in, 1 out]
            n1047 = Multiply(x=0.4, y=1.0) -> (x*y=w2047:dbl)
            n1048 = call "GoTarget.vi"("Enable ND"="Enable ND", "max speed"=w2047, "Distance"=0.02 ("y"), "SubGoal"=w2033, "Odometry Data"=w2042) -> ("Target Distance"=w2044:dbl, "Head CMD"=w2043:dbl, "VY"=w2049:dbl, "VX"=w2050:dbl)  [unwired: 3 in]
            n1049 = Less Or Equal?(x=w2044, y=0.03) -> (x <= y?=w2036:bool)
            n1050 = Index Array(array=w2042) -> (element #3=w2041:dbl)  [unwired: 3 in, 2 out]
            n1051 = Subtract(x=w2043, y=w2041) -> (x-y=w2040:dbl)
            n1052 = expression code="(x/pi)*180.0" "radians to degrees"(w2040) -> (w2039:dbl)
            n1053 = Absolute Value(x=w2039) -> (abs(x)=w2038:dbl)
            n1054 = Less?(x=w2038, y=15.0) -> (x < y?=w2034:bool)
            n1055 = And(x=w2036, y=w2034) -> (x .and. y?=w2035:bool)
          }
          frame "Wall Correction" {
            # "牆面對正,尚未處理"
            n1056 = shared-variable ".\\Motor Control Variables.lvlib\\Odometry Data"() -> (w2057:dbl[])  [unwired: 1 in, 1 out]
            n1057 = Index Array(array=w2057, index=2) -> (element=w2053:dbl)
          }
          frame "Block Correction" {
            (unwired) 5
            # "H"
            # "Y"
            # "X"
            # "5mm"
            # "3度"
            # "10mm"
            n1058 = local read "UltraSound"() -> (w2058:dbl)
            n1059 = call "Block Correction.vi"() -> ("RL Dist"=w2072:dbl, "Block rad"=w2078:dbl, "Block Face"=w2066:dbl, "Close Range"=w2062:dbl, "Right Block"=w2076:bool, "Left Block"=w2077:bool)  [unwired: 6 in]
            "LD Range" <- w2062
            n1060 = local write "Left Block"(w2077) -> ()
            n1061 = local write "Right Block"(w2076) -> ()
            n1062 = Select(t=w2058, s="Enable US", f=w2062) -> (s? t:f=w2060:dbl)
            n1063 = Subtract(x="BL Range", y=w2060) -> (x-y=w2081:dbl)
            n1064 = Absolute Value(x=w2081) -> (abs(x)=w2080:dbl)
            n1065 = shared-variable ".\\Motor Control Variables.lvlib\\Odometry Data"() -> (w2092:dbl[])  [unwired: 1 in, 1 out]
            n1066 = local read "QR_CAM"() -> (w2065:bool)
            n1067 = call-poly <vilib>:"PID.vi"("output range"=cluster{"output high":dbl, "output low":dbl} {"output high"=100.0, "output low"=-100.0}, "PID gains"=T6 {"proportional gain (Kc)"=0.25, "integral time (Ti, min)"=0.0, "derivative time (Td, min)"=0.0}, "process variable"=w2060, "setpoint"="BL Range") -> ("output"=w2098:dbl)  [unwired: 6 in, 1 out]
            n1068 = Divide(x=w2098, y=-100.0) -> (x/y=w2059:dbl)
            n1069 = Add(x=w2078, y=1.5707963267948966) -> (x+y=w2079:dbl)
            n1070 = call-poly <vilib>:"PID.vi"("output range"=cluster{"output high":dbl, "output low":dbl} {"output high"=100.0, "output low"=-100.0}, "PID gains"=T6 {"proportional gain (Kc)"=0.2, "integral time (Ti, min)"=0.0, "derivative time (Td, min)"=0.0001}, "process variable"=w2072, "setpoint"=0.0 ("y")) -> ("output"=w2071:dbl)  [unwired: 6 in, 1 out]
            n1071 = Divide(x=w2071, y=-100.0) -> (x/y=w2070:dbl)
            n1072 = Select(t=0.0, s=w2065, f=w2066) -> (s? t:f=→"Block Face":dbl)
            n1073 = Index Array(array=w2092, index=2) -> (element=w2074:dbl)
            n1074 = expression code="(x/pi)*180.0" "radians to degrees"(w2079) -> (w2083:dbl)
            n1075 = Multiply(x=w2079, y=1.0) -> (x*y=w2075:dbl)
            n1076 = Add(x=w2075, y=w2074) -> (x+y=w2073:dbl)
            n1077 = Subtract(x=w2074, y=w2078) -> ()  [unwired: 1 out]
            n1078 = Absolute Value(x=w2083) -> (abs(x)=w2082:dbl)
            n1079 = Less Or Equal?(x=w2080, y=5.0) -> (x <= y?=w2084:bool)
            n1080 = Less Or Equal?(x=w2072, y=8.0) -> (x <= y?=w2085:bool)
            n1081 = Less Or Equal?(x=w2082, y=2.0) -> (x <= y?=w2086:bool)
            n1082 = Compound Arithmetic op=AND(w2086, w2084, w2085) -> (w2067:bool)
          }
          frame "Home Correction" {
            w2132 = 220.0 ("y")
            # "H"
            # "Y"
            # "X"
            # "5mm"
            # "3度"
            # "10mm"
            n1083 = call "Home Correction.vi"() -> ("RL Dist"=w2105:dbl, "Angle out"=w2137:dbl, "Close Range"=w2136:dbl)  [unwired: 9 in]
            n1084 = Subtract(x=w2132, y=w2136) -> (x-y=w2133:dbl)
            n1085 = Absolute Value(x=w2133) -> (abs(x)=w2134:dbl)
            n1086 = shared-variable ".\\Motor Control Variables.lvlib\\Odometry Data"() -> (w2120:dbl[])  [unwired: 1 in, 1 out]
            n1087 = call-poly <vilib>:"PID.vi"("output range"=cluster{"output high":dbl, "output low":dbl} {"output high"=100.0, "output low"=-100.0}, "PID gains"=T6 {"proportional gain (Kc)"=0.2, "integral time (Ti, min)"=0.0, "derivative time (Td, min)"=0.0}, "process variable"=w2136, "setpoint"=w2132) -> ("output"=w2114:dbl)  [unwired: 6 in, 1 out]
            n1088 = Less?(x=w2105, y=30.0) -> (x < y?=w2103:bool)
            n1089 = Divide(x=w2114, y=-100.0) -> (x/y=w2108:dbl)
            n1090 = Add(x=w2137, y=1.5707963267948966) -> (x+y=w2135:dbl)
            n1091 = call-poly <vilib>:"PID.vi"("output range"=cluster{"output high":dbl, "output low":dbl} {"output high"=100.0, "output low"=-100.0}, "PID gains"=T6 {"proportional gain (Kc)"=0.25, "integral time (Ti, min)"=0.0, "derivative time (Td, min)"=0.0}, "process variable"=w2105, "setpoint"=0.0 ("y")) -> ("output"=w2112:dbl)  [unwired: 6 in, 1 out]
            n1092 = Index Array(array=w2120, index=2) -> (element=w2106:dbl)
            n1093 = Divide(x=w2112, y=-100.0) -> (x/y=w2109:dbl)
            n1094 = expression code="(x/pi)*180.0" "radians to degrees"(w2135) -> (w2130:dbl)
            n1095 = Multiply(x=w2135, y=0.7) -> (x*y=w2126:dbl)
            n1096 = Add(x=w2126, y=w2106) -> (x+y=w2101:dbl)
            n1097 = Subtract(x=w2106, y=w2137) -> ()  [unwired: 1 out]
            n1098 = Absolute Value(x=w2130) -> (abs(x)=w2131:dbl)
            n1099 = Less Or Equal?(x=w2134, y=9.0) -> (x <= y?=w2129:bool)
            n1100 = Less Or Equal?(x=w2105, y=9.0) -> (x <= y?=w2128:bool)
            n1101 = Less Or Equal?(x=w2131, y=3.0) -> (x <= y?=w2127:bool)
            n1102 = Compound Arithmetic op=AND(w2127, w2129, w2128) -> (w2107:bool)
            n1103 = Select(t=w2101, s=w2103, f=w2101) -> (s? t:f=w2102:dbl)
          }
          frame "Positioning" {
            w2184 = 1.0 ("y")
            # "補償值"
            n1104 = local read "FXindex"() -> (w2148:i32)
            n1105 = local read "FXArr"() -> (w2155:dbl[])
            n1106 = local read "XL Find"() -> (w2193:dbl)
            n1107 = local read "XL Dots"() -> (w2190:dbl)
            n1108 = local read "XR Dots"() -> (w2189:dbl)
            n1109 = local read "XR Find"() -> (w2192:dbl)
            n1110 = local read "Y Find"() -> (w2194:dbl)
            n1111 = call "WallAngleFind.vi"("End Angle"=50, "Start Angle"=-50) -> ("Angle out"=w2140:dbl, "Y out"=w2167:dbl, "Right Side"=w2175:dbl, "Left Side"=w2174:dbl, "Right Point"=w2187:dbl, "Left Point"=w2176:dbl)  [unwired: 3 in, 1 out]
            "Angle Find" <- w2140
            n1112 = Quotient & Remainder(x=w2148, y=5) -> (x-y*floor(x/y)=w2146:i32)  [unwired: 1 out]
            n1113 = Less?(x=w2167, y=w2194) -> (x < y?=w2195:bool)
            n1114 = Greater?(x=w2174, y=w2193) -> (0:w2191:bool)
            n1115 = Less?(x=w2175, y=w2192) -> (x < y?=w2188:bool)
            n1116 = Select(t=w2167, s=w2195, f=w2194) -> (s? t:f=w2179:dbl)
            n1117 = Select(t=w2174, s=w2191, f=w2193) -> (s? t:f=w2178:dbl)
            n1118 = Select(t=w2175, s=w2188, f=w2192) -> (s? t:f=w2177:dbl)
            n1119 = Index Array(array=w2155, index=w2146) -> (element=w2154:dbl)
            n1120 = Select(t=w2176, s=w2191, f=w2190) -> (s? t:f=w2186:dbl)
            n1121 = Select(t=w2187, s=w2188, f=w2189) -> (s? t:f=w2185:dbl)
            n1122 = local write "XL Find"(w2178) -> ()
            n1123 = local write "XR Find"(w2177) -> ()
            n1124 = local write "Y Find"(w2179) -> ()
            n1125 = local read "Y Find"() -> (w2171:dbl)
            n1126 = local write "XL Dots"(w2186) -> ()
            n1127 = local write "XR Dots"(w2185) -> ()
            n1128 = Add(x=w2171, y=100.0) -> (x+y=w2169:dbl)
            n1129 = local read "FYindex"() -> (w2165:i32)
            n1130 = local read "FYArr"() -> (w2166:dbl[])
            n1131 = Greater?(x=w2185, y=w2184) -> (0:w2172:bool)
            n1132 = Greater?(x=w2186, y=w2184) -> (0:w2173:bool)
            n1133 = Less?(x=w2167, y=w2169) -> (x < y?=w2168:bool)
            n1134 = Select(t=w2178, s=w2173, f=w2177) -> (s? t:f=w2182:dbl)
            n1135 = Select(t=w2177, s=w2172, f=w2178) -> (s? t:f=w2181:dbl)
            n1136 = case shown="True" w2168 {
              tunnel: w2167 -> [_ w2218]
              tunnel: w2165 -> [w2213 w2216]
              tunnel: w2166 -> [w2212 w2215]
              tunnel: [w2212 w2214] -> w2164
              tunnel: [w2213 w2217] -> w2161
              frame False {
              }
              frame True {
                n1137 = Increment(x=w2216) -> (x+1=w2217:i32)
                n1138 = Quotient & Remainder(x=w2216, y=i64 5) -> (x-y*floor(x/y)=w2219:i64)  [unwired: 1 out]
                n1139 = Replace Array Subset(array=w2215, new element=w2218, index=w2219) -> (w2214:dbl[])
              }
            }
            n1140 = Add(x=w2182, y=w2181) -> (x+y=w2183:dbl)
            n1141 = Divide(x=w2183, y=2.0) -> (x/y=w2153:dbl)
            n1142 = Subtract(x=w2153, y=w2154) -> (x-y=w2152:dbl)
            n1143 = Absolute Value(x=w2152) -> (abs(x)=w2151:dbl)
            n1144 = Greater?(x=w2151, y=0.1) -> (0:w2149:bool)
            n1145 = case shown="True" w2149 {
              tunnel: w2153 -> [_ w2209]
              tunnel: [w2204 w2205] -> w2159
              tunnel: w2148 -> [w2204 w2208]
              tunnel: w2155 -> [w2203 w2207]
              tunnel: [w2203 w2206] -> w2156
              frame False {
              }
              frame True {
                n1146 = Increment(x=w2208) -> (x+1=w2205:i32)
                n1147 = Quotient & Remainder(x=w2205, y=i64 5) -> (x-y*floor(x/y)=w2210:i64)  [unwired: 1 out]
                n1148 = Replace Array Subset(array=w2207, new element=w2209, index=w2210) -> (w2206:dbl[])
              }
            }
            n1149 = local write "X Find"(w2153) -> ()
            n1150 = shared-variable ".\\Motor Control Variables.lvlib\\Odometry Data"() -> (w2199:dbl[])  [unwired: 1 in, 1 out]
            n1151 = Sort 1D Array(array=w2156) -> (sorted array=w2157:dbl[])
            n1152 = local write "FXindex"(w2159) -> ()
            n1153 = local write "FYindex"(w2161) -> ()
            n1154 = Sort 1D Array(array=w2164) -> (sorted array=w2163:dbl[])
            n1155 = local write "FXArr"(w2156) -> ()
            n1156 = local write "FYArr"(w2164) -> ()
            n1157 = Index Array(array=w2157, index=3) -> (element=w2143:dbl)
            n1158 = Index Array(array=w2163, index=3) -> (element=w2145:dbl)
            n1159 = Index Array(array=w2199, index=2) -> (element=w2196:dbl)
            n1160 = Negate(x=w2140) -> ()  [unwired: 1 out]
            n1161 = Greater?(x=w2161, y=i64 8) -> (0:w2141:bool)
            n1162 = Add(x=w2145, y=0.0) -> (x+y=→"FY":dbl)
            n1163 = Add(x=w2143, y=0.0) -> (x+y=→"FX":dbl)
          }
          frame "Get Color" {
            # "可以設定成不看顏色,用預設值跑場地"
            n1164 = case shown="False" "Color Disable" {
              tunnel: [w2248 w2249] -> w2231
              tunnel: [w2247 w2251] -> w2230
              tunnel: w2223 -> [w2246 _]
              tunnel: w2221 -> [w2245 _]
              tunnel: w2222 -> [w2244 _]
              frame False {
                n1165 = local read "Proc Block Index"() -> (w2239:i16)
                n1166 = call "TESTC.vi"("error in"=w2244, "Image In"=w2245, "Session In"=w2246) -> ("Image Out"=w2243:T1, "dcolor"=w2247:i32, "ucolor"=w2248:i32, "error out"=w2236:errorcluster)  [unwired: 2 in, 3 out]
                "dcolor" <- w2247
                "ucolor" <- w2248
                "Image Out" <- w2243
                n1167 = Number To Decimal String(number=w2239) -> (decimal integer string=w2238:string)  [unwired: 1 in]
                n1168 = Concatenate Strings("/c/A" ("string"), w2238, ".png" ("string")) -> (w2240:string)
                n1169 = String To Path(string=w2240) -> (path=w2237:path)
                n1170 = call-poly "IMAQ Write File 2"("error in (no error)"=w2236, "File Path"=w2237, "Image"=w2243) -> ()  [unwired: 7 in, 2 out]
              }
              frame True {
                # "關閉顏色讀取狀況下\n使用預設值\n按照大方塊順序為1,2,3,4,5\n                小方塊為2,3,4,5,1"
                n1171 = local read "Proc Block Index"() -> (w2253:i16)
                n1172 = Quotient & Remainder(x=w2253, y=i16 5) -> (x-y*floor(x/y)=w2252:i16)  [unwired: 1 out]
                n1173 = Increment(x=w2252) -> (x+1=w2254:i16)
                n1174 = Quotient & Remainder(x=w2254, y=i16 5) -> (x-y*floor(x/y)=w2250:i16)  [unwired: 1 out]
                n1175 = Increment(x=w2250) -> (x+1=w2249:i16)
                n1176 = Increment(x=w2252) -> (x+1=w2251:i16)
              }
            }
            n1177 = Not Equal To 0?(x=w2231) -> (x != 0?=w2234:bool)
            n1178 = Not Equal To 0?(x=w2230) -> (x != 0?=w2235:bool)
            n1179 = And(x=w2234, y=w2235) -> (x .and. y?=w2225:bool)
            n1180 = case shown="True" w2225 {
              tunnel: w2231 -> [_ w2259]
              tunnel: w2230 -> [_ w2265]
              tunnel: [FALSE FALSE] -> w2224
              frame False {
              }
              frame True {
                w2258 = Operator_Loop_Mode."Idle" ("Operator Loop Mode")
                # "以索引值寫入目標方塊上下顏色"
                n1181 = local read "Down Color"() -> (w2263:i32)
                n1182 = local read "Up Color"() -> (w2262:i32)
                n1183 = Equal To 0?(x=w2263) -> (x = 0?=w2266:bool)
                n1184 = Equal To 0?(x=w2262) -> (x = 0?=w2260:bool)
                n1185 = Select(t=w2265, s=w2266, f=w2263) -> (s? t:f=w2264:i32)
                n1186 = Select(t=w2259, s=w2260, f=w2262) -> (s? t:f=w2261:i32)
                n1187 = local write "Robot Mode:"(w2258) -> ()
                n1188 = shared-variable ".\\Operator Variables.lvlib\\Mode"(w2258) -> ()  [unwired: 1 in, 1 out]
                n1189 = local write "Down Color"(w2264) -> ()
                n1190 = local write "Up Color"(w2261) -> ()
              }
            }
            n1191 = shared-variable ".\\Motor Control Variables.lvlib\\Odometry Data"() -> (w2232:dbl[])  [unwired: 1 in, 1 out]
            n1192 = Index Array(array=w2232, index=2) -> (element=w2227:dbl)
          }
          frame "WhereGo" {
            n1193 = local read "Put Counter"() -> (w2268:i32)
            n1194 = local read "QR_CAM"() -> (w2280:bool)
            n1195 = local read "Block Color"() -> (w2279:i16[][])
            n1196 = local read "Catch Color"() -> (w2278:i16[])
            n1197 = local read "Block Array"() -> (w2270:dbl[][])
            n1198 = call "WhereGo.vi"("QR CODE"=w2280, "Block Array"=w2270, "Catch Color"=w2278, "Put Counter"=w2268, "Block Color"=w2279) -> ("Block Array Out"=w2269:dbl[][], "Proc Block Index"=w2277:i16)  [unwired: 5 in]
            n1199 = local write "Proc Block Index"(w2277) -> ()
            n1200 = local write "Block Array"(w2269) -> ()
            n1201 = shared-variable ".\\Motor Control Variables.lvlib\\Odometry Data"() -> (w2275:dbl[])  [unwired: 1 in, 1 out]
            n1202 = Index Array(array=w2275, index=2) -> (element=w2274:dbl)
          }
          frame "RC Control" {
            n1203 = local read "Proc  VAL A"() -> (w2282:i32)
            n1204 = local read "Proc  VAL B"() -> (w2281:i32)
            n1205 = call "RCservo.vi"("Value"=w2281, "ID"=w2282, "VISA resource name"=w2284) -> ()  [unwired: 7 in, 2 out]
            n1206 = shared-variable ".\\Motor Control Variables.lvlib\\Odometry Data"() -> (w2288:dbl[])  [unwired: 1 in, 1 out]
            n1207 = Index Array(array=w2288, index=2) -> (element=w2287:dbl)
          }
          frame "MoveTarget" {
            w2292 = 0.15 ("upper limit")
            w2308 = 1000.0 ("y")
            w2326 = 1000.0 ("y")
            # "超音波差距在５公分內取平均，不然就拿最小的"
            # "Y動作限制在＋－３ｃｍ"
            # "移動150mm內,都使用超音波"
            # "以Offset移動"
            # "Y"
            n1208 = local read "UltraSound"() -> (w2294:dbl)
            n1209 = shared-variable ".\\Motor Control Variables.lvlib\\Odometry Data"() -> (w2338:dbl[])  [unwired: 1 in, 1 out]
            n1210 = local read "Proc  VAL B"() -> (w2300:i32)
            n1211 = shared-variable ".\\Operator Variables.lvlib\\SubGoal"() -> (w2309:dbl[])  [unwired: 1 in, 1 out]
            n1212 = local read "Proc  VAL A"() -> (w2315:i32)
            n1213 = local read "BL Range"() -> (w2325:dbl)
            n1214 = Index Array(array=w2338) -> (element #1=w2328:dbl, element #2=w2327:dbl, element #3=w2295:dbl)  [unwired: 3 in]
            n1215 = Index Array(array=w2309) -> (element #1=w2306:dbl, element #2=w2307:dbl, element #3=w2296:dbl)  [unwired: 3 in]
            n1216 = Absolute Value(x=w2300) -> (abs(x)=w2303:i32)
            n1217 = Greater?(x=w2303, y=30) -> (0:w2301:bool)
            n1218 = Multiply(x=w2326, y=w2327) -> (x*y=w2317:dbl)
            n1219 = Multiply(x=w2328, y=w2326) -> (x*y=w2318:dbl)
            n1220 = Multiply(x=w2306, y=w2308) -> (x*y=w2305:dbl)
            n1221 = Multiply(x=w2308, y=w2307) -> (x*y=w2304:dbl)
            n1222 = Select(t=0, s=w2301, f=w2300) -> (s? t:f=w2298:i32)
            n1223 = Subtract(x=w2325, y=w2298) -> (x-y=w2323:dbl)
            n1224 = Subtract(x=w2294, y=w2323) -> (x-y=w2322:dbl)
            n1225 = call-poly <vilib>:"2D Cartesian Coordinate Rotation.vi"("theta"=w2296, "y"=w2304, "x"=w2305) -> ("x out"=w2312:dbl)  [unwired: 6 in, 2 out]
            n1226 = call-poly <vilib>:"2D Cartesian Coordinate Rotation.vi"("theta"=w2296, "y"=w2317, "x"=w2318) -> ("x out"=w2313:dbl)  [unwired: 6 in, 2 out]
            n1227 = Add(x=w2315, y=w2312) -> (x+y=w2316:dbl)
            n1228 = Subtract(x=w2316, y=w2313) -> (x-y=w2314:dbl)
            n1229 = Subtract(x=w2313, y=w2312) -> (x-y=w2311:dbl)
            n1230 = Absolute Value(x=w2311) -> (abs(x)=w2337:dbl)
            n1231 = Less Or Equal?(x=w2337, y=100.0) -> (x <= y?=w2297:bool)
            n1232 = Select(t=w2322, s=w2297, f=0.0) -> (s? t:f=w2330:dbl)
            n1233 = Subtract(x=w2323, y=w2330) -> (x-y=w2342:dbl)
            n1234 = call-poly <vilib>:"PID.vi"("reinitialize? (F)"=w2310, "output range"=cluster{"output high":dbl, "output low":dbl} {"output high"=100.0, "output low"=-100.0}, "PID gains"=T6 {"proportional gain (Kc)"=0.23, "integral time (Ti, min)"=0.0, "derivative time (Td, min)"=0.0}, "process variable"=w2330, "setpoint"=0.0) -> ("output"=w2345:dbl)  [unwired: 5 in, 1 out]
            n1235 = Divide(x=w2345, y=-100.0) -> (x/y=w2331:dbl)
            n1236 = call-poly <vilib>:"PID.vi"("output range"=cluster{"output high":dbl, "output low":dbl} {"output high"=100.0, "output low"=-100.0}, "PID gains"=T6 {"proportional gain (Kc)"=0.25, "integral time (Ti, min)"=0.0, "derivative time (Td, min)"=0.0001}, "process variable"=w2314, "setpoint"=0.0) -> ("output"=w2333:dbl)  [unwired: 6 in, 1 out]
            n1237 = Divide(x=w2333, y=-60.0) -> (x/y=w2290:dbl)
            n1238 = Absolute Value(x=w2342) -> (abs(x)=w2340:dbl)
            n1239 = Absolute Value(x=w2314) -> (abs(x)=w2329:dbl)
            n1240 = Negate(x=w2292) -> (-x=w2293:dbl)
            n1241 = Less Or Equal?(x=w2329, y=3.0) -> (x <= y?=w2320:bool)
            n1242 = Less Or Equal?(x=w2340, y=3.0) -> (x <= y?=w2339:bool)
            n1243 = In Range and Coerce(upper limit=w2292, x=w2290, lower limit=w2293) -> (coerced(x)=w2291:dbl)  [unwired: 1 out]
            n1244 = Compound Arithmetic op=AND(w2320, w2339) -> ()  [unwired: 1 out]
          }
          frame "moveblock" {
            w2350 = 0.15 ("upper limit")
            w2371 = 1000.0 ("y")
            w2387 = 1000.0 ("y")
            # "白暗F"
            # "超音波差距在５公分內取平均，不然就拿最小的"
            # "Y動作限制在＋－３ｃｍ"
            # "移動150mm內,都使用超音波"
            # "以Offset移動"
            # "Y"
            n1245 = local read "UltraSound"() -> (w2357:dbl)
            n1246 = local read "Proc  VAL B"() -> (w2363:i32)
            n1247 = shared-variable ".\\Motor Control Variables.lvlib\\Odometry Data"() -> (w2399:dbl[])  [unwired: 1 in, 1 out]
            n1248 = shared-variable ".\\Operator Variables.lvlib\\SubGoal"() -> (w2372:dbl[])  [unwired: 1 in, 1 out]
            n1249 = local read "Proc  VAL A"() -> (w2377:i32)
            n1250 = local read "BL Range"() -> (w2386:dbl)
            n1251 = Index Array(array=w2399) -> (element #1=w2389:dbl, element #2=w2388:dbl, element #3=w2358:dbl)  [unwired: 3 in]
            n1252 = Index Array(array=w2372) -> (element #1=w2369:dbl, element #2=w2370:dbl, element #3=w2359:dbl)  [unwired: 3 in]
            n1253 = Absolute Value(x=w2363) -> (abs(x)=w2366:i32)
            n1254 = Greater?(x=w2366, y=30) -> (0:w2364:bool)
            n1255 = Multiply(x=w2387, y=w2388) -> (x*y=w2379:dbl)
            n1256 = Multiply(x=w2389, y=w2387) -> (x*y=w2380:dbl)
            n1257 = Multiply(x=w2369, y=w2371) -> (x*y=w2368:dbl)
            n1258 = Multiply(x=w2371, y=w2370) -> (x*y=w2367:dbl)
            n1259 = Select(t=0, s=w2364, f=w2363) -> (s? t:f=w2361:i32)
            n1260 = Subtract(x=w2386, y=w2361) -> (x-y=w2384:dbl)
            n1261 = Subtract(x=w2357, y=w2384) -> (x-y=w2383:dbl)
            n1262 = call-poly <vilib>:"2D Cartesian Coordinate Rotation.vi"("theta"=w2359, "y"=w2367, "x"=w2368) -> ("x out"=w2375:dbl)  [unwired: 6 in, 2 out]
            n1263 = call-poly <vilib>:"2D Cartesian Coordinate Rotation.vi"("theta"=w2359, "y"=w2379, "x"=w2380) -> ("x out"=w2376:dbl)  [unwired: 6 in, 2 out]
            n1264 = Add(x=w2377, y=w2375) -> (x+y=w2378:dbl)
            n1265 = Subtract(x=w2378, y=w2376) -> (x-y=w2353:dbl)
            "nowpos" <- w2353
            n1266 = Subtract(x=w2376, y=w2375) -> (x-y=w2374:dbl)
            n1267 = Absolute Value(x=w2374) -> (abs(x)=w2398:dbl)
            n1268 = Less Or Equal?(x=w2398, y=100.0) -> (x <= y?=w2360:bool)
            n1269 = Select(t=w2383, s=w2360, f=0.0) -> (s? t:f=w2391:dbl)
            n1270 = Subtract(x=w2384, y=w2391) -> (x-y=w2402:dbl)
            n1271 = call-poly <vilib>:"PID.vi"("reinitialize? (F)"=w2373, "output range"=cluster{"output high":dbl, "output low":dbl} {"output high"=100.0, "output low"=-100.0}, "PID gains"=T6 {"proportional gain (Kc)"=0.25, "integral time (Ti, min)"=0.0, "derivative time (Td, min)"=0.0}, "process variable"=w2391, "setpoint"=0.0) -> ("output"=w2405:dbl)  [unwired: 5 in, 1 out]
            n1272 = local read "B/DIO0 (Pin 11)"() -> (w2354:bool)
            n1273 = Divide(x=w2405, y=-100.0) -> (x/y=w2392:dbl)
            n1274 = call-poly <vilib>:"PID.vi"("output range"=cluster{"output high":dbl, "output low":dbl} {"output high"=100.0, "output low"=-100.0}, "PID gains"=T6 {"proportional gain (Kc)"=0.25, "integral time (Ti, min)"=0.0, "derivative time (Td, min)"=0.0001}, "process variable"=w2353, "setpoint"=0.0) -> ("output"=w2394:dbl)  [unwired: 6 in, 1 out]
            n1275 = Divide(x=w2394, y=-200.0) -> (x/y=w2348:dbl)
            n1276 = Absolute Value(x=w2402) -> (abs(x)=w2400:dbl)
            n1277 = Absolute Value(x=w2353) -> (abs(x)=w2390:dbl)
            n1278 = Negate(x=w2350) -> (-x=w2351:dbl)
            n1279 = In Range and Coerce(upper limit=w2350, x=w2348, lower limit=w2351) -> (coerced(x)=w2349:dbl)  [unwired: 1 out]
            n1280 = Less Or Equal?(x=w2390, y=3.0) -> (x <= y?=w2352:bool)
            n1281 = Less Or Equal?(x=w2400, y=2.0) -> ()  [unwired: 1 out]
            n1282 = Compound Arithmetic op=AND(w2352, w2352) -> (w2356:bool)
            n1283 = Or(x=w2356, y=w2354) -> (x .or. y?=w2355:bool)
          }
          frame "hands up" {
            w2422 = 1.0 ("ID")
            w2421 = 0.0 ("ID")
            n1284 = call "RC_MoveTable.vi"("Index"=w2422, "ID"=w2421, "CMD"=2.0) -> ("Value"=w2411:i32, "RC ID"=w2412:i32)  [unwired: 6 in]
            n1285 = call "RC_MoveTable.vi"("Index"=w2422, "ID"=w2422, "CMD"=2.0) -> ("Value"=w2409:i32, "RC ID"=w2410:i32)  [unwired: 6 in]
            n1286 = call "RC_MoveTable.vi"("Index"=w2422, "ID"=w2422, "CMD"=3.0) -> ("Value"=w2413:i32, "RC ID"=w2414:i32)  [unwired: 6 in]
            n1287 = call "RC_MoveTable.vi"("Index"=w2422, "ID"=w2421, "CMD"=3.0) -> ("Value"=w2415:i32, "RC ID"=w2416:i32)  [unwired: 6 in]
            n1288 = call "RCservo.vi"("Value"=w2415, "ID"=w2416, "VISA resource name"=w2408) -> ()  [unwired: 7 in, 2 out]
            n1289 = call "RCservo.vi"("Value"=w2413, "ID"=w2414, "VISA resource name"=w2408) -> ()  [unwired: 7 in, 2 out]
            n1290 = call "RCservo.vi"("Value"=w2411, "ID"=w2412, "VISA resource name"=w2408) -> ()  [unwired: 7 in, 2 out]
            n1291 = call "RCservo.vi"("Value"=w2409, "ID"=w2410, "VISA resource name"=w2408) -> ()  [unwired: 7 in, 2 out]
          }
          frame "hands down" {
            n1292 = call "RCservo.vi"("Value"=1835, "ID"=20, "VISA resource name"=w2425) -> ("VISA resource name out"=w2424:refnum<visa-resource-name>)  [unwired: 7 in, 1 out]
            n1293 = call "RCservo.vi"("Value"=1200, "ID"=10, "VISA resource name"=w2424) -> ()  [unwired: 7 in, 2 out]
          }
          frame "readQR" {
            n1294 = local write "Light"(0.7 ("Light")) -> ()
            n1295 = call "GetQR_A.vi"("error in"=w2436, "Image In"=w2437, "Session In"=w2438) -> ("QR_OK"=w2433:bool, "QR_CODE"=w2432:string, "Image Out"=w2435:T1)  [unwired: 5 in, 1 out]
            n1296 = local write "Image Out"(w2435) -> ()
            n1297 = case shown="True" w2433 {
              tunnel: w2432 -> [_ w2445]
              frame False {
              }
              frame True {
                w2446 = Operator_Loop_Mode."Idle" ("Operator Loop Mode")
                n1298 = call "QR2POS.vi"("QR_string"=w2445) -> ("Start Out Point"=w2447:dbl[], "Start Front"=w2448:dbl[], "Start POS"=w2449:dbl[], "heading"=w2450:dbl, "Block Array"=w2451:dbl[][])  [unwired: 5 in, 1 out]
                n1299 = local write "Start POS"(w2449) -> ()
                n1300 = local write "Start Out Point"(w2447) -> ()
                n1301 = local write "Heading(rad)"(w2450) -> ()
                n1302 = local write "Start Front"(w2448) -> ()
                n1303 = local write "Block Array"(w2451) -> ()
                n1304 = local write "Robot Mode:"(w2446) -> ()
                n1305 = shared-variable ".\\Operator Variables.lvlib\\Mode"(w2446) -> ()  [unwired: 1 in, 1 out]
                n1306 = local write "Light"(0.0 ("Light")) -> ()
              }
            }
            n1307 = shared-variable ".\\Motor Control Variables.lvlib\\Odometry Data"() -> (w2442:dbl[])  [unwired: 1 in, 1 out]
            n1308 = Index Array(array=w2442, index=2) -> (element=w2439:dbl)
          }
        }
        n1309 = local read "stop"() -> (w1928:bool)
        n1310 = Select(t=FALSE, s=w1914, f=w1918) -> (s? t:f=w1913:bool)
        n1311 = case shown="True" "Show VFH" {
          frame False {
          }
          frame True {
            # "顯示自動避障圖"
            n1312 = call "VFH Visualization.vi"() -> ("Heading History"=→"Heading History 2":dbl, "VY History"=→"VY History 2":dbl, "LIDAR data"=→"LIDAR data":cluster{dbl[], dbl[]}[])  [unwired: 7 in]
          }
        }
        n1313 = shared-variable ".\\Motor Control Variables.lvlib\\VX_Cmd"(w1919) -> ()  [unwired: 1 in, 1 out]
        n1314 = shared-variable ".\\Motor Control Variables.lvlib\\Heading_Cmd"(w1921) -> ()  [unwired: 1 in, 1 out]
        n1315 = shared-variable ".\\Motor Control Variables.lvlib\\VY_Cmd"(w1920) -> ()  [unwired: 1 in, 1 out]
        n1316 = local write "Proc Finish"(w1913) -> ()
        n1317 = node-c288() -> ()  [unwired: 1 in, 1 out]
      }
      n1318 = node-c288(w485) -> ()  [unwired: 1 out]
      n1319 = node-c288(w477) -> ()  [unwired: 1 out]
      n1320 = node-c288(w499) -> ()  [unwired: 1 out]
      n1321 = node-c288(i64 200 ("Period")) -> (w469:T20)  [unwired: 3 in]
      n1322 = timed-loop {
        shift-right: [w641] -> _
        shift-left: _ -> [w644]
        shift-right: [w639] -> _
        shift-left: _ -> [w643]
        timing: w469 -> [_]
        timing-out: [_] -> w468
        shift-right: [w621] -> _
        shift-left: _ -> [w628]
        stop <- w635 stop-if-true
        # "當在Path Following模式下\n目標的距離比已經紀錄的還要遠\n就開始累加秒數,否則就把秒數歸零"
        # "時間計時功能"
        n1323 = node-c288() -> ()  [unwired: 1 in, 1 out]
        n1324 = local read "Target Distance"() -> (w632:dbl)
        n1325 = local read "min Distance"() -> (w631:dbl)
        n1326 = local read "Robot Mode:"() -> (w630:T5)
        n1327 = local read "Timer Run"() -> (w636:bool)
        n1328 = Greater?(x=w632, y=w631) -> (0:w624:bool)
        n1329 = Equal?(x=w630, y=Operator_Loop_Mode."Path Following" ("Operator Loop Mode")) -> (x = y?=w623:bool)
        n1330 = And(x=w624, y=w623) -> (x .and. y?=w622:bool)
        n1331 = Get Date/Time In Seconds() -> (seconds since 1Jan1904=w642:timestamp)
        n1332 = To Double Precision Float(number=w642) -> (double precision float=w641:dbl)
        n1333 = Subtract(x=w641, y=w644) -> (x-y=w627:dbl)
        n1334 = Add(x=w627, y=w628) -> (x+y=w625:dbl)
        n1335 = Select(t=w625, s=w622, f=0.0) -> (s? t:f=w621:dbl)
        "GoFarSec" <- w621
        n1336 = Add(x=w627, y=w643) -> (x+y=w637:dbl)
        n1337 = Select(t=w637, s=w636, f=u64 0 ("t")) -> (s? t:f=w639:dbl)
        n1338 = Quotient & Remainder(x=w639, y=u64 60 ("t")) -> (x-y*floor(x/y)=→"SEC":dbl, floor(x/y)=w633:dbl)
        "MIN" <- w633
        n1339 = local write "MIN"(w633) -> ()
        n1340 = local read "stop"() -> (w635:bool)
        n1341 = node-c288() -> ()  [unwired: 1 in, 1 out]
      }
      n1342 = Merge Errors(w492, w482) -> (w483:errorcluster)
      n1343 = node-c288(w490) -> ()  [unwired: 1 out]
      n1344 = node-c288(w468) -> ()  [unwired: 1 out]
    }
    frame #5 {
      # "Close"
      n1345 = call <vilib>:"IMAQdx Close Camera.vi"("error in"=w2684, "Session In"=w2685) -> ("error out"=w2686:errorcluster)  [unwired: 9 in]
      n1346 = call "Imaq Dispose"("All Images? (No)"=TRUE, "error in (no error)"=w2686) -> ()  [unwired: 4 in, 1 out]
      n1347 = VISA Flush I/O Buffer(VISA resource name=w2689) -> (VISA resource name out=w2688:refnum<visa-resource-name>)  [unwired: 2 in, 1 out]
      n1348 = call <vilib>:"Reset myRIO.vi"("error in (no error)"=w2690) -> ("error out"=→"error out":errorcluster)  [unwired: 10 in]
      n1349 = call "URG-04LX-UG01 Close.vi"("VISA Refnum in"=w2688) -> ()  [unwired: 10 in, 1 out]
    }
  }
